vi "PIV_Stats_Single_with_Check.vi"(0 "Data Folder":path=path "C:/Users/PIV/Documents/mike_ensight/NACA0015_MB_G/15ms_PLANE_B_PA_300/rear", 1 "PIV Meas Plane":enum16{"XY", "YZ", "XZ"}(ring)=enum."XZ", 2 "Row number":i32=1, 5 "Output Directory":path=path "C:/Users/PIV/Documents/mike_ensight/NACA0015_MB_G/15ms_PLANE_B_PA_300/rear", 7 "XYZ Translation":dbl[](array[numeric])=[0.0, 0.0, 0.0], 9 "Case Name":string="ensight", 11 "PIV Freq (Hz)":dbl=7.25, 12 "Invert U":bool=TRUE, 13 "Invert V":bool, 14 "Kurt Tolerance":dbl=2.0) -> (4 "Progress Bar":i32(slide)=98 scale=0.0..100.0, 6 "Status":string="Wrting the data to file...", 10 "# total vectors":i32=10235)   [LabVIEW 2022 SP3]
uses:
  <vilib>/Utility/error.llb/DialogType.ctl
  <vilib>/Analysis/1siggen.llb/Ramp Pattern by Samples.vi
  <vilib>/Utility/error.llb/Trim Whitespace One-Sided.vi
  <vilib>/Analysis/NI_AALBase.lvlib
panel:
  out "interpolated vetors %":dbl[][](array[numeric])=[[15.76889236484505], [16.860635696821515], [16.77103718199609], [19.11750317972801], [17.901838091513493], [19.95502542041455], [17.47335484501809], [19.833822091886606], [17.568228504352927], [19.048084440969507], [19.503129890453835], [18.20848816741639], [19.704818688300264], [16.888323880305105], [18.985238048685112], [19.086731201720937], [19.43874058863792], [20.062603932309496], [18.812946123007723], [16.77097594367299], [18.17114914425428], [17.349232724073893], [20.437884859740006], [18.84596577017115], [17.522245037645447], [16.37484104470312], [17.813844348846306], [15.853300733496333], [17.204616588419405], [17.514179542343047], [17.895560336397416], [17.282502443792765], [19.48978594467794], [19.409406473061505], [15.101721439749607], [19.047153198982585], [20.273838630806846], [18.624669862075713], [16.686217008797655], [19.910033248582046], [17.447432762836186], [19.52292501710822], [18.057321725520882], [17.794290183809153], [18.836185819070906], [21.9538431449247], [19.12771367103462], [18.779342723004692], [19.080684596577015], [17.11324075884999], [18.96989835809226], [19.661712944857253], [17.548147423990613], [18.355173088206534], [19.303735575982788], [18.40226850493791], [19.730020541915287], [19.192412983965585], [15.809542432538132], [18.797066014669927], [16.179489686186333], [19.215724623508702], [20.629644114196324], [17.93116933906922], [21.66601486116543], [17.78973105134474], [18.141809290953546], [18.83987087938961], [17.193154034229828], [18.425427872860638], [19.253322908522282], [17.072455265473746], [19.196166634070018], [19.11189358372457], [19.732212666145426], [20.89566832893322], [19.980440097799512], [19.622604614782947], [19.311626087806786], [19.655779385879132], [16.301584197144532], [18.671752738654146], [15.97887737140622], [19.530562347188262], [19.66363547472377], [20.829664416397613], [16.601486116542823], [16.992760712189394], [17.893810501613377], [18.24581988853036], [17.78973105134474], [17.86098347834588], [17.78973105134474], [17.41001564945227], [17.850156494522693], [19.681267109894407], [18.73472181480395], [21.938575899843503], [19.033646322378715], [19.186387639350674], [17.31859964795619], [17.96752738654147], [19.69682151589242], [18.45115869756527], [19.102112676056336], [18.613067292644757], [17.709759436729904], [19.551815246110188], [17.30543605788033], [19.72809076682316], [16.93075117370892], [17.594132029339853], [17.77190923317684], [20.385217051231912], [19.26461959710542], [18.672401994329846], [19.91392801251956], [16.23154395228317], [17.58381389893461], [15.446280183791181], [18.061803246626244], [16.744868035190617], [18.525760093850817], [17.470409860119336], [18.382712427886965], [17.205982989539546], [15.335744306519402], [17.284554436075517], [19.13562139434829], [15.350019554165037], [17.535452322738386], [17.87775061124694], [18.39710343477835], [16.475994915419967], [18.69012707722385], [18.228046156855076], [18.21292403949555], [18.4841075794621], [16.744868035190617], [17.404908575339785], [16.477606102092704], [19.155177471399238], [16.891627543035995], [19.15330465389128], [15.395148669796557], [16.83129584352078], [15.180840664711631], [18.634451726499073], [15.529043614316448], [17.396831605710933], [16.927439859182474], [20.05475701574264], [19.317292644757433], [17.39853300733496], [17.240367690201445], [16.317950723504108], [19.3097379741885], [17.056234718826406], [19.3138500635324], [16.695992179863147], [16.347281971059836], [17.157390198571846], [17.117997849252127], [17.041454829878763], [17.015450811656564], [17.597028057483623], [17.059571554338255], [17.588971450919047], [18.4627420301193], [18.077825576847868], [17.58091326879828], [16.572154868987095], [19.052281182690425], [17.87775061124694], [17.80299325051355], [18.21826716213573], [18.3080684596577], [18.710876369327075], [19.27215809039327], [19.72051206879703], [19.921760391198042], [18.24403597966367], [19.72423234891453], [15.3199804592086], [16.674816625916872], [16.570534754130414], [17.03500880109525], [18.68583162217659], [16.901270772238515], [18.910726508262442], [17.408748409824838], [18.578273198396403], [17.970277669143528], [18.99872885499169], [21.344028171769537], [19.526742935367164], [21.466992665036674], [19.835680751173708], [16.83778234086242], [18.54712553773954], [17.253176930596286], [18.63147605083089], [18.648542929786817], [19.033646322378715], [17.03500880109525], [19.061124694376527], [17.418092909535453], [19.13562139434829], [18.521415998435362], [19.90804147916259], [17.784513101290575], [20.27185605319773], [16.47438404380133], [18.333822235259607], [17.155712050078247], [18.580089966751416], [18.459131795072352], [15.453834115805948], [17.59874853343762], [16.863934265871077], [17.800176142479696], [16.863818555088475], [17.311827956989248], [17.727583846680357], [17.946210268948658], [19.180760582657154], [19.683191551774716], [17.917888563049853], [20.86429409464216], [21.878971551471306], [15.705065519264618], [18.638763935067477], [18.72739712638061], [19.74982898465748], [18.00762537882491], [17.647058823529413], [17.874254424562434], [19.739802406338647], [18.43417065780471], [17.437200664646664], [17.852952678920612], [17.64360504941775], [17.750611246943766], [17.874254424562434], [17.916870415647924], [18.86976926085256], [17.11324075884999], [19.081133919843598], [16.035983181773737], [19.767214397496087], [18.37113805240516], [18.18092909535452], [17.330073349633253], [18.031665363565285], [21.255377395385217], [17.061008994915916], [18.806845965770172], [19.315403422982886], [18.615565115369574], [16.559076682316118], [17.602190494817133], [15.735941320293398], [19.3236242791516], [18.736553882260903], [17.475063563465675], [20.082127493156044], [17.285881892843175], [20.16428711128496], [16.264058679706604], [17.944455309994133], [18.732890105592492], [19.088151844242248], [19.34474327628362], [18.116933906922174], [19.14768839800606], [21.071673022391707], [16.199041939583537], [18.748166259168705], [19.50122249388753], [19.26049104959405], [16.738365271802895], [18.34001368657738], [19.061124694376527], [19.13562139434829], [19.585613760750586], [13.806590397966168], [17.269704674359478], [18.765890866418932], [17.905339331116764], [19.098376686876588], [19.888584831899923], [18.167595580326587], [19.346635367762126], [17.93743890518084], [18.859992178333982], [18.32225263981228], [17.175273865414713], [17.594132029339853], [21.550796910139827], [19.675337375317817], [19.9745795854517], [17.489490663799003], [17.597028057483623], [20.565225894778017], [17.530308955807588], [17.732160312805473], [17.74997556446095], [18.715165737753008], [19.61071987480438], [18.376528117359413], [19.511002444987774], [17.846665362800703], [17.036674816625915], [18.672401994329846], [17.70171149144254], [21.95718056506012], [18.378325508607197], [17.779298211318544], [18.45115869756527], [18.919976521228723], [20.117359413202934], [18.040481079495454], [16.73185996479562], [19.538431449247017], [18.728606356968218], [20.350259270130124], [19.403422982885086], [21.09122909944265], [18.34620271723194], [17.928403755868544], [18.18092909535452], [18.332029722330855], [19.943298465148107], [22.793470823966377], [18.34360027378508], [20.62762733405025], [18.61738535249829], [17.86098347834588], [17.132798748288675], [17.196206862840942], [21.914727166047328], [14.947697722162479], [15.304126735771561], [20.660995404321895], [19.66940532081377], [16.668296021116433], [15.213140398904967], [18.66379731976915], [18.029739776951672], [19.9745795854517], [18.912575787209075], [17.682151589242054], [17.44402072944167], [17.805808154884133], [19.692969590300187], [20.61008994915917], [20.428319968707218], [20.316932407316834], [20.152462861610633], [17.095354523227385], [19.796656564669078], [18.82145998240985], [18.58260019550342], [18.43417065780471], [17.052899188422803], [18.29113305308437], [16.335907713363966], [19.471882640586795], [18.873459808331702], [20.506799726054204], [20.774647887323944], [16.995892822217876], [17.378555370931483], [17.704565451168246], [19.362409544298846], [16.679702776691435], [17.47335484501809], [19.74572127139364], [19.206333691721237], [19.086731201720937], [18.099149310648283], [20.04304020346278], [17.628079780993353], [19.245061607666734], [20.81377151799687], [18.90279679248973], [17.227219397731716], [18.228046156855076], [19.75755205787467], [19.145399432873766], [18.90094846973697], [18.190709046454767], [19.178885630498534], [19.042033235581624], [17.743669957962656], [18.37473107764522], [17.963252541047694], [17.39853300733496], [18.413847056522588], [19.763348327791903], [18.490270851667155], [18.787286063569685], [20.867950346984653], [18.49281595151989], [16.904575674618695], [18.58372456964006], [18.274310311093718], [17.887530562347187], [19.69874804381847], [16.370037160179933], [18.66314347230378], [17.079135283184975], [19.534383253448105], [18.054740957966764], [20.440097799511005], [21.149335418295543], [17.499755453389415], [17.452092295658975], [18.888780201506407], [18.130256209661646], [19.249193469547365], [18.702924777462584], [17.767787333854574], [18.11069822022296], [16.555838059847446], [18.613745234138236], [19.497408819790753], [20.228783730934687], [17.86622335223939], [17.49633251833741], [20.891582754912505], [18.69743790338353], [18.560531977312735], [18.07158224134559], [21.411810715682442], [20.602327173169062], [20.312805474095796], [20.739219712525667], [17.956989247311828], [20.39898298454919], [18.723113023073914], [17.535452322738386], [16.753056234718827], [19.824046920821115], [18.035190615835777], [17.988073125427707], [19.87875232228415], [18.24139280125196], [18.715793588741203], [19.577340769004987], [20.41454829878764], [20.058651026392962], [19.9119804400978], [20.45387850924386], [19.552034428794993], [20.097751710654936], [17.038341158059467], [17.32499022291748], [18.571009676473462], [18.65401545534579], [20.035218156916454], [18.608746697974755], [18.689486552567235], [17.492910922069033], [17.35981994324298], [19.092331768388107], [17.507824726134587], [17.42105777690879], [18.456572769953052], [17.519319182236135], [20.583056153394637], [19.960899315738025], [17.404908575339785], [17.452092295658975], [17.77299833805846], [18.66875183266543], [20.156479217603913], [18.75794621026895], [17.165200391006845], [18.464547677261614], [16.239734063355495], [18.397887323943664], [18.585542404382274], [16.31774603795735], [18.59601095033242], [19.50909446508899], [19.61839530332681], [20.013694610192704], [17.93467631527479], [19.46781451770691], [18.842845973416733], [19.970660146699267], [19.661547490951776], [20.01173708920188], [17.32329650992277], [17.194525904203324], [18.394289067083903], [17.039788835663312], [18.974960876369327], [21.02589154860772], [17.850156494522693], [19.375978090766825], [19.976521228722362], [18.593505477308295], [19.558205454012313], [18.383719792583896], [17.42105777690879], [17.284554436075517], [20.357876210032266], [18.441380659039798], [17.685013197771042], [16.725352112676056], [17.999608916699255], [18.996380710163358], [17.113502935420744], [19.454225352112676], [17.900087985140285], [19.158924205378973], [19.244692300166324], [20.751026794445533], [16.903061723564512], [19.804496578690127], [18.955909668589303], [16.606321557882374], [16.823069403714566], [17.376856919468334], [18.418222700166194], [18.361360969886587], [18.68765890866419], [16.37484104470312], [16.754694835680752], [20.195599022004888], [19.405320813771517], [17.202933985330073], [16.927439859182474], [19.859196245233207], [22.610312102534], [17.74997556446095], [17.352624890018575], [18.286720125171133], [20.944558521560573], [20.0352009386917], [16.413968502396557], [18.96703511689328], [18.456572769953052], [19.466432131339783], [18.93716970052848], [20.36566288619476], [18.341806804849433], [17.438905180840663], [17.015450811656564], [16.47921760391198], [19.524833789597185], [20.952287837309346], [17.84492030898602], [17.970277669143528], [20.819880637902358], [18.754277891854894], [20.445878556761514], [17.774736018771996], [19.30596285434995], [18.083961248654468], [20.291414042636415], [21.10872115760657], [19.114196323816973], [17.74083129584352], [19.9041939583537], [18.413847056522588], [17.884032463087905], [20.316777473601878], [19.180760582657154], [19.319182236134207], [17.137550102649328], [18.688845401174166], [19.43276283618582], [17.962256771291678], [17.66718811106766], [18.811106765741105], [19.08904310429088], [18.918125794776483], [18.540973987874047], [18.228046156855076], [19.07463562555023], [18.894865525672373], [16.441837732160312], [18.448596302455247], [17.67523707107244], [17.79495206417531], [17.525672371638144], [20.217030012708964], [15.66536203522505], [20.88223787167449], [18.855745721271393], [17.196206862840942], [17.561357191747334], [16.916006649066198], [18.2200488997555], [17.900087985140285], [17.97906681013401], [17.561882398982487], [18.752444270629645], [16.528036011351404], [18.55438184663537], [18.778103616813294], [16.33750488854126], [20.3991781626064], [18.635119280406727], [19.05134474327628], [16.779114109709592], [18.947985921001173], [17.80058651026393], [19.86897428375868], [19.17245426978382], [18.552567237163814], [18.271580799687165], [20.39898298454919], [16.839428906708388], [17.947214076246336], [19.36840046929996], [19.741859782927545], [19.33118216485773], [17.87075960504448], [18.394289067083903], [16.552600703949942], [17.207665232694563], [16.554219223623743], [16.982792334767304], [20.39319248826291], [19.97653270753887], [16.314760508308897], [18.998239092154176], [20.4950107611035], [18.120477214942305], [20.73552425665102], [17.04312114989733], [17.134474327628364], [17.369193154034228], [20.232853928187065], [17.389177023192094], [15.833740831295842], [16.195599022004888], [19.107719401232757], [19.90414710485133], [18.320461433180174], [17.392154944732464], [18.744499853329422], [18.20492764958936], [17.336855493591624], [18.035190615835777], [17.944455309994133], [16.169713559487732], [17.334767305436056], [19.157050655192645], [16.687848274513637], [17.832338843783624], [17.58607198748044], [18.2920864716815], [17.725850606179115], [16.964896841693555], [13.423344095489679], [17.139503032674625], [17.230588695482105], [17.21744231521314], [17.748875415607277], [17.15067957367752], [17.93116933906922], [16.352262730915847], [16.65199960887846], [19.098376686876588], [17.804067266327728], [16.775897486060842], [18.155140369754474], [16.39921722113503], [18.191593352883675], [17.3657964212379], [18.539161044294513], [18.77750611246944], [18.68765890866419], [18.77750611246944], [17.962256771291678], [19.090909090909093], [15.611855619681112], [18.877151799687013], [16.977995110024448], [18.47432762836186], [20.25625978090767], [18.840438013296833], [18.73105875452146], [17.22754842496576], [19.66363547472377], [18.910726508262442], [18.490270851667155], [19.006648416112633], [18.720657276995308], [18.677879913944846], [17.549863120844737], [15.50880626223092], [18.96889062805713], [16.73349633251834], [16.1861010653895], [17.693661971830984], [18.190709046454767], [17.08866946915632], [15.605749486652979], [16.050469483568076], [18.646719468074703], [18.80258266484054], [18.431602620514326], [17.22586324953536], [15.487721357988454], [17.11324075884999], [17.751710654936463], [17.44402072944167], [18.501125134526955], [16.992952231793264], [17.659137577002053], [17.629803461425638], [15.108546841384706], [19.38196753373753], [18.052976248656044], [16.49555099247091], [17.792550591455665], [17.498043818466353], [20.03325833903942], [18.609426950909448], [18.11069822022296], [17.969284945710655], [17.721271393643033], [17.964013299432818], [18.754277891854894], [17.111567419575632], [19.78097193702943], [16.83129584352078], [19.231145456323976], [19.614556838192136], [18.47432762836186], [16.749779994133178], [17.825364231935072], [18.07252467989444], [16.052400039104505], [19.538431449247017], [17.541801114696394], [16.819960861056753], [16.311363191863876], [19.000097837784953], [16.412363067292645], [17.737990411897076], [17.23531136963535], [18.854461929430162], [21.517254863623034], [18.426197458455523], [17.667775386421443], [15.67726161369193], [16.955118803168084], [18.10623104763768], [18.682178121028446], [19.83770043019163], [20.40876197926853], [16.151740320688308], [16.314760508308897], [17.471646460696128], [20.04105973213413], [18.35337831231055], [19.09046454767726], [18.258234776659172], [20.41454829878764], [18.4627420301193], [17.98983183418068], [16.59986313422622], [18.249388753056234], [17.628079780993353], [16.454829878764176], [16.665035717780604], [17.531515684549987], [15.328181551403697], [18.447551080262002], [17.56479217603912], [20.778712580708277], [18.253813062182246], [19.14581704456607], [19.36840046929996], [17.58263250537845], [15.22589477801682], [17.96752738654147], [15.164254986312084], [19.19843597262952], [16.544441185098268], [18.894865525672373], [16.07858469357834], [17.616580310880828], [18.34360027378508], [18.81846635367762], [18.411269810213266], [15.996477839741708], [15.626833561509876], [16.7627797869221], [17.843175596402034], [20.119327073552427], [16.779114109709592], [19.27887434043385], [16.709034024247167], [18.114241001564945], [16.339102376063362], [18.195150567070787], [20.588235294117645], [19.27027291401741], [18.879546343371135], [16.59495403872482], [16.938715668067637], [18.670576735092865], [17.334767305436056], [16.757919436840048], [17.73562768869769], [17.466992665036674], [18.695609660702065], [16.995892822217876], [17.727583846680357], [16.808365093325516], [17.416389595149617], [17.59874853343762], [20.266040688575902], [19.375978090766825], [17.630368848449272], [17.205982989539546], [19.14768839800606], [16.625916870415647], [20.125171132407587], [17.597028057483623], [20.09190457567462], [18.07959323359734], [18.5721271393643], [17.95950308128729], [17.401505523511585], [19.65753424657534], [18.325836104048506], [16.357059053578414], [21.65412063740346], [18.282304607258144], [19.505279624560032], [19.252957856653953], [16.80031292783102], [17.87075960504448], [15.955781647427116], [19.775061124694375], [17.08390377469196], [18.63080684596577], [18.542787286063568], [18.710876369327075], [17.162135732446703], [18.853901818893018], [18.236041850004888], [18.461688819390147], [16.096225308038335], [20.391006842619745], [18.081361236064932], [16.933906922174423], [17.81451770690667], [17.197888150175988], [17.725850606179115], [17.284554436075517], [20.357876210032266], [17.97203480981715], [18.915745180546043], [16.2217659137577], [17.892780277832127], [17.45255331637644], [18.253813062182246], [16.850855745721272], [17.697644874425876], [18.369543942063025], [19.36399217221135], [18.188930177977706], [17.774736018771996], [15.708699902248288], [18.71699589282222], [16.321142186583216], [16.172875721130342], [16.709034024247167], [17.07102328311485], [18.332029722330855], [18.461688819390147], [17.75691796225677], [16.426964093532924], [17.600469345849223], [16.01642710472279], [17.194835680751176], [17.24340175953079], [18.01114696391904], [17.629803461425638], [19.927607121893953], [18.037757996674166], [18.345394093487187], [17.530308955807588], [17.851902572630344], [16.269065310911223], [18.517794290183808], [14.646069612827533], [18.236041850004888], [16.01642710472279], [18.581213307240706], [16.90774042220485], [17.44402072944167], [17.038341158059467], [16.619415387623423], [18.16849100860047], [16.357059053578414], [19.4759483770043], [21.434854852898056], [18.054740957966764], [19.814271749755623], [17.248801487134333], [19.36840046929996], [16.80680484943293], [18.79890453834116], [15.502738654147105], [17.72411770456545], [20.832925994720892], [19.215724623508702], [18.437774953563398], [20.22504892367906], [15.943304007820135], [17.95774647887324], [18.707216898102875], [19.072769953051644], [17.517605633802816], [18.599647956190104], [18.03246626246822], [19.469978486211616], [17.83059467918623], [18.87585532746823], [18.566679702776693], [19.590958019375673], [18.881392392686028], [20.667057902973397], [20.26392961876833], [20.91113500830971], [17.414686613865257], [18.947471388046562], [17.49633251833741], [17.22586324953536], [18.195150567070787], [19.636221396440444], [18.10800234787713], [18.89301779777039], [18.464547677261614], [19.096509240246405], [17.48826291079812], [16.839428906708388], [17.34793663211422], [17.718921032056294], [18.498240125146655], [17.93366598180217], [20.150567070786078], [22.345002933698417], [19.387954634337117], [17.728694292415952], [18.726152039917814], [19.282291972230368], [20.502787831360656], [19.64809384164223], [19.299960891669926], [17.835142270460548], [18.464547677261614], [16.74491392801252], [15.907313257723896], [21.59546387721185], [18.93213377664776], [18.49643171375501], [20.39898298454919], [20.553436980541704], [16.891627543035995], [15.97419102551569], [18.38810641627543], [19.90804147916259], [17.341153470185727], [18.2200488997555], [17.832338843783624], [19.978486211617447], [17.295658975361754], [15.711771607352365], [18.327628361858192], [16.658515112980535], [19.41510172143975], [19.078818697437903], [17.002543533555077], [18.133802816901408], [18.982885085574573], [18.548939082819988], [18.274310311093718], [18.00841240340409], [18.190709046454767], [18.38091513492374], [17.831655098250074], [18.174704098601193], [20.766523269456393], [18.657154026583267], [18.019163081736412], [18.08312958435208], [17.59241150009779], [17.400234741784036]]
  out "bad vectors %":dbl[][](array[numeric])=[[0.009776126698602014], [0.15647921760391198], [0.12720156555772996], [0.1858917914098425], [0.04888541259288229], [0.04888541259288229], [0.048890192627358955], [0.04887585532746823], [0.1271642375036682], [0.039093041438623924], [0.21517996870109546], [0.18580089966751417], [0.1466132342879484], [0.15646391550948563], [0.22485091406784632], [0.048890192627358955], [0.10755842378018969], [0.04890932211679546], [0.19556077050943582], [0.09778994719342853], [0.254278728606357], [0.029322646857589677], [0.17593588114553807], [0.0684596577017115], [0.14667057788207685], [0.04890932211679546], [0.03910833007430582], [0.058679706601467], [0.029342723004694836], [0.2249168785448856], [0.11734793663211421], [0.13685239491691104], [0.10751637181116215], [0.06844626967830253], [0.18583724569640062], [0.17609078458227354], [0.10757946210268948], [0.17607355962046367], [0.4594330400782014], [0.07823195775474281], [0.0684596577017115], [0.29328380095806045], [0.14672796635038637], [0.1564333202972233], [0.08801955990220049], [0.2835908468609427], [0.19557989438685705], [0.09780907668231612], [0.058679706601467], [0.10756894191277137], [0.029319781078967946], [0.09777082518576458], [0.05865676019161209], [0.07823195775474281], [0.2542538627029141], [0.05866823115283074], [0.19563728846718184], [0.08799374266718811], [0.14665623777864686], [0.31295843520782396], [0.09776126698602015], [0.18580089966751417], [0.06843957763003519], [0.17598748533437622], [0.03910833007430582], [0.24449877750611246], [0.18581907090464547], [0.20541915289054094], [0.04889975550122249], [0.1466992665036675], [0.13682564503518374], [0.05866823115283074], [0.019557989438685704], [0.0782472613458529], [0.1563721657544957], [0.10755842378018969], [0.009779951100244499], [0.09777082518576458], [0.09778038525471791], [0.3422648151769998], [0.07823195775474281], [0.029342723004694836], [0.009778994719342852], [0.26405867970660146], [0.07822430820377432], [0.13697289893356815], [0.3030895580758702], [0.019565642731363724], [0.07822430820377432], [0.05866823115283074], [0.04889975550122249], [0.29328380095806045], [0.0293398533007335], [0.08802816901408451], [0.09780907668231612], [0.19554165037152915], [0.02933411557641537], [0.09780907668231612], [0.13693270735524257], [0.09778994719342853], [0.37160179933502835], [0.13693270735524257], [0.08801955990220049], [0.0880023467292461], [0.14671361502347416], [0.03912363067292645], [0.06845296303539997], [0.17614247969468638], [0.01955416503715291], [0.19561815336463223], [0.009780907668231613], [0.19559902200488996], [0.03912363067292645], [0.06843957763003519], [0.058673968316057104], [0.10753739368462216], [0.35211267605633806], [0.12711450083113326], [0.20525852800312777], [0.17597028057483624], [0.27381185214159987], [0.19550342130987292], [0.43014957473848864], [0.1173823730803091], [0.048890192627358955], [0.14664190047903022], [0.0977421561919656], [0.019563728846718184], [0.048890192627358955], [0.14665623777864686], [0.019559902200488997], [0.0293398533007335], [0.18592817301105782], [0.048890192627358955], [0.05865102639296188], [0.019557989438685704], [0.08798514028741812], [0.09779951100244498], [0.1270772238514174], [0.02933411557641537], [0.04889497359671426], [0.3324533098660409], [0.04890453834115806], [0.1564333202972233], [0.0], [0.0293398533007335], [0.07820136852394917], [0.2641103394306955], [0.17602190494817133], [0.08801095247408566], [0.23469587326422842], [0.10755842378018969], [0.09780907668231612], [0.039119804400977995], [0.2444748679835713], [0.0], [0.0], [0.07823960880195599], [0.1368390186687518], [0.08797653958944282], [0.0], [0.15650983077374547], [0.1955225339720403], [0.009777082518576456], [0.04889497359671426], [0.05865676019161209], [0.029345593270077276], [0.18576456785295267], [0.12712693135145706], [0.05866249511145874], [0.28356311723868194], [0.19554165037152915], [0.10769532014881535], [0.1271393643031785], [0.06847305096351364], [0.10756894191277137], [0.18581907090464547], [0.019561815336463225], [0.16630796321659166], [0.0977230528681716], [0.04889975550122249], [0.09777082518576458], [0.08801095247408566], [0.039081582804103565], [0.0684596577017115], [0.10753739368462216], [0.2249168785448856], [0.16622665493302044], [0.16617790811339198], [0.22489488608585118], [0.03914277326548586], [0.10755842378018969], [0.02933124755572937], [0.07822430820377432], [0.15650983077374547], [0.03911215410188716], [0.09779951100244498], [0.10758998435054773], [0.24445096313679476], [0.18576456785295267], [0.04887585532746823], [0.13685239491691104], [0.16624291022882848], [0.08802816901408451], [0.04889497359671426], [0.1271393643031785], [0.117359413202934], [0.03911215410188716], [0.058673968316057104], [0.20543924867931912], [0.07821666014861164], [0.07823195775474281], [0.18576456785295267], [0.09778038525471791], [0.09780907668231612], [0.19557989438685705], [0.14665623777864686], [0.0], [0.04888541259288229], [0.04890932211679546], [0.1076426264800861], [0.0], [0.0], [0.05866823115283074], [0.15647921760391198], [0.21507478736924432], [0.30311919428962547], [0.1466275659824047], [0.19554165037152915], [0.14664190047903022], [0.058673968316057104], [0.27381185214159987], [0.0684195093343759], [0.3420306850386006], [0.30305992765666245], [0.11745130664578643], [0.05866823115283074], [0.20541915289054094], [0.1954843123839312], [0.0], [0.02933124755572937], [0.07828554653097172], [0.117359413202934], [0.13689253935660506], [0.1271393643031785], [0.04888541259288229], [0.3227068257383141], [0.20527859237536658], [0.13689253935660506], [0.12715179968701096], [0.05866249511145874], [0.20537897310513448], [0.28361858190709044], [0.2052384675527756], [0.07821666014861164], [0.09777082518576458], [0.019559902200488997], [0.19559902200488996], [0.03910833007430582], [0.12715179968701096], [0.06845296303539997], [0.1271393643031785], [0.1368390186687518], [0.21513788382554275], [0.009778994719342852], [0.04888541259288229], [0.09777082518576458], [0.08801095247408566], [0.117359413202934], [0.13690592607079993], [0.10754790770434103], [0.2348106838861168], [0.019559902200488997], [0.01955416503715291], [0.08796794057276904], [0.26400704018773835], [0.16619415387623424], [0.09779951100244498], [0.1662591687041565], [0.06847305096351364], [0.14665623777864686], [0.11731352038322418], [0.0684596577017115], [0.12711450083113326], [0.009773260359655981], [0.10755842378018969], [0.07823195775474281], [0.14668492079014278], [0.09778994719342853], [0.14668492079014278], [0.019546520719311962], [0.22489488608585118], [0.03912363067292645], [0.13685239491691104], [0.06843957763003519], [0.29331247555729373], [0.1564945226917058], [0.136919315403423], [0.25422900166226653], [0.009778994719342852], [0.10754790770434103], [0.2052986606706423], [0.03910450679440806], [0.03911597887737141], [0.0], [0.09775171065493646], [0.11729058743035871], [0.14667057788207685], [0.30320813771517996], [0.04889975550122249], [0.019559902200488997], [0.17602190494817133], [0.04889975550122249], [0.15641802717763223], [0.117359413202934], [0.029328380095806045], [0.04890453834115806], [0.03909686247678624], [0.05866823115283074], [0.03913128546272745], [0.058679706601467], [0.21511684756037938], [0.04889497359671426], [0.23469587326422842], [0.09779951100244498], [0.1174053419430584], [0.0684596577017115], [0.24445096313679476], [0.01954843123839312], [0.1662754303599374], [0.273838630806846], [0.21509581540868206], [0.2052986606706423], [0.15638744990714495], [0.09778038525471791], [0.07820901358881611], [0.05866823115283074], [0.29328380095806045], [0.07823195775474281], [0.21507478736924432], [0.13690592607079993], [0.05865676019161209], [0.08801095247408566], [0.048890192627358955], [0.12715179968701096], [0.23462704076644836], [0.04888541259288229], [0.07825491538687274], [0.04891410682840931], [0.05866249511145874], [0.12712693135145706], [0.1271393643031785], [0.0880023467292461], [0.11733646230566148], [0.20533880903490762], [0.02933124755572937], [0.29336984158028556], [0.17607355962046367], [0.07818608287724785], [0.1662591687041565], [0.23462704076644836], [0.08795074758135445], [0.09775171065493646], [0.2639038217183071], [0.09778038525471791], [0.12708964708182618], [0.05865676019161209], [0.136919315403423], [0.029336984158028552], [0.10762156344780353], [0.019561815336463225], [0.058673968316057104], [0.03909686247678624], [0.12708964708182618], [0.2444748679835713], [0.13687915526007038], [0.1760046934584922], [0.04889975550122249], [0.18571009676473463], [0.11733646230566148], [0.2737850787132101], [0.04890932211679546], [0.09777082518576458], [0.23469587326422842], [0.009780907668231613], [0.10756894191277137], [0.1564333202972233], [0.15646391550948563], [0.11731352038322418], [0.02933411557641537], [0.26400704018773835], [0.019559902200488997], [0.04887585532746823], [0.5474095796676441], [0.05865676019161209], [0.14668492079014278], [0.11727912431587179], [0.10757946210268948], [0.019557989438685704], [0.019557989438685704], [0.05866823115283074], [0.43031784841075793], [0.03909686247678624], [0.07819372495357248], [0.08799374266718811], [0.09780907668231612], [0.06847974955977304], [0.293398533007335], [0.009780907668231613], [0.2249168785448856], [0.21530632217655118], [0.019563728846718184], [0.05869118654015455], [0.009775171065493646], [0.04889975550122249], [0.2052384675527756], [0.08803677981023184], [0.03910833007430582], [0.14672796635038637], [0.019557989438685704], [0.1955225339720403], [0.14672796635038637], [0.13682564503518374], [0.04889497359671426], [0.21513788382554275], [0.2052986606706423], [0.06844626967830253], [0.19554165037152915], [0.2249168785448856], [0.24449877750611246], [0.03910450679440806], [0.16624291022882848], [0.20535888910619987], [0.009778994719342852], [0.23464998044583496], [0.16622665493302044], [0.1270772238514174], [0.05866823115283074], [0.11730205278592376], [0.16624291022882848], [0.18576456785295267], [0.1662591687041565], [0.35207823960880197], [0.08797653958944282], [0.3812316715542522], [0.03910450679440806], [0.14667057788207685], [0.44992175273865415], [0.07818608287724785], [0.15654045592407786], [0.07821666014861164], [0.17595307917888564], [0.136919315403423], [0.06847305096351364], [0.04890453834115806], [0.24437927663734116], [0.27386541471048514], [0.1564333202972233], [0.2639038217183071], [0.1271642375036682], [0.019565642731363724], [0.0293513354857646], [0.09779951100244498], [0.15644861640754865], [0.08807123984734319], [0.009780907668231613], [0.10758998435054773], [0.08798514028741812], [0.19561815336463223], [0.019563728846718184], [0.14674232048522795], [0.21505376344086022], [0.10755842378018969], [0.07821666014861164], [0.15641802717763223], [0.10751637181116215], [0.09779951100244498], [0.1271393643031785], [0.09775171065493646], [0.039119804400977995], [0.02933124755572937], [0.11737089201877934], [0.2543284750073364], [0.0782625709254549], [0.04888541259288229], [0.12712693135145706], [0.029354207436399216], [0.30323779712413185], [0.11734793663211421], [0.2543533555077284], [0.14659890539483972], [0.24449877750611246], [0.1271642375036682], [0.13693270735524257], [0.10753739368462216], [0.17595307917888564], [0.08801095247408566], [0.08798514028741812], [0.1662754303599374], [0.14655593551538837], [0.1662754303599374], [0.1564945226917058], [0.05869692819409117], [0.11737089201877934], [0.058645293715179354], [0.07827022796203893], [0.17597028057483624], [0.09781864423359092], [0.048890192627358955], [0.13689253935660506], [0.08798514028741812], [0.04890453834115806], [0.2248728979272585], [0.21520101731390004], [0.08806262230919766], [0.10758998435054773], [0.08798514028741812], [0.10757946210268948], [0.09783778495254868], [0.04889497359671426], [0.03912745769343637], [0.09775171065493646], [0.009776126698602014], [0.1369997064292005], [0.1466275659824047], [0.06841282251759187], [0.03910450679440806], [0.20531873289010558], [0.19557989438685705], [0.13694610192702728], [0.029342723004694836], [0.1466992665036675], [0.14671361502347416], [0.0684596577017115], [0.11734793663211421], [0.05866823115283074], [0.1858917914098425], [0.0977421561919656], [0.2835076742594584], [0.13690592607079993], [0.39112154101887164], [0.40089957954434335], [0.14672796635038637], [0.1173823730803091], [0.19561815336463223], [0.0977230528681716], [0.07829320806420043], [0.3030895580758702], [0.10754790770434103], [0.13685239491691104], [0.14668492079014278], [0.09779951100244498], [0.11732499022291748], [0.12710207274149393], [0.185782731983964], [0.009777082518576456], [0.5381078172390177], [0.06844626967830253], [0.19556077050943582], [0.16621040281579977], [0.19550342130987292], [0.07828554653097172], [0.17602190494817133], [0.21509581540868206], [0.10754790770434103], [0.04889975550122249], [0.30305992765666245], [0.30314883629962835], [0.05866823115283074], [0.25420414548298786], [0.14664190047903022], [0.10760050865695002], [0.09776126698602015], [0.09784735812133072], [0.22493887530562348], [0.0880023467292461], [0.12710207274149393], [0.10754790770434103], [0.12706480304955528], [0.1173823730803091], [0.19557989438685705], [0.14668492079014278], [0.009781864423359092], [0.0293398533007335], [0.08797653958944282], [0.009781864423359092], [0.1955225339720403], [0.1565251418509098], [0.019559902200488997], [0.09776126698602015], [0.1076320939334638], [0.3129890453834116], [0.15647921760391198], [0.08798514028741812], [0.1760046934584922], [0.02933411557641537], [0.0684596577017115], [0.2052986606706423], [0.019563728846718184], [0.2054593484003522], [0.10754790770434103], [0.029357079949114396], [0.12715179968701096], [0.23460410557184752], [0.04888541259288229], [0.019567556990509733], [0.2835353930387172], [0.15647921760391198], [0.03911215410188716], [0.24442706296441144], [0.10752688172043011], [0.06844626967830253], [0.05869118654015455], [0.058679706601467], [0.04888063349301008], [0.2444748679835713], [0.0], [0.05865102639296188], [0.18576456785295267], [0.34223134839151265], [0.1760046934584922], [0.10753739368462216], [0.11734793663211421], [0.35197497066875244], [0.04888541259288229], [0.06844626967830253], [0.07821666014861164], [0.19561815336463223], [0.1760046934584922], [0.08797653958944282], [0.22500489141068286], [0.09782821365681862], [0.20535888910619987], [0.39123630672926446], [0.13689253935660506], [0.0293398533007335], [0.039119804400977995], [0.009783778495254867], [0.26421371954202955], [0.117359413202934], [0.04889975550122249], [0.0587026709715292], [0.08802816901408451], [0.23462704076644836], [0.04890932211679546], [0.0880023467292461], [0.0], [0.34243224733392036], [0.37145650048875856], [0.029336984158028552], [0.11731352038322418], [0.05866249511145874], [0.03911597887737141], [0.09776126698602015], [0.15650983077374547], [0.019561815336463225], [0.15650983077374547], [0.3226437231130231], [0.05866823115283074], [0.0], [0.029348464097045585], [0.0], [0.10754790770434103], [0.16624291022882848], [0.20533880903490762], [0.03910833007430582], [0.1954843123839312], [0.10755842378018969], [0.12712693135145706], [0.02933124755572937], [0.07825491538687274], [0.06847305096351364], [0.14677103718199608], [0.1466275659824047], [0.02933411557641537], [0.11733646230566148], [0.08801955990220049], [0.09778994719342853], [0.08801955990220049], [0.048890192627358955], [0.039100684261974585], [0.18585542404382277], [0.09780907668231612], [0.1271393643031785], [0.058679706601467], [0.09780907668231612], [0.27375831052014077], [0.24440316746505036], [0.09782821365681862], [0.06844626967830253], [0.01955607705094358], [0.07822430820377432], [0.21509581540868206], [0.08802816901408451], [0.10756894191277137], [0.06843957763003519], [0.03913894324853229], [0.04891410682840931], [0.17603911980440098], [0.18571009676473463], [0.19561815336463223], [0.0684596577017115], [0.07820901358881611], [0.07822430820377432], [0.10758998435054773], [0.20533880903490762], [0.18587360594795538], [0.07822430820377432], [0.08803677981023184], [0.28372957636239116], [0.10756894191277137], [0.20527859237536658], [0.12711450083113326], [0.0880540064572938], [0.07830853563038372], [0.22489488608585118], [0.10755842378018969], [0.04889497359671426], [0.07823195775474281], [0.058645293715179354], [0.0880023467292461], [0.12708964708182618], [0.06846635367762129], [0.08803677981023184], [0.04889497359671426], [0.10756894191277137], [0.2445466105839773], [0.019559902200488997], [0.13690592607079993], [0.0], [0.05866823115283074], [0.23467292461132297], [0.15647921760391198], [0.05869118654015455], [0.13695949911954608], [0.0293398533007335], [0.11733646230566148], [0.03911215410188716], [0.03909686247678624], [0.10753739368462216], [0.058673968316057104], [0.03911215410188716], [0.05870841487279843], [0.04889497359671426], [0.3913511398101947], [0.05868544600938967], [0.019567556990509733], [0.0684328868902141], [0.12706480304955528], [0.14664190047903022], [0.09775171065493646], [0.06847974955977304], [0.019559902200488997], [0.06844626967830253], [0.0], [0.01955225339720403], [0.03910833007430582], [0.10756894191277137], [0.03910833007430582], [0.04887585532746823], [0.20531873289010558], [0.05865676019161209], [0.0880023467292461], [0.117359413202934], [0.10751637181116215], [0.17598748533437622], [0.029336984158028552], [0.08799374266718811], [0.11731352038322418], [0.0293398533007335], [0.10754790770434103], [0.1564333202972233], [0.12721401311282904], [0.13681227401544024], [0.13694610192702728], [0.12708964708182618], [0.019559902200488997], [0.09782821365681862], [0.04888541259288229], [0.13682564503518374], [0.14665623777864686], [0.09778994719342853], [0.019557989438685704], [0.22496087636932707], [0.05866249511145874], [0.1270772238514174], [0.15644861640754865], [0.117359413202934], [0.0], [0.0], [0.22489488608585118], [0.06846635367762129], [0.0782625709254549], [0.0587026709715292], [0.10756894191277137], [0.1466132342879484], [0.14665623777864686], [0.1564945226917058], [0.13689253935660506], [0.048856752003126835], [0.09777082518576458], [0.11737089201877934], [0.10755842378018969], [0.18576456785295267], [0.13679890560875513], [0.029345593270077276], [0.11732499022291748], [0.06845296303539997], [0.01954843123839312], [0.08797653958944282], [0.07821666014861164], [0.12710207274149393], [0.08799374266718811], [0.04889975550122249], [0.048890192627358955], [0.20535888910619987], [0.0880023467292461], [0.10749535815498877], [0.3618228046156855], [0.08799374266718811], [0.3423317683881064], [0.05868544600938967], [0.07827022796203893], [0.08798514028741812], [0.1954843123839312], [0.08801955990220049], [0.20535888910619987], [0.05865676019161209], [0.11732499022291748], [0.05866823115283074], [0.04889975550122249], [0.13694610192702728], [0.1368657737804282], [0.23483365949119372], [0.18580089966751417], [0.16621040281579977], [0.31283605435526446], [0.05869118654015455], [0.04888541259288229], [0.05866823115283074], [0.21513788382554275], [0.03910450679440806], [0.1271766777538642], [0.1466992665036675], [0.14668492079014278], [0.1662591687041565], [0.117359413202934], [0.3227699530516432], [0.019557989438685704], [0.18580089966751417], [0.02933411557641537], [0.3029710711493354], [0.058673968316057104], [0.11730205278592376], [0.10756894191277137], [0.14665623777864686], [0.19565642731363725], [0.09777082518576458], [0.16621040281579977], [0.04890932211679546], [0.12711450083113326], [0.11733646230566148], [0.029357079949114396], [0.00977803852547179], [0.03913128546272745], [0.04891410682840931], [0.0], [0.15647921760391198], [0.16612918987589173], [0.23487962419260128], [0.03913894324853229], [0.13690592607079993], [0.0], [0.02932551319648094], [0.04889497359671426], [0.0], [0.07822430820377432], [0.04888541259288229], [0.1565251418509098], [0.05866249511145874], [0.1563721657544957], [0.06844626967830253], [0.19567556990509735], [0.10755842378018969], [0.19556077050943582], [0.08802816901408451], [0.06842619745845552], [0.07822430820377432], [0.32267527134056906], [0.20543924867931912], [0.2249828817372591], [0.23469587326422842], [0.11732499022291748], [0.13694610192702728], [0.03910833007430582], [0.19554165037152915], [0.13687915526007038], [0.09778038525471791], [0.07822430820377432], [0.2054794520547945], [0.11727912431587179], [0.06844626967830253], [0.0782472613458529], [0.17597028057483624], [0.08795934323690383], [0.11732499022291748], [0.01955416503715291], [0.1661616655263415], [0.019550342130987292], [0.06842619745845552], [0.009783778495254867], [0.14665623777864686], [0.41063746578021115], [0.03912363067292645], [0.09780907668231612], [0.029328380095806045], [0.029328380095806045], [0.11734793663211421], [0.07820901358881611], [0.04892367906066536], [0.22482893450635386], [0.10758998435054773], [0.264032857422257], [0.08802816901408451], [0.05868544600938967], [0.12712693135145706], [0.04889497359671426], [0.09778994719342853], [0.019561815336463225], [0.019550342130987292], [0.21509581540868206], [0.05871415989822879], [0.07822430820377432], [0.4694835680751174], [0.039100684261974585], [0.08798514028741812], [0.30311919428962547], [0.03912745769343637], [0.21515892420537897], [0.09781864423359092], [0.16621040281579977], [0.10756894191277137], [0.20543924867931912], [0.19557989438685705], [0.058679706601467], [0.10755842378018969], [0.2445226917057903], [0.029336984158028552], [0.17602190494817133], [0.009773260359655981], [0.08799374266718811], [0.009783778495254867], [0.09777082518576458], [0.3227068257383141], [0.21509581540868206], [0.0], [0.0587026709715292], [0.28356311723868194], [0.07825491538687274], [0.009775171065493646], [0.04888541259288229], [0.13689253935660506], [0.08801955990220049], [0.0], [0.009777082518576456], [0.04888063349301008], [0.16624291022882848], [0.11731352038322418], [0.2542538627029141], [0.24445096313679476], [0.04890453834115806], [0.03910450679440806], [0.35211267605633806], [0.13695949911954608], [0.1466275659824047], [0.09779951100244498], [0.03912745769343637], [0.019557989438685704], [0.3226437231130231], [0.21509581540868206], [0.039119804400977995], [0.04890932211679546], [0.18583724569640062], [0.2542538627029141], [0.13695949911954608], [0.14671361502347416], [0.058679706601467], [0.01955607705094358], [0.215222070045001], [0.16629169519710454], [0.20537897310513448], [0.01955416503715291], [0.2052986606706423], [0.029345593270077276], [0.10754790770434103], [0.11727912431587179], [0.06843957763003519], [0.3422982885085574], [0.06845296303539997], [0.1662754303599374]]
  out "good vectors %":dbl[][](array[numeric])=[[84.22133150845636], [82.98288508557458], [83.10176125244618], [80.69660502886215], [82.04927649589364], [79.99608916699256], [82.47775496235455], [80.11730205278592], [82.3046072581434], [80.91282251759186], [80.28169014084507], [81.6057109329161], [80.14856807741178], [82.95521220418541], [80.78991103724704], [80.86437860565171], [80.45370098758188], [79.8884867455737], [80.99149310648284], [83.13123410913357], [81.57457212713936], [82.62144462906852], [79.38617925911446], [81.08557457212714], [82.33108438447248], [83.57624963318008], [82.1470473210794], [84.08801955990221], [82.7660406885759], [82.26090357911207], [81.98709172697046], [82.58064516129032], [80.4026976835109], [80.52214725726019], [84.71244131455398], [80.77675601643513], [79.61858190709047], [81.19925657830382], [82.85434995112414], [80.01173479366321], [82.4841075794621], [80.18379118193371], [81.79595030812872], [82.04927649589364], [81.0757946210269], [77.76256600821435], [80.67670643457852], [81.12284820031299], [80.86063569682152], [82.77919029923724], [81.00078186082878], [80.24051622995698], [82.39319581581778], [81.56659495403873], [80.44201056131429], [81.53906326390926], [80.07434216961752], [80.71959327336722], [84.04380132968322], [80.88997555012224], [83.72274904682764], [80.59847447682378], [79.30191630817363], [81.8928431755964], [78.29487680876026], [81.96577017114915], [81.67237163814181], [80.95470996771985], [82.75794621026895], [81.4278728606357], [80.60985144644253], [82.86887650337343], [80.7842753764913], [80.80985915492957], [80.11141516810008], [78.99677324728658], [80.00977995110024], [80.27962456003128], [80.59059352693849], [80.00195579894387], [83.62018384510073], [81.29890453834115], [84.01134363387443], [80.20537897310514], [80.25814021707247], [79.03336268466882], [83.0954243253813], [82.98767364507924], [82.02796519018285], [81.6955118803168], [82.16136919315403], [81.84573272069606], [82.18092909535453], [82.50195618153364], [82.052034428795], [80.12319123973406], [81.23594406961963], [77.96361502347418], [80.82942097026604], [80.7158224134559], [82.30979855270878], [81.89553990610328], [80.21515892420538], [81.46083895570548], [80.75117370892019], [81.34780907668232], [82.22178760023469], [80.27204227419513], [82.67500977708252], [80.07629107981221], [83.05946791862286], [82.21026894865525], [82.18896713615024], [79.54634337113805], [80.67670643457852], [81.22006061198553], [79.7339593114241], [83.6413415468857], [82.21092757306226], [84.37774953563398], [81.66438490123215], [83.05962854349951], [81.04409033141069], [82.41220776680035], [81.56839737948567], [82.64737510998143], [84.56651353728863], [82.69588183507777], [80.81548841302435], [84.50332420805631], [82.44498777506112], [82.09290953545232], [81.41696839221059], [83.47511489195267], [81.25122189638319], [81.75239585370623], [81.69909082021704], [81.41809290953546], [83.12805474095796], [82.56575730908379], [83.47349892431059], [80.51236921873472], [83.05946791862286], [80.69026202581149], [84.60485133020345], [83.13936430317848], [84.74095796676441], [81.10143793407023], [84.29493448073538], [82.51515744181498], [82.8378642675533], [79.83768456047717], [80.58489827856025], [82.56234718826406], [82.51515744181498], [83.68204927649589], [80.69026202581149], [82.86552567237165], [80.54931091779885], [83.21603128054741], [83.65271802894017], [82.6860999706544], [82.68647961677583], [82.94876808760266], [82.93565421474672], [82.34431518232476], [82.91108285239167], [82.225263981228], [81.41013103852924], [81.86351192804068], [82.13552361396303], [83.23230348064138], [80.84002349716076], [81.99511002444989], [82.12853369852294], [81.6741638959515], [81.50611246943765], [81.26956181533646], [80.56153394639014], [80.1817648783348], [80.02933985330073], [81.65819319515056], [80.18775669861138], [84.64093795798729], [83.25672371638142], [83.32192785218496], [82.74007432035987], [81.1479417228904], [82.9325513196481], [80.86437860565171], [82.55210881690968], [81.3141683778234], [82.00039108330074], [80.92304683680453], [78.4994619974567], [80.43414491053095], [78.43520782396088], [80.05672926447575], [82.91776669600078], [81.26710989440751], [82.69794721407625], [81.23167155425219], [81.18521415998435], [80.87832550860719], [82.91609622530804], [80.8117359413203], [82.4645476772616], [80.82526645154982], [81.41991003324858], [79.88651927215808], [82.13727023856082], [79.64991198904752], [83.33985138834572], [81.56839737948567], [82.74647887323944], [81.22433013886172], [81.394211967149], [84.54616588419405], [82.35236605396949], [83.08715641201213], [82.09218123104021], [83.13618144491153], [82.68817204301075], [82.21374792216682], [81.89731051344744], [80.60416462997361], [80.01368925393567], [81.93548387096774], [78.94016425498631], [77.97438654804967], [84.23626051241932], [81.08742421279092], [81.20418336428502], [79.90814033030392], [81.68931469351844], [82.2354898698248], [82.06707734428474], [80.05477844077082], [81.37034502981135], [82.56279933535335], [82.11771607352367], [82.27810940405128], [82.13202933985329], [81.98885303608097], [81.9559902200489], [81.08134532655455], [82.5640524154117], [80.71358748778104], [83.82712427886966], [80.1056338028169], [81.57019945248338], [81.61369193154034], [82.38630806845966], [81.76309616888194], [78.66640594446616], [82.84122017989833], [81.17359413202934], [80.48899755501222], [81.34532655455612], [83.31377151799687], [82.32935654214747], [84.13691931540342], [80.53953670217965], [81.04830823391356], [82.51515744181498], [79.86898709425108], [82.61634728197106], [79.74770193624096], [83.61858190709046], [81.91863876393506], [81.15956198670317], [80.67703747187164], [80.6356968215159], [81.86351192804068], [80.76434366142117], [78.66431993742056], [83.63476390654023], [81.15403422982885], [80.33251833740832], [80.67103589944243], [83.11497849041845], [81.5426727930394], [80.87041564792176], [80.73726410482057], [80.40461297888976], [86.08585117825365], [82.65206336788579], [81.08742421279092], [81.9968707216898], [80.75493839233326], [80.09186864738076], [81.60750953358756], [80.61424100156495], [81.92570869990224], [81.07156824403597], [81.38443488463042], [82.66823161189359], [82.26894865525672], [78.19497408819791], [80.31488362996284], [79.91787250684396], [82.30521067553036], [82.36386743572197], [79.39565812634461], [82.46969104419242], [82.17008797653959], [82.13273384810869], [81.13816368436491], [80.08607198748044], [81.57457212713936], [80.46943765281173], [81.97731273225114], [82.91442542787286], [81.17117997849252], [82.18092909535453], [78.01349105484408], [81.57276995305163], [82.18160492620467], [81.4901730712819], [81.04089219330855], [79.8239608801956], [81.74440207294417], [83.21924506160767], [80.22687267748876], [81.17359413202934], [79.53233538792682], [80.5281173594132], [78.66431993742056], [81.63424885152966], [81.90532081377152], [81.54523227383864], [81.45287446226047], [79.85140287418126], [77.05014172612647], [81.5586193409602], [79.29416365236094], [81.32394641634887], [81.84573272069606], [82.78896929395658], [82.58871834978981], [77.94836690788188], [84.99364551764592], [84.60786231175436], [79.29011440305075], [80.20344287949922], [83.09707693811713], [84.73797418850215], [81.25794776484398], [81.92134611621992], [79.96675791943684], [80.96029728143947], [82.19070904645477], [82.46797692382908], [82.07685538281021], [80.1016916006649], [79.3605788032851], [79.2783101897125], [79.50699403306271], [79.76935105551212], [82.73838630806846], [79.96871639456448], [81.09058927000879], [81.31964809384165], [81.30192552047698], [82.84932042632248], [81.5817772998338], [83.60543552644442], [80.39119804400978], [81.09720320751028], [79.385578710498], [79.20579029733959], [82.94543320946607], [82.58234776659174], [82.16834490174992], [80.39311558771757], [83.1834180680485], [82.35064046152341], [80.20537897310514], [80.60795621151404], [80.7959323359734], [81.62706561063851], [79.90805047442042], [82.27414939382088], [80.52024251906904], [79.1764475743349], [80.9896342655975], [82.61634728197106], [81.61548992763544], [80.1251344217421], [80.82526645154982], [80.83504449007529], [81.78973105134475], [80.772238514174], [80.41055718475073], [82.19767328184572], [81.47858400156464], [81.91946833463643], [82.49388753056235], [81.56659495403873], [80.21709368276942], [81.45106091718002], [80.78239608801955], [79.09295279053856], [81.42899032352653], [83.00743058271411], [81.31846635367762], [81.65720993934652], [81.81907090464547], [80.2914710485133], [83.40504596127518], [81.12155020551967], [82.90130098796831], [80.40692556001173], [81.93548387096774], [79.51100244498778], [78.64542611415169], [82.41220776680035], [82.50879937426672], [80.96449183214321], [81.85018580089967], [80.5552839964806], [81.15034725618703], [82.09538702111024], [81.84040680618033], [83.229024056327], [81.18095610519113], [80.43414491053095], [79.57567461869378], [81.90885976921572], [82.25916870415648], [79.06931273829308], [81.13631918638764], [81.23410913358107], [81.91863876393506], [78.35353930387173], [79.23144617189791], [79.56011730205279], [79.20211205632151], [81.92570869990224], [79.43477410522199], [81.09112240907314], [82.29828850855746], [82.89486552567237], [80.08797653958945], [81.58357771260997], [81.97282236777788], [79.97457709983378], [81.30868544600939], [81.20602032838154], [80.26611877507092], [79.50723504106375], [79.76539589442815], [79.95110024449878], [79.47764843979263], [80.39906103286386], [79.65786901270772], [82.68779342723005], [82.5185764567853], [81.16508650180822], [81.21882030715054], [79.94521620035219], [81.36190196653948], [81.21271393643032], [82.35064046152341], [82.55210881690968], [80.89788732394366], [82.38458528951486], [82.49095708280379], [81.34780907668232], [82.46111708891715], [79.27020152612013], [79.82404692082112], [82.48753300088002], [82.46969104419242], [82.0705836347639], [81.2237317955234], [79.74572127139365], [81.11491442542787], [82.73704789833822], [81.49633251833741], [83.73093468908877], [81.48474178403757], [81.16012912061039], [83.60399139111719], [81.3551036370747], [80.36377860355955], [80.35225048923678], [79.68306759268316], [81.9479757480931], [80.27783212678537], [81.01055512118843], [79.78484107579462], [80.21128827154456], [79.85133020344288], [82.5691660963926], [82.62952101661779], [81.51769998044202], [82.87222602404927], [80.85876369327075], [78.8275525158769], [81.98356807511738], [80.46752738654148], [79.96478184308354], [81.28912363067292], [80.3831492522725], [81.53800997945406], [82.40297194251637], [82.61762691969089], [79.59323359734037], [81.4217268016036], [82.22700166194153], [83.22574334898279], [81.77551818537349], [80.78841827252275], [82.79843444227006], [80.43818466353677], [82.0119268745723], [80.73349633251834], [80.65746991488113], [79.20007823195776], [83.05781081874206], [80.09775171065495], [81.03431420471209], [83.25667873568842], [83.03030303030303], [82.55473025801408], [81.5426727930394], [81.4333202972233], [81.11676119694894], [83.48821285336984], [83.21596244131455], [79.65770171149144], [80.447965571205], [82.72860635696821], [82.95521220418541], [80.08213552361396], [77.20379610605616], [82.15228227934708], [82.36386743572197], [81.57637394875806], [78.66431993742056], [79.56389948176395], [83.43930353125306], [80.91558251002641], [81.34780907668232], [80.43584481579205], [80.98453709140732], [79.33124755572936], [81.55064528744622], [82.42424242424242], [82.8378642675533], [83.42298288508557], [80.35784122017989], [78.92061008994916], [81.96929695903002], [82.0199452483379], [78.64201154485862], [81.1772758384668], [79.35856067272906], [82.0590535784122], [80.49853372434018], [81.83775320481456], [79.53256405241541], [78.67618302698475], [80.77825576847869], [82.21026894865525], [79.79274611398964], [81.28300410717777], [82.05729930575927], [79.42901838091514], [80.67259751686382], [80.57321725520885], [82.76468863036465], [81.2133072407045], [80.34229828850856], [81.94974088197907], [82.20570981619085], [81.08134532655455], [80.78389209265956], [80.96449183214321], [81.2634461177391], [81.62526892235478], [80.91558251002641], [81.0757946210269], [83.47018572825024], [81.5416218331214], [82.12924039495552], [82.04852279397377], [82.45476772616136], [79.68520872030501], [84.22700587084148], [78.80477308294209], [80.9877750611247], [82.71580799687163], [82.26263811479417], [83.05465923535739], [81.71149144254278], [81.89461335418908], [82.00136946101927], [82.23265825261717], [81.14000782166602], [83.44260690869947], [81.31846635367762], [80.98729227761486], [83.61360969886586], [79.58125428040309], [81.08134532655455], [80.7921760391198], [83.18177373618852], [80.8075870160344], [82.09188660801564], [80.06257944656302], [80.76885454367603], [81.38875305623472], [81.67953856681983], [79.35654214746724], [83.16057109329161], [81.99413489736071], [80.44583496284709], [79.91590886868094], [80.49281314168378], [82.0217030012709], [81.48836299628398], [83.0954243253813], [82.74344935471255], [83.37733450669795], [82.93899100508409], [79.41118935837245], [79.84746259900264], [83.59726295210166], [80.77675601643513], [79.40716102523967], [81.6741638959515], [78.87323943661971], [82.81998631074606], [82.8361858190709], [82.59168704156478], [79.75736229331768], [82.34660925726588], [84.04889975550122], [83.75550122249389], [80.83357792779572], [80.00782472613459], [81.44491152605337], [82.55893573315075], [81.16749779994133], [81.79507235041063], [82.32071225907445], [81.59335288367546], [82.02620770584784], [83.71297292012905], [82.60657019945248], [80.80383336592998], [83.21439045850035], [82.01115132544263], [82.3943661971831], [81.55140369754476], [81.95150567070786], [82.9764349271536], [86.57665590451032], [82.83114850322833], [82.76941130451789], [82.67500977708252], [82.0848816741639], [82.64398161728758], [82.02972233085647], [83.45225295670022], [83.24044196734135], [80.77449638177195], [82.16660148611655], [83.14584759855228], [81.77638657928202], [83.45401174168298], [81.66177908113393], [82.60486946318568], [81.34350249339982], [81.13447432762835], [81.21455114414238], [81.13447432762835], [81.98885303608097], [80.86999022482894], [84.20228895627505], [81.02503912363068], [82.89486552567237], [81.46699266503667], [79.64593114241002], [80.88580367618303], [81.02453807801349], [82.67462336137741], [80.26791825559792], [81.06971741468662], [81.43150484012907], [80.77825576847869], [81.19131455399061], [81.21455114414238], [82.38169730152522], [84.45205479452055], [80.98219526511446], [83.09046454767726], [83.62818883784577], [82.11071987480439], [81.74083129584352], [82.83312151725485], [84.31602620514325], [83.84194053208138], [81.1479417228904], [81.0115437292115], [81.4901730712819], [82.6860999706544], [84.22854906564915], [82.77919029923724], [82.04301075268818], [82.4288647697272], [81.41082085901576], [82.92873923257635], [82.1159675369121], [82.26263811479417], [84.84255818501858], [80.53980050850772], [81.88837845762878], [83.41644666079985], [82.0803597614625], [82.43348982785602], [79.87870488115034], [81.34167807549385], [81.78173283786427], [81.78616844370536], [82.25916870415648], [81.89908077449638], [81.2457221081451], [82.82976434927154], [79.98435513835925], [83.0122249388753], [80.71016335713587], [80.24848366268832], [81.49633251833741], [83.13288354356116], [82.13552361396303], [81.88837845762878], [83.84006256721086], [80.40289458243693], [82.41908673120172], [83.12133072407045], [83.63974183453941], [80.60855102240485], [83.52895148669796], [82.24244203111242], [82.69625574347444], [81.01847326752029], [78.33610323589794], [81.47605083088955], [82.26374486401879], [84.30317848410758], [82.9764349271536], [81.89376895236232], [81.29826962557435], [80.12319123973406], [79.48366907881869], [83.80915134923738], [83.63636363636363], [82.32303480641376], [79.90028350767426], [81.5586193409602], [80.7921760391198], [81.63424885152966], [79.40946421587797], [81.50792098572268], [81.92217442315213], [83.28282334539055], [81.72127139364304], [82.26437231130231], [83.3887368009386], [83.20775026910655], [82.33167204143457], [84.53487234666927], [81.42535927265617], [82.4156479217604], [79.1234592056349], [81.69730152522487], [80.71735731039875], [80.4849432929214], [82.31957754742812], [84.7545472325445], [81.8075117370892], [84.77708251857645], [80.67448680351906], [83.29911019849419], [80.9877750611247], [83.92141530642166], [82.38341968911918], [81.43150484012907], [81.11306729264476], [81.51046761886128], [83.94481948928676], [84.26559749657734], [83.09060697878995], [82.01016816581932], [79.72417840375586], [83.08399335093381], [80.67226890756302], [83.19319515056706], [81.76838810641628], [83.55333920015646], [81.61908486507626], [79.2749658002736], [80.70038149271251], [81.00312866640594], [83.33659299823978], [83.04173590069396], [81.24144672531769], [82.58701603441533], [83.11497849041845], [82.17637856863512], [82.4841075794621], [81.25550014667058], [82.79874828867592], [82.1844138065904], [83.0841395485195], [82.22178760023469], [82.31325772389519], [79.391627543036], [80.56533646322379], [82.29136092358868], [82.70603187017304], [80.65682728961], [83.28606356968216], [79.6694699784862], [82.34431518232476], [79.79077043410247], [81.86173853524983], [81.37897310513448], [81.90355081678568], [82.46162870270798], [80.10763209393346], [81.48836299628398], [83.4767305436058], [78.03304330824128], [81.6590042062017], [80.44583496284709], [80.68837391219321], [82.98454918834344], [82.09013588816111], [83.91704167481902], [80.07823960880197], [82.76941130451789], [81.20293398533008], [81.3398533007335], [80.96635367762129], [82.8183062781146], [80.96029728143947], [81.73462403441869], [81.23534010946052], [83.8451007236456], [79.49169110459434], [81.8110698220223], [82.91943684004693], [81.9898258657797], [82.70434102463825], [82.10793899100508], [82.66653624180769], [79.5150092891366], [81.91062872787718], [81.05489773950484], [83.76845604771684], [82.06808843670514], [82.49853257679514], [81.74618693781775], [82.99266503667482], [82.13622593569822], [81.39557643374438], [80.59686888454011], [81.6741638959515], [82.225263981228], [84.26197458455523], [81.23410913358107], [83.67885781341678], [83.74889997066587], [83.24208056315994], [82.77245157503424], [81.60930778255768], [81.38193901485535], [82.17463576806493], [83.37736033656198], [82.29197223037059], [83.78801212476777], [82.71713615023474], [82.68817204301075], [81.91062872787718], [82.04752126723379], [79.86695362942673], [81.73725912158858], [81.41991003324858], [82.35236605396949], [82.01115132544263], [83.69182635901447], [81.28666405944466], [85.2170512319124], [81.66617776474038], [83.90534858707343], [81.2133072407045], [82.97498045347929], [82.48753300088002], [82.88341158059468], [83.20461433180174], [81.74354964816263], [83.52561595619868], [80.50449745795855], [78.3989834815756], [81.92570869990224], [80.11730205278592], [82.74141473437041], [80.4849432929214], [82.78255768478687], [81.16197183098592], [84.39945226917058], [82.24655391533874], [79.1377456251833], [80.66692743985918], [81.48401603284779], [79.72602739726027], [83.83186705767352], [81.93466353677621], [81.02875024447486], [80.83920187793427], [82.42370892018779], [81.27322511245843], [81.91863876393506], [80.43223156659496], [82.1498435054773], [81.10459433040079], [81.21822448181463], [80.3503278207261], [81.0403832991102], [78.8634585289515], [79.6969696969697], [79.00087985140287], [82.28219419184512], [81.01340115426], [82.2885085574572], [82.67631810623105], [81.63863903011341], [80.25620966164678], [81.68655840344356], [80.91140230784275], [81.47677261613691], [80.7959323359734], [82.26721439749609], [83.13123410913357], [82.47604146293762], [82.27130570758405], [81.41376613218615], [82.05655023970257], [79.75166210402816], [77.33229024056327], [80.3969495502542], [82.27130570758405], [81.21514528911065], [80.43414491053095], [79.41895725325246], [80.34213098729228], [80.6511536957372], [82.02796519018285], [81.44743276283619], [83.25508607198748], [84.08290965975753], [78.35565548929515], [80.90162331312342], [81.38625476586176], [79.3467631527479], [79.20211205632151], [83.05946791862286], [83.9867044676899], [81.25978090766823], [79.95499902171787], [82.51221896383186], [81.68215158924205], [82.12853369852294], [80.00195579894387], [82.38169730152522], [84.07313257723895], [81.63325183374083], [83.29257556490268], [80.39906103286386], [80.66692743985918], [82.86049696732537], [81.71948356807512], [80.95843520782397], [81.43150484012907], [81.51046761886128], [81.8252959013988], [81.6039119804401], [81.59953070003911], [81.96304624107928], [81.79595030812872], [79.12592882283927], [81.22556684910086], [81.91239734063356], [81.57457212713936], [82.33913553686682], [82.43348982785602]]
  out "max bad vectors":i32=34
  out "Bad vect index (spot)":i32[][](array[numeric])
  out "Data Array (spot,Var)":dbl[][](array[numeric])
  out "File Paths":path[](array[path])=[path "C:/Users/PIV/Documents/mike_ensight/NACA0015_MB_G/15ms_PLANE_B_PA_300/rear/ensight/ENSI.case", path "C:/Users/PIV/Documents/mike_ensight/NACA0015_MB_G/15ms_PLANE_B_PA_300/rear/ensight/ENSI.geo", path "C:/Users/PIV/Documents/mike_ensight/NACA0015_MB_G/15ms_PLANE_B_PA_300/rear/ensight/ENSI.var1", path "C:/Users/PIV/Documents/mike_ensight/NACA0015_MB_G/15ms_PLANE_B_PA_300/rear/ensight/ENSI.var2", path "C:/Users/PIV/Documents/mike_ensight/NACA0015_MB_G/15ms_PLANE_B_PA_300/rear/ensight/ENSI.var3", path "C:/Users/PIV/Documents/mike_ensight/NACA0015_MB_G/15ms_PLANE_B_PA_300/rear/ensight/ENSI.var4", path "C:/Users/PIV/Documents/mike_ensight/NACA0015_MB_G/15ms_PLANE_B_PA_300/rear/ensight/ENSI.var5", path "C:/Users/PIV/Documents/mike_ensight/NACA0015_MB_G/15ms_PLANE_B_PA_300/rear/ensight/ENSI.var6", path "C:/Users/PIV/Documents/mike_ensight/NACA0015_MB_G/15ms_PLANE_B_PA_300/rear/ensight/ENSI.var7", path "C:/Users/PIV/Documents/mike_ensight/NACA0015_MB_G/15ms_PLANE_B_PA_300/rear/ensight/ENSI.var8", path "C:/Users/PIV/Documents/mike_ensight/NACA0015_MB_G/15ms_PLANE_B_PA_300/rear/ensight/ENSI.var9", path "C:/Users/PIV/Documents/mike_ensight/NACA0015_MB_G/15ms_PLANE_B_PA_300/rear/ensight/ENSI.var10", path "C:/Users/PIV/Documents/mike_ensight/NACA0015_MB_G/15ms_PLANE_B_PA_300/rear/ensight/ENSI.var11", path "C:/Users/PIV/Documents/mike_ensight/NACA0015_MB_G/15ms_PLANE_B_PA_300/rear/ensight/ENSI.var12", path "C:/Users/PIV/Documents/mike_ensight/NACA0015_MB_G/15ms_PLANE_B_PA_300/rear/ensight/ENSI.var13", path "C:/Users/PIV/Documents/mike_ensight/NACA0015_MB_G/15ms_PLANE_B_PA_300/rear/ensight/ENSI.var14", path "C:/Users/PIV/Documents/mike_ensight/NACA0015_MB_G/15ms_PLANE_B_PA_300/rear/ensight/ENSI.var15", path "C:/Users/PIV/Documents/mike_ensight/NACA0015_MB_G/15ms_PLANE_B_PA_300/rear/ensight/ENSI.var16", path "C:/Users/PIV/Documents/mike_ensight/NACA0015_MB_G/15ms_PLANE_B_PA_300/rear/ensight/ENSI.var17", path "C:/Users/PIV/Documents/mike_ensight/NACA0015_MB_G/15ms_PLANE_B_PA_300/rear/ensight/ENSI.var18", path "C:/Users/PIV/Documents/mike_ensight/NACA0015_MB_G/15ms_PLANE_B_PA_300/rear/ensight/ENSI.var19", path "C:/Users/PIV/Documents/mike_ensight/NACA0015_MB_G/15ms_PLANE_B_PA_300/rear/ensight/ENSI.var20", path "C:/Users/PIV/Documents/mike_ensight/NACA0015_MB_G/15ms_PLANE_B_PA_300/rear/ensight/ENSI.var21", path "C:/Users/PIV/Documents/mike_ensight/NACA0015_MB_G/15ms_PLANE_B_PA_300/rear/ensight/ENSI.var22", path "C:/Users/PIV/Documents/mike_ensight/NACA0015_MB_G/15ms_PLANE_B_PA_300/rear/ensight/ENSI.var23", path "C:/Users/PIV/Documents/mike_ensight/NACA0015_MB_G/15ms_PLANE_B_PA_300/rear/ensight/ENSI.var24", path "C:/Users/PIV/Documents/mike_ensight/NACA0015_MB_G/15ms_PLANE_B_PA_300/rear/ensight/ENSI.var25", path "C:/Users/PIV/Documents/mike_ensight/NACA0015_MB_G/15ms_PLANE_B_PA_300/rear/ensight/ENSI.var26", path "C:/Users/PIV/Documents/mike_ensight/NACA0015_MB_G/15ms_PLANE_B_PA_300/rear/ensight/ENSI.var27", path "C:/Users/PIV/Documents/mike_ensight/NACA0015_MB_G/15ms_PLANE_B_PA_300/rear/ensight/ENSI.var28", path "C:/Users/PIV/Documents/mike_ensight/NACA0015_MB_G/15ms_PLANE_B_PA_300/rear/ensight/ENSI.var29", path "C:/Users/PIV/Documents/mike_ensight/NACA0015_MB_G/15ms_PLANE_B_PA_300/rear/ensight/ENSI.var30", path "C:/Users/PIV/Documents/mike_ensight/NACA0015_MB_G/15ms_PLANE_B_PA_300/rear/ensight/ENSI.var31", path "C:/Users/PIV/Documents/mike_ensight/NACA0015_MB_G/15ms_PLANE_B_PA_300/rear/ensight/ENSI.var32", path "C:/Users/PIV/Documents/mike_ensight/NACA0015_MB_G/15ms_PLANE_B_PA_300/rear/ensight/ENSI.var33", path "C:/Users/PIV/Documents/mike_ensight/NACA0015_MB_G/15ms_PLANE_B_PA_300/rear/ensight/ENSI.var34", path "C:/Users/PIV/Documents/mike_ensight/NACA0015_MB_G/15ms_PLANE_B_PA_300/rear/ensight/ENSI.var35", path "C:/Users/PIV/Documents/mike_ensight/NACA0015_MB_G/15ms_PLANE_B_PA_300/rear/ensight/ENSI.var36", path "C:/Users/PIV/Documents/mike_ensight/NACA0015_MB_G/15ms_PLANE_B_PA_300/rear/ensight/ENSI.var37", path "C:/Users/PIV/Documents/mike_ensight/NACA0015_MB_G/15ms_PLANE_B_PA_300/rear/ensight/ENSI.var38", path "C:/Users/PIV/Documents/mike_ensight/NACA0015_MB_G/15ms_PLANE_B_PA_300/rear/ensight/ENSI.var39", path "C:/Users/PIV/Documents/mike_ensight/NACA0015_MB_G/15ms_PLANE_B_PA_300/rear/ensight/ENSI.var40", path "C:/Users/PIV/Documents/mike_ensight/NACA0015_MB_G/15ms_PLANE_B_PA_300/rear/ensight/ENSI.var41", path "C:/Users/PIV/Documents/mike_ensight/NACA0015_MB_G/15ms_PLANE_B_PA_300/rear/ensight/ENSI.var42", path "C:/Users/PIV/Documents/mike_ensight/NACA0015_MB_G/15ms_PLANE_B_PA_300/rear/ensight/ENSI.var43", path "C:/Users/PIV/Documents/mike_ensight/NACA0015_MB_G/15ms_PLANE_B_PA_300/rear/ensight/ENSI.var44", path "C:/Users/PIV/Documents/mike_ensight/NACA0015_MB_G/15ms_PLANE_B_PA_300/rear/ensight/ENSI.var45"]
  out "Position Array (XYZ,spot)":dbl[][](array[numeric])
  out "Variable Names":string[](array[string])=["Record_Length", "Turb_Stats_U_ms", "Turb_Stats_u2_m2s2", "Turb_Stats_u3_m3s3", "Turb_Stats_u4_m4s4", "Turb_Stats_TurbU_%", "Turb_Stats_Skew_u", "Turb_Stats_Kurt_u", "Turb_Stats_V_ms", "Turb_Stats_v2_m2s2", "Turb_Stats_v3_m3s3", "Turb_Stats_v4_m4s4", "Turb_Stats_TurbV_%", "Turb_Stats_Skew_v", "Turb_Stats_Kurt_v", "Turb_Stats_u2v2_m4s4", "Turb_Stats_uv3_m4s4", "Turb_Stats_u3v_m4s4", "Turb_Stats_uv2_m3s3", "Turb_Stats_u2v_m3s3", "Turb_Stats_uv_cc", "Turb_Stats_uv", "Turb_Stats_TKE_J", "Turb_Stats_Error_U_ms", "Turb_Stats_Error_u2_m2s2", "Turb_Stats_Error_u3_m3s3", "Turb_Stats_Error_u4_m4s4", "Turb_Stats_Error_TurbU_%", "Turb_Stats_Error_Skew_u", "Turb_Stats_Error_Kurt_u", "Turb_Stats_Error_V_ms", "Turb_Stats_Error_v2_m2s2", "Turb_Stats_Error_v3_m3s3", "Turb_Stats_Error_v4_m4s4", "Turb_Stats_Error_TurbV_%", "Turb_Stats_Error_Skew_v", "Turb_Stats_Error_Kurt_v", "Turb_Stats_Error_u2v2_m4s4", "Turb_Stats_Error_uv3_m4s4", "Turb_Stats_Error_u3v_m4s4", "Turb_Stats_Error_uv2_m3s3", "Turb_Stats_Error_u2v_m3s3", "Turb_Stats_Error_uv_cc", "Turb_Stats_Error_uv", "Turb_Stats_Error_TKE_J"]
  out "time s":dbl[](array[numeric])=[0.0, 0.13806910358634494, 0.2761382071726899, 0.41420731075903483, 0.5522764143453798, 0.6903455179317247, 0.8284146215180697, 0.9664837251044146, 1.1045528286907595, 1.2426219322771046, 1.3806910358634494, 1.5187601394497943, 1.6568292430361393, 1.7948983466224844, 1.9329674502088292, 2.071036553795174, 2.209105657381519, 2.347174760967864, 2.485243864554209, 2.623312968140554, 2.761382071726899, 2.899451175313244, 3.0375202788995885, 3.1755893824859336, 3.3136584860722786, 3.4517275896586237, 3.5897966932449688, 3.7278657968313134, 3.8659349004176584, 4.0040040040040035, 4.142073107590348, 4.280142211176694, 4.418211314763038, 4.556280418349383, 4.694349521935728, 4.832418625522073, 4.970487729108418, 5.108556832694763, 5.246625936281108, 5.384695039867453, 5.522764143453798, 5.660833247040142, 5.798902350626488, 5.9369714542128325, 6.075040557799177, 6.213109661385523, 6.351178764971867, 6.489247868558213, 6.627316972144557, 6.765386075730902, 6.903455179317247, 7.041524282903592, 7.1795933864899375, 7.317662490076282, 7.455731593662627, 7.593800697248972, 7.731869800835317, 7.869938904421661, 8.008008008008007, 8.146077111594352, 8.284146215180696, 8.42221531876704, 8.560284422353387, 8.698353525939732, 8.836422629526076, 8.974491733112421, 9.112560836698766, 9.250629940285112, 9.388699043871457, 9.526768147457801, 9.664837251044146, 9.80290635463049, 9.940975458216837, 10.079044561803181, 10.217113665389526, 10.35518276897587, 10.493251872562215, 10.63132097614856, 10.769390079734906, 10.90745918332125, 11.045528286907595, 11.18359739049394, 11.321666494080285, 11.459735597666631, 11.597804701252976, 11.73587380483932, 11.873942908425665, 12.01201201201201, 12.150081115598354, 12.2881502191847, 12.426219322771045, 12.56428842635739, 12.702357529943734, 12.840426633530079, 12.978495737116425, 13.11656484070277, 13.254633944289115, 13.39270304787546, 13.530772151461804, 13.66884125504815, 13.806910358634495, 13.94497946222084, 14.083048565807184, 14.221117669393529, 14.359186772979875, 14.49725587656622, 14.635324980152564, 14.773394083738909, 14.911463187325253, 15.049532290911598, 15.187601394497944, 15.325670498084289, 15.463739601670634, 15.601808705256978, 15.739877808843323, 15.87794691242967, 16.016016016016014, 16.154085119602357, 16.292154223188703, 16.43022332677505, 16.568292430361392, 16.70636153394774, 16.84443063753408, 16.982499741120428, 17.120568844706774, 17.258637948293117, 17.396707051879464, 17.534776155465806, 17.672845259052153, 17.8109143626385, 17.948983466224842, 18.08705256981119, 18.22512167339753, 18.363190776983878, 18.501259880570224, 18.639328984156567, 18.777398087742913, 18.915467191329256, 19.053536294915602, 19.19160539850195, 19.32967450208829, 19.467743605674638, 19.60581270926098, 19.743881812847327, 19.881950916433674, 20.020020020020016, 20.158089123606363, 20.296158227192706, 20.434227330779052, 20.572296434365395, 20.71036553795174, 20.848434641538088, 20.98650374512443, 21.124572848710777, 21.26264195229712, 21.400711055883466, 21.538780159469813, 21.676849263056155, 21.8149183666425, 21.952987470228845, 22.09105657381519, 22.229125677401537, 22.36719478098788, 22.505263884574227, 22.64333298816057, 22.781402091746916, 22.919471195333262, 23.057540298919605, 23.19560940250595, 23.333678506092294, 23.47174760967864, 23.609816713264987, 23.74788581685133, 23.885954920437676, 24.02402402402402, 24.162093127610365, 24.30016223119671, 24.438231334783055, 24.5763004383694, 24.714369541955744, 24.85243864554209, 24.990507749128433, 25.12857685271478, 25.266645956301126, 25.40471505988747, 25.542784163473815, 25.680853267060158, 25.818922370646504, 25.95699147423285, 26.095060577819194, 26.23312968140554, 26.371198784991883, 26.50926788857823, 26.647336992164576, 26.78540609575092, 26.923475199337265, 27.061544302923608, 27.199613406509954, 27.3376825100963, 27.475751613682643, 27.61382071726899, 27.751889820855332, 27.88995892444168, 28.028028028028025, 28.166097131614368, 28.304166235200714, 28.442235338787057, 28.580304442373404, 28.71837354595975, 28.856442649546093, 28.99451175313244, 29.132580856718782, 29.27064996030513, 29.40871906389147, 29.546788167477818, 29.684857271064164, 29.822926374650507, 29.960995478236853, 30.099064581823196, 30.237133685409542, 30.37520278899589, 30.51327189258223, 30.651340996168578, 30.78941009975492, 30.927479203341267, 31.065548306927614, 31.203617410513957, 31.341686514100303, 31.479755617686646, 31.617824721272992, 31.75589382485934, 31.89396292844568, 32.03203203203203, 32.170101135618374, 32.30817023920471, 32.44623934279106, 32.584308446377406, 32.72237754996375, 32.8604466535501, 32.99851575713644, 33.136584860722785, 33.27465396430913, 33.41272306789548, 33.550792171481824, 33.68886127506816, 33.82693037865451, 33.964999482240856, 34.1030685858272, 34.24113768941355, 34.37920679299989, 34.517275896586234, 34.65534500017258, 34.79341410375893, 34.93148320734527, 35.06955231093161, 35.20762141451796, 35.345690518104306, 35.48375962169065, 35.621828725277, 35.75989782886334, 35.897966932449684, 36.03603603603603, 36.17410513962238, 36.31217424320872, 36.45024334679506, 36.58831245038141, 36.726381553967755, 36.8644506575541, 37.00251976114045, 37.14058886472679, 37.278657968313134, 37.41672707189948, 37.554796175485826, 37.69286527907217, 37.83093438265851, 37.96900348624486, 38.107072589831205, 38.24514169341755, 38.3832107970039, 38.52127990059024, 38.65934900417658, 38.79741810776293, 38.935487211349276, 39.07355631493562, 39.21162541852196, 39.34969452210831, 39.487763625694654, 39.625832729281, 39.76390183286735, 39.90197093645369, 40.04004004004003, 40.17810914362638, 40.316178247212726, 40.454247350799065, 40.59231645438541, 40.73038555797176, 40.868454661558104, 41.00652376514445, 41.14459286873079, 41.282661972317136, 41.42073107590348, 41.55880017948983, 41.696869283076175, 41.834938386662515, 41.97300749024886, 42.11107659383521, 42.249145697421554, 42.3872148010079, 42.52528390459424, 42.663353008180586, 42.80142211176693, 42.93949121535328, 43.077560318939625, 43.215629422525964, 43.35369852611231, 43.49176762969866, 43.629836733285, 43.76790583687135, 43.90597494045769, 44.044044044044036, 44.18211314763038, 44.32018225121673, 44.458251354803075, 44.596320458389414, 44.73438956197576, 44.87245866556211, 45.01052776914845, 45.1485968727348, 45.28666597632114, 45.424735079907485, 45.56280418349383, 45.70087328708018, 45.838942390666524, 45.977011494252864, 46.11508059783921, 46.253149701425556, 46.3912188050119, 46.52928790859825, 46.66735701218459, 46.805426115770935, 46.94349521935728, 47.08156432294363, 47.219633426529974, 47.35770253011631, 47.49577163370266, 47.633840737289006, 47.77190984087535, 47.9099789444617, 48.04804804804804, 48.186117151634384, 48.32418625522073, 48.46225535880708, 48.60032446239342, 48.73839356597976, 48.87646266956611, 49.014531773152456, 49.1526008767388, 49.29066998032514, 49.42873908391149, 49.566808187497834, 49.70487729108418, 49.84294639467053, 49.981015498256866, 50.11908460184321, 50.25715370542956, 50.395222809015905, 50.53329191260225, 50.67136101618859, 50.80943011977494, 50.947499223361284, 51.08556832694763, 51.22363743053398, 51.361706534120316, 51.49977563770666, 51.63784474129301, 51.775913844879355, 51.9139829484657, 52.05205205205204, 52.19012115563839, 52.32819025922473, 52.46625936281108, 52.604328466397426, 52.742397569983765, 52.88046667357011, 53.01853577715646, 53.156604880742805, 53.29467398432915, 53.43274308791549, 53.57081219150184, 53.70888129508818, 53.84695039867453, 53.985019502260876, 54.123088605847215, 54.26115770943356, 54.39922681301991, 54.537295916606254, 54.6753650201926, 54.81343412377894, 54.951503227365286, 55.08957233095163, 55.22764143453798, 55.365710538124326, 55.503779641710665, 55.64184874529701, 55.77991784888336, 55.917986952469704, 56.05605605605605, 56.19412515964239, 56.332194263228736, 56.47026336681508, 56.60833247040143, 56.746401573987775, 56.884470677574114, 57.02253978116046, 57.16060888474681, 57.298677988333154, 57.4367470919195, 57.57481619550584, 57.712885299092186, 57.85095440267853, 57.98902350626488, 58.12709260985122, 58.265161713437564, 58.40323081702391, 58.54129992061026, 58.6793690241966, 58.81743812778294, 58.95550723136929, 59.093576334955635, 59.23164543854198, 59.36971454212833, 59.50778364571467, 59.645852749301014, 59.78392185288736, 59.92199095647371, 60.06006006006005, 60.19812916364639, 60.33619826723274, 60.474267370819085, 60.61233647440543, 60.75040557799178, 60.88847468157812, 61.02654378516446, 61.16461288875081, 61.302681992337156, 61.4407510959235, 61.57882019950984, 61.71688930309619, 61.854958406682535, 61.99302751026888, 62.13109661385523, 62.26916571744157, 62.40723482102791, 62.54530392461426, 62.683373028200606, 62.82144213178695, 62.95951123537329, 63.09758033895964, 63.235649442545984, 63.37371854613233, 63.51178764971868, 63.649856753305016, 63.78792585689136, 63.92599496047771, 64.06406406406406, 64.2021331676504, 64.34020227123675, 64.4782713748231, 64.61634047840943, 64.75440958199577, 64.89247868558212, 65.03054778916847, 65.16861689275481, 65.30668599634116, 65.4447550999275, 65.58282420351385, 65.7208933071002, 65.85896241068654, 65.99703151427288, 66.13510061785922, 66.27316972144557, 66.41123882503192, 66.54930792861826, 66.68737703220461, 66.82544613579095, 66.9635152393773, 67.10158434296365, 67.23965344655, 67.37772255013633, 67.51579165372267, 67.65386075730902, 67.79192986089537, 67.92999896448171, 68.06806806806806, 68.2061371716544, 68.34420627524075, 68.4822753788271, 68.62034448241344, 68.75841358599978, 68.89648268958612, 69.03455179317247, 69.17262089675881, 69.31069000034516, 69.44875910393151, 69.58682820751785, 69.7248973111042, 69.86296641469055, 70.0010355182769, 70.13910462186323, 70.27717372544957, 70.41524282903592, 70.55331193262226, 70.69138103620861, 70.82945013979496, 70.9675192433813, 71.10558834696765, 71.243657450554, 71.38172655414033, 71.51979565772668, 71.65786476131302, 71.79593386489937, 71.93400296848571, 72.07207207207206, 72.2101411756584, 72.34821027924475, 72.4862793828311, 72.62434848641745, 72.76241759000378, 72.90048669359012, 73.03855579717647, 73.17662490076282, 73.31469400434916, 73.45276310793551, 73.59083221152186, 73.7289013151082, 73.86697041869455, 74.0050395222809, 74.14310862586723, 74.28117772945357, 74.41924683303992, 74.55731593662627, 74.69538504021261, 74.83345414379896, 74.9715232473853, 75.10959235097165, 75.247661454558, 75.38573055814435, 75.52379966173068, 75.66186876531702, 75.79993786890337, 75.93800697248972, 76.07607607607606, 76.21414517966241, 76.35221428324876, 76.4902833868351, 76.62835249042145, 76.7664215940078, 76.90449069759413, 77.04255980118047, 77.18062890476682, 77.31869800835317, 77.45676711193951, 77.59483621552586, 77.7329053191122, 77.87097442269855, 78.0090435262849, 78.14711262987124, 78.28518173345758, 78.42325083704392, 78.56131994063027, 78.69938904421662, 78.83745814780296, 78.97552725138931, 79.11359635497566, 79.251665458562, 79.38973456214835, 79.5278036657347, 79.66587276932103, 79.80394187290737, 79.94201097649372, 80.08008008008007, 80.21814918366641, 80.35621828725276, 80.4942873908391, 80.63235649442545, 80.7704255980118, 80.90849470159813, 81.04656380518448, 81.18463290877082, 81.32270201235717, 81.46077111594352, 81.59884021952986, 81.73690932311621, 81.87497842670255, 82.0130475302889, 82.15111663387525, 82.28918573746158, 82.42725484104793, 82.56532394463427, 82.70339304822062, 82.84146215180697, 82.97953125539331, 83.11760035897966, 83.255669462566, 83.39373856615235, 83.5318076697387, 83.66987677332503, 83.80794587691138, 83.94601498049772, 84.08408408408407, 84.22215318767041, 84.36022229125676, 84.49829139484311, 84.63636049842945, 84.7744296020158, 84.91249870560215, 85.05056780918848, 85.18863691277483, 85.32670601636117, 85.46477511994752, 85.60284422353386, 85.74091332712021, 85.87898243070656, 86.0170515342929, 86.15512063787925, 86.2931897414656, 86.43125884505193, 86.56932794863827, 86.70739705222462, 86.84546615581097, 86.98353525939731, 87.12160436298366, 87.25967346657, 87.39774257015635, 87.5358116737427, 87.67388077732905, 87.81194988091538, 87.95001898450172, 88.08808808808807, 88.22615719167442, 88.36422629526076, 88.50229539884711, 88.64036450243346, 88.7784336060198, 88.91650270960615, 89.05457181319248, 89.19264091677883, 89.33071002036517, 89.46877912395152, 89.60684822753787, 89.74491733112421, 89.88298643471056, 90.0210555382969, 90.15912464188325, 90.2971937454696, 90.43526284905593, 90.57333195264228, 90.71140105622862, 90.84947015981497, 90.98753926340132, 91.12560836698766, 91.26367747057401, 91.40174657416036, 91.5398156777467, 91.67788478133305, 91.81595388491938, 91.95402298850573, 92.09209209209207, 92.23016119567842, 92.36823029926477, 92.50629940285111, 92.64436850643746, 92.7824376100238, 92.92050671361015, 93.0585758171965, 93.19664492078283, 93.33471402436918, 93.47278312795552, 93.61085223154187, 93.74892133512822, 93.88699043871456, 94.02505954230091, 94.16312864588726, 94.3011977494736, 94.43926685305995, 94.57733595664628, 94.71540506023263, 94.85347416381897, 94.99154326740532, 95.12961237099167, 95.26768147457801, 95.40575057816436, 95.5438196817507, 95.68188878533705, 95.8199578889234, 95.95802699250973, 96.09609609609608, 96.23416519968242, 96.37223430326877, 96.51030340685512, 96.64837251044146, 96.78644161402781, 96.92451071761415, 97.0625798212005, 97.20064892478683, 97.33871802837318, 97.47678713195953, 97.61485623554587, 97.75292533913222, 97.89099444271856, 98.02906354630491, 98.16713264989126, 98.3052017534776, 98.44327085706395, 98.58133996065028, 98.71940906423663, 98.85747816782298, 98.99554727140932, 99.13361637499567, 99.27168547858201, 99.40975458216836, 99.54782368575471, 99.68589278934105, 99.8239618929274, 99.96203099651373, 100.10010010010008, 100.23816920368643, 100.37623830727277, 100.51430741085912, 100.65237651444546, 100.79044561803181, 100.92851472161816, 101.0665838252045, 101.20465292879085, 101.34272203237718, 101.48079113596353, 101.61886023954987, 101.75692934313622, 101.89499844672257, 102.03306755030891, 102.17113665389526, 102.3092057574816, 102.44727486106795, 102.5853439646543, 102.72341306824063, 102.86148217182698, 102.99955127541332, 103.13762037899967, 103.27568948258602, 103.41375858617236, 103.55182768975871, 103.68989679334506, 103.8279658969314, 103.96603500051775, 104.10410410410408, 104.24217320769043, 104.38024231127677, 104.51831141486312, 104.65638051844947, 104.79444962203581, 104.93251872562216, 105.0705878292085, 105.20865693279485, 105.3467260363812, 105.48479513996753, 105.62286424355388, 105.76093334714022, 105.89900245072657, 106.03707155431292, 106.17514065789926, 106.31320976148561, 106.45127886507196, 106.5893479686583, 106.72741707224463, 106.86548617583098, 107.00355527941733, 107.14162438300367, 107.27969348659002, 107.41776259017637, 107.55583169376271, 107.69390079734906, 107.8319699009354, 107.97003900452175, 108.10810810810808, 108.24617721169443, 108.38424631528078, 108.52231541886712, 108.66038452245347, 108.79845362603982, 108.93652272962616, 109.07459183321251, 109.21266093679886, 109.3507300403852, 109.48879914397153, 109.62686824755788, 109.76493735114423, 109.90300645473057, 110.04107555831692, 110.17914466190327, 110.31721376548961, 110.45528286907596, 110.5933519726623, 110.73142107624865, 110.86949017983498, 111.00755928342133, 111.14562838700768, 111.28369749059402, 111.42176659418037, 111.55983569776672, 111.69790480135306, 111.83597390493941, 111.97404300852575, 112.1121121121121, 112.25018121569843, 112.38825031928478, 112.52631942287113, 112.66438852645747, 112.80245763004382, 112.94052673363016, 113.07859583721651, 113.21666494080286, 113.3547340443892, 113.49280314797555, 113.63087225156188, 113.76894135514823, 113.90701045873458, 114.04507956232092, 114.18314866590727, 114.32121776949361, 114.45928687307996, 114.59735597666631, 114.73542508025265, 114.873494183839, 115.01156328742533, 115.14963239101168, 115.28770149459802, 115.42577059818437, 115.56383970177072, 115.70190880535706, 115.83997790894341, 115.97804701252976, 116.1161161161161, 116.25418521970244, 116.39225432328878, 116.53032342687513, 116.66839253046147, 116.80646163404782, 116.94453073763417, 117.08259984122051, 117.22066894480686, 117.3587380483932, 117.49680715197955, 117.63487625556589, 117.77294535915223, 117.91101446273858, 118.04908356632492, 118.18715266991127, 118.32522177349762, 118.46329087708396, 118.60135998067031, 118.73942908425666, 118.877498187843, 119.01556729142933, 119.15363639501568, 119.29170549860203, 119.42977460218837, 119.56784370577472, 119.70591280936107, 119.84398191294741, 119.98205101653376, 120.1201201201201, 120.25818922370645, 120.39625832729278, 120.53432743087913, 120.67239653446548, 120.81046563805182, 120.94853474163817, 121.08660384522452, 121.22467294881086, 121.36274205239721, 121.50081115598356, 121.6388802595699, 121.77694936315623, 121.91501846674258, 122.05308757032893, 122.19115667391527, 122.32922577750162, 122.46729488108797, 122.60536398467431, 122.74343308826066, 122.881502191847, 123.01957129543335, 123.15764039901968, 123.29570950260603, 123.43377860619238, 123.57184770977872, 123.70991681336507, 123.84798591695142, 123.98605502053776, 124.12412412412411, 124.26219322771045, 124.40026233129679, 124.53833143488313, 124.67640053846948, 124.81446964205583, 124.95253874564217, 125.09060784922852, 125.22867695281487, 125.36674605640121, 125.50481515998756, 125.6428842635739, 125.78095336716024, 125.91902247074658, 126.05709157433293, 126.19516067791928, 126.33322978150562, 126.47129888509197, 126.60936798867831, 126.74743709226466, 126.88550619585101, 127.02357529943735, 127.16164440302369, 127.29971350661003, 127.43778261019638, 127.57585171378273, 127.71392081736907, 127.85198992095542, 127.99005902454176, 128.1281281281281, 128.26619723171444, 128.4042663353008, 128.54233543888714, 128.6804045424735, 128.81847364605983, 128.9565427496462, 129.09461185323252, 129.23268095681885, 129.37075006040521, 129.50881916399155, 129.6468882675779, 129.78495737116424, 129.9230264747506, 130.06109557833693, 130.1991646819233, 130.33723378550962, 130.47530288909599, 130.61337199268232, 130.75144109626865, 130.889510199855, 131.02757930344134, 131.1656484070277, 131.30371751061404, 131.4417866142004, 131.57985571778673, 131.7179248213731, 131.85599392495942, 131.99406302854575, 132.1321321321321, 132.27020123571845, 132.4082703393048, 132.54633944289114, 132.6844085464775, 132.82247765006383, 132.9605467536502, 133.09861585723652, 133.23668496082286, 133.37475406440922, 133.51282316799555, 133.6508922715819, 133.78896137516824, 133.9270304787546, 134.06509958234093, 134.2031686859273, 134.34123778951363, 134.4793068931, 134.61737599668632, 134.75544510027265, 134.893514203859, 135.03158330744535, 135.1696524110317, 135.30772151461804, 135.4457906182044, 135.58385972179073, 135.7219288253771, 135.85999792896342, 135.99806703254976, 136.13613613613612, 136.27420523972245, 136.4122743433088, 136.55034344689514, 136.6884125504815, 136.82648165406783, 136.9645507576542, 137.10261986124053, 137.2406889648269, 137.37875806841322, 137.51682717199955, 137.6548962755859, 137.79296537917224, 137.9310344827586]
  out "File Array":path[](array[path])=[path "C:/Users/PIV/Documents/mike_ensight/NACA0015_MB_G/15ms_PLANE_B_PA_300/rear/15ms_PLANE_B_PA_300_000000.T000.D000.P007.H000.L.vec", path "C:/Users/PIV/Documents/mike_ensight/NACA0015_MB_G/15ms_PLANE_B_PA_300/rear/15ms_PLANE_B_PA_300_000001.T000.D000.P007.H000.L.vec", path "C:/Users/PIV/Documents/mike_ensight/NACA0015_MB_G/15ms_PLANE_B_PA_300/rear/15ms_PLANE_B_PA_300_000002.T000.D000.P007.H000.L.vec", path "C:/Users/PIV/Documents/mike_ensight/NACA0015_MB_G/15ms_PLANE_B_PA_300/rear/15ms_PLANE_B_PA_300_000003.T000.D000.P007.H000.L.vec", path "C:/Users/PIV/Documents/mike_ensight/NACA0015_MB_G/15ms_PLANE_B_PA_300/rear/15ms_PLANE_B_PA_300_000004.T000.D000.P007.H000.L.vec", path "C:/Users/PIV/Documents/mike_ensight/NACA0015_MB_G/15ms_PLANE_B_PA_300/rear/15ms_PLANE_B_PA_300_000005.T000.D000.P007.H000.L.vec", path "C:/Users/PIV/Documents/mike_ensight/NACA0015_MB_G/15ms_PLANE_B_PA_300/rear/15ms_PLANE_B_PA_300_000006.T000.D000.P007.H000.L.vec", path "C:/Users/PIV/Documents/mike_ensight/NACA0015_MB_G/15ms_PLANE_B_PA_300/rear/15ms_PLANE_B_PA_300_000007.T000.D000.P007.H000.L.vec", path "C:/Users/PIV/Documents/mike_ensight/NACA0015_MB_G/15ms_PLANE_B_PA_300/rear/15ms_PLANE_B_PA_300_000008.T000.D000.P007.H000.L.vec", path "C:/Users/PIV/Documents/mike_ensight/NACA0015_MB_G/15ms_PLANE_B_PA_300/rear/15ms_PLANE_B_PA_300_000009.T000.D000.P007.H000.L.vec", path "C:/Users/PIV/Documents/mike_ensight/NACA0015_MB_G/15ms_PLANE_B_PA_300/rear/15ms_PLANE_B_PA_300_000010.T000.D000.P007.H000.L.vec", path "C:/Users/PIV/Documents/mike_ensight/NACA0015_MB_G/15ms_PLANE_B_PA_300/rear/15ms_PLANE_B_PA_300_000011.T000.D000.P007.H000.L.vec", path "C:/Users/PIV/Documents/mike_ensight/NACA0015_MB_G/15ms_PLANE_B_PA_300/rear/15ms_PLANE_B_PA_300_000012.T000.D000.P007.H000.L.vec", path "C:/Users/PIV/Documents/mike_ensight/NACA0015_MB_G/15ms_PLANE_B_PA_300/rear/15ms_PLANE_B_PA_300_000013.T000.D000.P007.H000.L.vec", path "C:/Users/PIV/Documents/mike_ensight/NACA0015_MB_G/15ms_PLANE_B_PA_300/rear/15ms_PLANE_B_PA_300_000014.T000.D000.P007.H000.L.vec", path "C:/Users/PIV/Documents/mike_ensight/NACA0015_MB_G/15ms_PLANE_B_PA_300/rear/15ms_PLANE_B_PA_300_000015.T000.D000.P007.H000.L.vec", path "C:/Users/PIV/Documents/mike_ensight/NACA0015_MB_G/15ms_PLANE_B_PA_300/rear/15ms_PLANE_B_PA_300_000016.T000.D000.P007.H000.L.vec", path "C:/Users/PIV/Documents/mike_ensight/NACA0015_MB_G/15ms_PLANE_B_PA_300/rear/15ms_PLANE_B_PA_300_000017.T000.D000.P007.H000.L.vec", path "C:/Users/PIV/Documents/mike_ensight/NACA0015_MB_G/15ms_PLANE_B_PA_300/rear/15ms_PLANE_B_PA_300_000018.T000.D000.P007.H000.L.vec", path "C:/Users/PIV/Documents/mike_ensight/NACA0015_MB_G/15ms_PLANE_B_PA_300/rear/15ms_PLANE_B_PA_300_000019.T000.D000.P007.H000.L.vec", path "C:/Users/PIV/Documents/mike_ensight/NACA0015_MB_G/15ms_PLANE_B_PA_300/rear/15ms_PLANE_B_PA_300_000020.T000.D000.P007.H000.L.vec", path "C:/Users/PIV/Documents/mike_ensight/NACA0015_MB_G/15ms_PLANE_B_PA_300/rear/15ms_PLANE_B_PA_300_000021.T000.D000.P007.H000.L.vec", path "C:/Users/PIV/Documents/mike_ensight/NACA0015_MB_G/15ms_PLANE_B_PA_300/rear/15ms_PLANE_B_PA_300_000022.T000.D000.P007.H000.L.vec", path "C:/Users/PIV/Documents/mike_ensight/NACA0015_MB_G/15ms_PLANE_B_PA_300/rear/15ms_PLANE_B_PA_300_000023.T000.D000.P007.H000.L.vec", path "C:/Users/PIV/Documents/mike_ensight/NACA0015_MB_G/15ms_PLANE_B_PA_300/rear/15ms_PLANE_B_PA_300_000024.T000.D000.P007.H000.L.vec", path "C:/Users/PIV/Documents/mike_ensight/NACA0015_MB_G/15ms_PLANE_B_PA_300/rear/15ms_PLANE_B_PA_300_000025.T000.D000.P007.H000.L.vec", path "C:/Users/PIV/Documents/mike_ensight/NACA0015_MB_G/15ms_PLANE_B_PA_300/rear/15ms_PLANE_B_PA_300_000026.T000.D000.P007.H000.L.vec", path "C:/Users/PIV/Documents/mike_ensight/NACA0015_MB_G/15ms_PLANE_B_PA_300/rear/15ms_PLANE_B_PA_300_000027.T000.D000.P007.H000.L.vec", path "C:/Users/PIV/Documents/mike_ensight/NACA0015_MB_G/15ms_PLANE_B_PA_300/rear/15ms_PLANE_B_PA_300_000028.T000.D000.P007.H000.L.vec", path "C:/Users/PIV/Documents/mike_ensight/NACA0015_MB_G/15ms_PLANE_B_PA_300/rear/15ms_PLANE_B_PA_300_000029.T000.D000.P007.H000.L.vec", path "C:/Users/PIV/Documents/mike_ensight/NACA0015_MB_G/15ms_PLANE_B_PA_300/rear/15ms_PLANE_B_PA_300_000030.T000.D000.P007.H000.L.vec", path "C:/Users/PIV/Documents/mike_ensight/NACA0015_MB_G/15ms_PLANE_B_PA_300/rear/15ms_PLANE_B_PA_300_000031.T000.D000.P007.H000.L.vec", path "C:/Users/PIV/Documents/mike_ensight/NACA0015_MB_G/15ms_PLANE_B_PA_300/rear/15ms_PLANE_B_PA_300_000032.T000.D000.P007.H000.L.vec", path "C:/Users/PIV/Documents/mike_ensight/NACA0015_MB_G/15ms_PLANE_B_PA_300/rear/15ms_PLANE_B_PA_300_000033.T000.D000.P007.H000.L.vec", path "C:/Users/PIV/Documents/mike_ensight/NACA0015_MB_G/15ms_PLANE_B_PA_300/rear/15ms_PLANE_B_PA_300_000034.T000.D000.P007.H000.L.vec", path "C:/Users/PIV/Documents/mike_ensight/NACA0015_MB_G/15ms_PLANE_B_PA_300/rear/15ms_PLANE_B_PA_300_000035.T000.D000.P007.H000.L.vec", path "C:/Users/PIV/Documents/mike_ensight/NACA0015_MB_G/15ms_PLANE_B_PA_300/rear/15ms_PLANE_B_PA_300_000036.T000.D000.P007.H000.L.vec", path "C:/Users/PIV/Documents/mike_ensight/NACA0015_MB_G/15ms_PLANE_B_PA_300/rear/15ms_PLANE_B_PA_300_000037.T000.D000.P007.H000.L.vec", path "C:/Users/PIV/Documents/mike_ensight/NACA0015_MB_G/15ms_PLANE_B_PA_300/rear/15ms_PLANE_B_PA_300_000038.T000.D000.P007.H000.L.vec", path "C:/Users/PIV/Documents/mike_ensight/NACA0015_MB_G/15ms_PLANE_B_PA_300/rear/15ms_PLANE_B_PA_300_000039.T000.D000.P007.H000.L.vec", path "C:/Users/PIV/Documents/mike_ensight/NACA0015_MB_G/15ms_PLANE_B_PA_300/rear/15ms_PLANE_B_PA_300_000040.T000.D000.P007.H000.L.vec", path "C:/Users/PIV/Documents/mike_ensight/NACA0015_MB_G/15ms_PLANE_B_PA_300/rear/15ms_PLANE_B_PA_300_000041.T000.D000.P007.H000.L.vec", path "C:/Users/PIV/Documents/mike_ensight/NACA0015_MB_G/15ms_PLANE_B_PA_300/rear/15ms_PLANE_B_PA_300_000042.T000.D000.P007.H000.L.vec", path "C:/Users/PIV/Documents/mike_ensight/NACA0015_MB_G/15ms_PLANE_B_PA_300/rear/15ms_PLANE_B_PA_300_000043.T000.D000.P007.H000.L.vec", path "C:/Users/PIV/Documents/mike_ensight/NACA0015_MB_G/15ms_PLANE_B_PA_300/rear/15ms_PLANE_B_PA_300_000044.T000.D000.P007.H000.L.vec", path "C:/Users/PIV/Documents/mike_ensight/NACA0015_MB_G/15ms_PLANE_B_PA_300/rear/15ms_PLANE_B_PA_300_000045.T000.D000.P007.H000.L.vec", path "C:/Users/PIV/Documents/mike_ensight/NACA0015_MB_G/15ms_PLANE_B_PA_300/rear/15ms_PLANE_B_PA_300_000046.T000.D000.P007.H000.L.vec", path "C:/Users/PIV/Documents/mike_ensight/NACA0015_MB_G/15ms_PLANE_B_PA_300/rear/15ms_PLANE_B_PA_300_000047.T000.D000.P007.H000.L.vec", path "C:/Users/PIV/Documents/mike_ensight/NACA0015_MB_G/15ms_PLANE_B_PA_300/rear/15ms_PLANE_B_PA_300_000048.T000.D000.P007.H000.L.vec", path "C:/Users/PIV/Documents/mike_ensight/NACA0015_MB_G/15ms_PLANE_B_PA_300/rear/15ms_PLANE_B_PA_300_000049.T000.D000.P007.H000.L.vec", path "C:/Users/PIV/Documents/mike_ensight/NACA0015_MB_G/15ms_PLANE_B_PA_300/rear/15ms_PLANE_B_PA_300_000050.T000.D000.P007.H000.L.vec", path "C:/Users/PIV/Documents/mike_ensight/NACA0015_MB_G/15ms_PLANE_B_PA_300/rear/15ms_PLANE_B_PA_300_000051.T000.D000.P007.H000.L.vec", path "C:/Users/PIV/Documents/mike_ensight/NACA0015_MB_G/15ms_PLANE_B_PA_300/rear/15ms_PLANE_B_PA_300_000052.T000.D000.P007.H000.L.vec", path "C:/Users/PIV/Documents/mike_ensight/NACA0015_MB_G/15ms_PLANE_B_PA_300/rear/15ms_PLANE_B_PA_300_000053.T000.D000.P007.H000.L.vec", path "C:/Users/PIV/Documents/mike_ensight/NACA0015_MB_G/15ms_PLANE_B_PA_300/rear/15ms_PLANE_B_PA_300_000054.T000.D000.P007.H000.L.vec", path "C:/Users/PIV/Documents/mike_ensight/NACA0015_MB_G/15ms_PLANE_B_PA_300/rear/15ms_PLANE_B_PA_300_000055.T000.D000.P007.H000.L.vec", path "C:/Users/PIV/Documents/mike_ensight/NACA0015_MB_G/15ms_PLANE_B_PA_300/rear/15ms_PLANE_B_PA_300_000056.T000.D000.P007.H000.L.vec", path "C:/Users/PIV/Documents/mike_ensight/NACA0015_MB_G/15ms_PLANE_B_PA_300/rear/15ms_PLANE_B_PA_300_000057.T000.D000.P007.H000.L.vec", path "C:/Users/PIV/Documents/mike_ensight/NACA0015_MB_G/15ms_PLANE_B_PA_300/rear/15ms_PLANE_B_PA_300_000058.T000.D000.P007.H000.L.vec", path "C:/Users/PIV/Documents/mike_ensight/NACA0015_MB_G/15ms_PLANE_B_PA_300/rear/15ms_PLANE_B_PA_300_000059.T000.D000.P007.H000.L.vec", path "C:/Users/PIV/Documents/mike_ensight/NACA0015_MB_G/15ms_PLANE_B_PA_300/rear/15ms_PLANE_B_PA_300_000060.T000.D000.P007.H000.L.vec", path "C:/Users/PIV/Documents/mike_ensight/NACA0015_MB_G/15ms_PLANE_B_PA_300/rear/15ms_PLANE_B_PA_300_000061.T000.D000.P007.H000.L.vec", path "C:/Users/PIV/Documents/mike_ensight/NACA0015_MB_G/15ms_PLANE_B_PA_300/rear/15ms_PLANE_B_PA_300_000062.T000.D000.P007.H000.L.vec", path "C:/Users/PIV/Documents/mike_ensight/NACA0015_MB_G/15ms_PLANE_B_PA_300/rear/15ms_PLANE_B_PA_300_000063.T000.D000.P007.H000.L.vec", path "C:/Users/PIV/Documents/mike_ensight/NACA0015_MB_G/15ms_PLANE_B_PA_300/rear/15ms_PLANE_B_PA_300_000064.T000.D000.P007.H000.L.vec", path "C:/Users/PIV/Documents/mike_ensight/NACA0015_MB_G/15ms_PLANE_B_PA_300/rear/15ms_PLANE_B_PA_300_000065.T000.D000.P007.H000.L.vec", path "C:/Users/PIV/Documents/mike_ensight/NACA0015_MB_G/15ms_PLANE_B_PA_300/rear/15ms_PLANE_B_PA_300_000066.T000.D000.P007.H000.L.vec", path "C:/Users/PIV/Documents/mike_ensight/NACA0015_MB_G/15ms_PLANE_B_PA_300/rear/15ms_PLANE_B_PA_300_000067.T000.D000.P007.H000.L.vec", path "C:/Users/PIV/Documents/mike_ensight/NACA0015_MB_G/15ms_PLANE_B_PA_300/rear/15ms_PLANE_B_PA_300_000068.T000.D000.P007.H000.L.vec", path "C:/Users/PIV/Documents/mike_ensight/NACA0015_MB_G/15ms_PLANE_B_PA_300/rear/15ms_PLANE_B_PA_300_000069.T000.D000.P007.H000.L.vec", path "C:/Users/PIV/Documents/mike_ensight/NACA0015_MB_G/15ms_PLANE_B_PA_300/rear/15ms_PLANE_B_PA_300_000070.T000.D000.P007.H000.L.vec", path "C:/Users/PIV/Documents/mike_ensight/NACA0015_MB_G/15ms_PLANE_B_PA_300/rear/15ms_PLANE_B_PA_300_000071.T000.D000.P007.H000.L.vec", path "C:/Users/PIV/Documents/mike_ensight/NACA0015_MB_G/15ms_PLANE_B_PA_300/rear/15ms_PLANE_B_PA_300_000072.T000.D000.P007.H000.L.vec", path "C:/Users/PIV/Documents/mike_ensight/NACA0015_MB_G/15ms_PLANE_B_PA_300/rear/15ms_PLANE_B_PA_300_000073.T000.D000.P007.H000.L.vec", path "C:/Users/PIV/Documents/mike_ensight/NACA0015_MB_G/15ms_PLANE_B_PA_300/rear/15ms_PLANE_B_PA_300_000074.T000.D000.P007.H000.L.vec", path "C:/Users/PIV/Documents/mike_ensight/NACA0015_MB_G/15ms_PLANE_B_PA_300/rear/15ms_PLANE_B_PA_300_000075.T000.D000.P007.H000.L.vec", path "C:/Users/PIV/Documents/mike_ensight/NACA0015_MB_G/15ms_PLANE_B_PA_300/rear/15ms_PLANE_B_PA_300_000076.T000.D000.P007.H000.L.vec", path "C:/Users/PIV/Documents/mike_ensight/NACA0015_MB_G/15ms_PLANE_B_PA_300/rear/15ms_PLANE_B_PA_300_000077.T000.D000.P007.H000.L.vec", path "C:/Users/PIV/Documents/mike_ensight/NACA0015_MB_G/15ms_PLANE_B_PA_300/rear/15ms_PLANE_B_PA_300_000078.T000.D000.P007.H000.L.vec", path "C:/Users/PIV/Documents/mike_ensight/NACA0015_MB_G/15ms_PLANE_B_PA_300/rear/15ms_PLANE_B_PA_300_000079.T000.D000.P007.H000.L.vec", path "C:/Users/PIV/Documents/mike_ensight/NACA0015_MB_G/15ms_PLANE_B_PA_300/rear/15ms_PLANE_B_PA_300_000080.T000.D000.P007.H000.L.vec", path "C:/Users/PIV/Documents/mike_ensight/NACA0015_MB_G/15ms_PLANE_B_PA_300/rear/15ms_PLANE_B_PA_300_000081.T000.D000.P007.H000.L.vec", path "C:/Users/PIV/Documents/mike_ensight/NACA0015_MB_G/15ms_PLANE_B_PA_300/rear/15ms_PLANE_B_PA_300_000082.T000.D000.P007.H000.L.vec", path "C:/Users/PIV/Documents/mike_ensight/NACA0015_MB_G/15ms_PLANE_B_PA_300/rear/15ms_PLANE_B_PA_300_000083.T000.D000.P007.H000.L.vec", path "C:/Users/PIV/Documents/mike_ensight/NACA0015_MB_G/15ms_PLANE_B_PA_300/rear/15ms_PLANE_B_PA_300_000084.T000.D000.P007.H000.L.vec", path "C:/Users/PIV/Documents/mike_ensight/NACA0015_MB_G/15ms_PLANE_B_PA_300/rear/15ms_PLANE_B_PA_300_000085.T000.D000.P007.H000.L.vec", path "C:/Users/PIV/Documents/mike_ensight/NACA0015_MB_G/15ms_PLANE_B_PA_300/rear/15ms_PLANE_B_PA_300_000086.T000.D000.P007.H000.L.vec", path "C:/Users/PIV/Documents/mike_ensight/NACA0015_MB_G/15ms_PLANE_B_PA_300/rear/15ms_PLANE_B_PA_300_000087.T000.D000.P007.H000.L.vec", path "C:/Users/PIV/Documents/mike_ensight/NACA0015_MB_G/15ms_PLANE_B_PA_300/rear/15ms_PLANE_B_PA_300_000088.T000.D000.P007.H000.L.vec", path "C:/Users/PIV/Documents/mike_ensight/NACA0015_MB_G/15ms_PLANE_B_PA_300/rear/15ms_PLANE_B_PA_300_000089.T000.D000.P007.H000.L.vec", path "C:/Users/PIV/Documents/mike_ensight/NACA0015_MB_G/15ms_PLANE_B_PA_300/rear/15ms_PLANE_B_PA_300_000090.T000.D000.P007.H000.L.vec", path "C:/Users/PIV/Documents/mike_ensight/NACA0015_MB_G/15ms_PLANE_B_PA_300/rear/15ms_PLANE_B_PA_300_000091.T000.D000.P007.H000.L.vec", path "C:/Users/PIV/Documents/mike_ensight/NACA0015_MB_G/15ms_PLANE_B_PA_300/rear/15ms_PLANE_B_PA_300_000092.T000.D000.P007.H000.L.vec", path "C:/Users/PIV/Documents/mike_ensight/NACA0015_MB_G/15ms_PLANE_B_PA_300/rear/15ms_PLANE_B_PA_300_000093.T000.D000.P007.H000.L.vec", path "C:/Users/PIV/Documents/mike_ensight/NACA0015_MB_G/15ms_PLANE_B_PA_300/rear/15ms_PLANE_B_PA_300_000094.T000.D000.P007.H000.L.vec", path "C:/Users/PIV/Documents/mike_ensight/NACA0015_MB_G/15ms_PLANE_B_PA_300/rear/15ms_PLANE_B_PA_300_000095.T000.D000.P007.H000.L.vec", path "C:/Users/PIV/Documents/mike_ensight/NACA0015_MB_G/15ms_PLANE_B_PA_300/rear/15ms_PLANE_B_PA_300_000096.T000.D000.P007.H000.L.vec", path "C:/Users/PIV/Documents/mike_ensight/NACA0015_MB_G/15ms_PLANE_B_PA_300/rear/15ms_PLANE_B_PA_300_000097.T000.D000.P007.H000.L.vec", path "C:/Users/PIV/Documents/mike_ensight/NACA0015_MB_G/15ms_PLANE_B_PA_300/rear/15ms_PLANE_B_PA_300_000098.T000.D000.P007.H000.L.vec", path "C:/Users/PIV/Documents/mike_ensight/NACA0015_MB_G/15ms_PLANE_B_PA_300/rear/15ms_PLANE_B_PA_300_000099.T000.D000.P007.H000.L.vec", path "C:/Users/PIV/Documents/mike_ensight/NACA0015_MB_G/15ms_PLANE_B_PA_300/rear/15ms_PLANE_B_PA_300_000100.T000.D000.P007.H000.L.vec", path "C:/Users/PIV/Documents/mike_ensight/NACA0015_MB_G/15ms_PLANE_B_PA_300/rear/15ms_PLANE_B_PA_300_000101.T000.D000.P007.H000.L.vec", path "C:/Users/PIV/Documents/mike_ensight/NACA0015_MB_G/15ms_PLANE_B_PA_300/rear/15ms_PLANE_B_PA_300_000102.T000.D000.P007.H000.L.vec", path "C:/Users/PIV/Documents/mike_ensight/NACA0015_MB_G/15ms_PLANE_B_PA_300/rear/15ms_PLANE_B_PA_300_000103.T000.D000.P007.H000.L.vec", path "C:/Users/PIV/Documents/mike_ensight/NACA0015_MB_G/15ms_PLANE_B_PA_300/rear/15ms_PLANE_B_PA_300_000104.T000.D000.P007.H000.L.vec", path "C:/Users/PIV/Documents/mike_ensight/NACA0015_MB_G/15ms_PLANE_B_PA_300/rear/15ms_PLANE_B_PA_300_000105.T000.D000.P007.H000.L.vec", path "C:/Users/PIV/Documents/mike_ensight/NACA0015_MB_G/15ms_PLANE_B_PA_300/rear/15ms_PLANE_B_PA_300_000106.T000.D000.P007.H000.L.vec", path "C:/Users/PIV/Documents/mike_ensight/NACA0015_MB_G/15ms_PLANE_B_PA_300/rear/15ms_PLANE_B_PA_300_000107.T000.D000.P007.H000.L.vec", path "C:/Users/PIV/Documents/mike_ensight/NACA0015_MB_G/15ms_PLANE_B_PA_300/rear/15ms_PLANE_B_PA_300_000108.T000.D000.P007.H000.L.vec", path "C:/Users/PIV/Documents/mike_ensight/NACA0015_MB_G/15ms_PLANE_B_PA_300/rear/15ms_PLANE_B_PA_300_000109.T000.D000.P007.H000.L.vec", path "C:/Users/PIV/Documents/mike_ensight/NACA0015_MB_G/15ms_PLANE_B_PA_300/rear/15ms_PLANE_B_PA_300_000110.T000.D000.P007.H000.L.vec", path "C:/Users/PIV/Documents/mike_ensight/NACA0015_MB_G/15ms_PLANE_B_PA_300/rear/15ms_PLANE_B_PA_300_000111.T000.D000.P007.H000.L.vec", path "C:/Users/PIV/Documents/mike_ensight/NACA0015_MB_G/15ms_PLANE_B_PA_300/rear/15ms_PLANE_B_PA_300_000112.T000.D000.P007.H000.L.vec", path "C:/Users/PIV/Documents/mike_ensight/NACA0015_MB_G/15ms_PLANE_B_PA_300/rear/15ms_PLANE_B_PA_300_000113.T000.D000.P007.H000.L.vec", path "C:/Users/PIV/Documents/mike_ensight/NACA0015_MB_G/15ms_PLANE_B_PA_300/rear/15ms_PLANE_B_PA_300_000114.T000.D000.P007.H000.L.vec", path "C:/Users/PIV/Documents/mike_ensight/NACA0015_MB_G/15ms_PLANE_B_PA_300/rear/15ms_PLANE_B_PA_300_000115.T000.D000.P007.H000.L.vec", path "C:/Users/PIV/Documents/mike_ensight/NACA0015_MB_G/15ms_PLANE_B_PA_300/rear/15ms_PLANE_B_PA_300_000116.T000.D000.P007.H000.L.vec", path "C:/Users/PIV/Documents/mike_ensight/NACA0015_MB_G/15ms_PLANE_B_PA_300/rear/15ms_PLANE_B_PA_300_000117.T000.D000.P007.H000.L.vec", path "C:/Users/PIV/Documents/mike_ensight/NACA0015_MB_G/15ms_PLANE_B_PA_300/rear/15ms_PLANE_B_PA_300_000118.T000.D000.P007.H000.L.vec", path "C:/Users/PIV/Documents/mike_ensight/NACA0015_MB_G/15ms_PLANE_B_PA_300/rear/15ms_PLANE_B_PA_300_000119.T000.D000.P007.H000.L.vec", path "C:/Users/PIV/Documents/mike_ensight/NACA0015_MB_G/15ms_PLANE_B_PA_300/rear/15ms_PLANE_B_PA_300_000120.T000.D000.P007.H000.L.vec", path "C:/Users/PIV/Documents/mike_ensight/NACA0015_MB_G/15ms_PLANE_B_PA_300/rear/15ms_PLANE_B_PA_300_000121.T000.D000.P007.H000.L.vec", path "C:/Users/PIV/Documents/mike_ensight/NACA0015_MB_G/15ms_PLANE_B_PA_300/rear/15ms_PLANE_B_PA_300_000122.T000.D000.P007.H000.L.vec", path "C:/Users/PIV/Documents/mike_ensight/NACA0015_MB_G/15ms_PLANE_B_PA_300/rear/15ms_PLANE_B_PA_300_000123.T000.D000.P007.H000.L.vec", path "C:/Users/PIV/Documents/mike_ensight/NACA0015_MB_G/15ms_PLANE_B_PA_300/rear/15ms_PLANE_B_PA_300_000124.T000.D000.P007.H000.L.vec", path "C:/Users/PIV/Documents/mike_ensight/NACA0015_MB_G/15ms_PLANE_B_PA_300/rear/15ms_PLANE_B_PA_300_000125.T000.D000.P007.H000.L.vec", path "C:/Users/PIV/Documents/mike_ensight/NACA0015_MB_G/15ms_PLANE_B_PA_300/rear/15ms_PLANE_B_PA_300_000126.T000.D000.P007.H000.L.vec", path "C:/Users/PIV/Documents/mike_ensight/NACA0015_MB_G/15ms_PLANE_B_PA_300/rear/15ms_PLANE_B_PA_300_000127.T000.D000.P007.H000.L.vec", path "C:/Users/PIV/Documents/mike_ensight/NACA0015_MB_G/15ms_PLANE_B_PA_300/rear/15ms_PLANE_B_PA_300_000128.T000.D000.P007.H000.L.vec", path "C:/Users/PIV/Documents/mike_ensight/NACA0015_MB_G/15ms_PLANE_B_PA_300/rear/15ms_PLANE_B_PA_300_000129.T000.D000.P007.H000.L.vec", path "C:/Users/PIV/Documents/mike_ensight/NACA0015_MB_G/15ms_PLANE_B_PA_300/rear/15ms_PLANE_B_PA_300_000130.T000.D000.P007.H000.L.vec", path "C:/Users/PIV/Documents/mike_ensight/NACA0015_MB_G/15ms_PLANE_B_PA_300/rear/15ms_PLANE_B_PA_300_000131.T000.D000.P007.H000.L.vec", path "C:/Users/PIV/Documents/mike_ensight/NACA0015_MB_G/15ms_PLANE_B_PA_300/rear/15ms_PLANE_B_PA_300_000132.T000.D000.P007.H000.L.vec", path "C:/Users/PIV/Documents/mike_ensight/NACA0015_MB_G/15ms_PLANE_B_PA_300/rear/15ms_PLANE_B_PA_300_000133.T000.D000.P007.H000.L.vec", path "C:/Users/PIV/Documents/mike_ensight/NACA0015_MB_G/15ms_PLANE_B_PA_300/rear/15ms_PLANE_B_PA_300_000134.T000.D000.P007.H000.L.vec", path "C:/Users/PIV/Documents/mike_ensight/NACA0015_MB_G/15ms_PLANE_B_PA_300/rear/15ms_PLANE_B_PA_300_000135.T000.D000.P007.H000.L.vec", path "C:/Users/PIV/Documents/mike_ensight/NACA0015_MB_G/15ms_PLANE_B_PA_300/rear/15ms_PLANE_B_PA_300_000136.T000.D000.P007.H000.L.vec", path "C:/Users/PIV/Documents/mike_ensight/NACA0015_MB_G/15ms_PLANE_B_PA_300/rear/15ms_PLANE_B_PA_300_000137.T000.D000.P007.H000.L.vec", path "C:/Users/PIV/Documents/mike_ensight/NACA0015_MB_G/15ms_PLANE_B_PA_300/rear/15ms_PLANE_B_PA_300_000138.T000.D000.P007.H000.L.vec", path "C:/Users/PIV/Documents/mike_ensight/NACA0015_MB_G/15ms_PLANE_B_PA_300/rear/15ms_PLANE_B_PA_300_000139.T000.D000.P007.H000.L.vec", path "C:/Users/PIV/Documents/mike_ensight/NACA0015_MB_G/15ms_PLANE_B_PA_300/rear/15ms_PLANE_B_PA_300_000140.T000.D000.P007.H000.L.vec", path "C:/Users/PIV/Documents/mike_ensight/NACA0015_MB_G/15ms_PLANE_B_PA_300/rear/15ms_PLANE_B_PA_300_000141.T000.D000.P007.H000.L.vec", path "C:/Users/PIV/Documents/mike_ensight/NACA0015_MB_G/15ms_PLANE_B_PA_300/rear/15ms_PLANE_B_PA_300_000142.T000.D000.P007.H000.L.vec", path "C:/Users/PIV/Documents/mike_ensight/NACA0015_MB_G/15ms_PLANE_B_PA_300/rear/15ms_PLANE_B_PA_300_000143.T000.D000.P007.H000.L.vec", path "C:/Users/PIV/Documents/mike_ensight/NACA0015_MB_G/15ms_PLANE_B_PA_300/rear/15ms_PLANE_B_PA_300_000144.T000.D000.P007.H000.L.vec", path "C:/Users/PIV/Documents/mike_ensight/NACA0015_MB_G/15ms_PLANE_B_PA_300/rear/15ms_PLANE_B_PA_300_000145.T000.D000.P007.H000.L.vec", path "C:/Users/PIV/Documents/mike_ensight/NACA0015_MB_G/15ms_PLANE_B_PA_300/rear/15ms_PLANE_B_PA_300_000146.T000.D000.P007.H000.L.vec", path "C:/Users/PIV/Documents/mike_ensight/NACA0015_MB_G/15ms_PLANE_B_PA_300/rear/15ms_PLANE_B_PA_300_000147.T000.D000.P007.H000.L.vec", path "C:/Users/PIV/Documents/mike_ensight/NACA0015_MB_G/15ms_PLANE_B_PA_300/rear/15ms_PLANE_B_PA_300_000148.T000.D000.P007.H000.L.vec", path "C:/Users/PIV/Documents/mike_ensight/NACA0015_MB_G/15ms_PLANE_B_PA_300/rear/15ms_PLANE_B_PA_300_000149.T000.D000.P007.H000.L.vec", path "C:/Users/PIV/Documents/mike_ensight/NACA0015_MB_G/15ms_PLANE_B_PA_300/rear/15ms_PLANE_B_PA_300_000150.T000.D000.P007.H000.L.vec", path "C:/Users/PIV/Documents/mike_ensight/NACA0015_MB_G/15ms_PLANE_B_PA_300/rear/15ms_PLANE_B_PA_300_000151.T000.D000.P007.H000.L.vec", path "C:/Users/PIV/Documents/mike_ensight/NACA0015_MB_G/15ms_PLANE_B_PA_300/rear/15ms_PLANE_B_PA_300_000152.T000.D000.P007.H000.L.vec", path "C:/Users/PIV/Documents/mike_ensight/NACA0015_MB_G/15ms_PLANE_B_PA_300/rear/15ms_PLANE_B_PA_300_000153.T000.D000.P007.H000.L.vec", path "C:/Users/PIV/Documents/mike_ensight/NACA0015_MB_G/15ms_PLANE_B_PA_300/rear/15ms_PLANE_B_PA_300_000154.T000.D000.P007.H000.L.vec", path "C:/Users/PIV/Documents/mike_ensight/NACA0015_MB_G/15ms_PLANE_B_PA_300/rear/15ms_PLANE_B_PA_300_000155.T000.D000.P007.H000.L.vec", path "C:/Users/PIV/Documents/mike_ensight/NACA0015_MB_G/15ms_PLANE_B_PA_300/rear/15ms_PLANE_B_PA_300_000156.T000.D000.P007.H000.L.vec", path "C:/Users/PIV/Documents/mike_ensight/NACA0015_MB_G/15ms_PLANE_B_PA_300/rear/15ms_PLANE_B_PA_300_000157.T000.D000.P007.H000.L.vec", path "C:/Users/PIV/Documents/mike_ensight/NACA0015_MB_G/15ms_PLANE_B_PA_300/rear/15ms_PLANE_B_PA_300_000158.T000.D000.P007.H000.L.vec", path "C:/Users/PIV/Documents/mike_ensight/NACA0015_MB_G/15ms_PLANE_B_PA_300/rear/15ms_PLANE_B_PA_300_000159.T000.D000.P007.H000.L.vec", path "C:/Users/PIV/Documents/mike_ensight/NACA0015_MB_G/15ms_PLANE_B_PA_300/rear/15ms_PLANE_B_PA_300_000160.T000.D000.P007.H000.L.vec", path "C:/Users/PIV/Documents/mike_ensight/NACA0015_MB_G/15ms_PLANE_B_PA_300/rear/15ms_PLANE_B_PA_300_000161.T000.D000.P007.H000.L.vec", path "C:/Users/PIV/Documents/mike_ensight/NACA0015_MB_G/15ms_PLANE_B_PA_300/rear/15ms_PLANE_B_PA_300_000162.T000.D000.P007.H000.L.vec", path "C:/Users/PIV/Documents/mike_ensight/NACA0015_MB_G/15ms_PLANE_B_PA_300/rear/15ms_PLANE_B_PA_300_000163.T000.D000.P007.H000.L.vec", path "C:/Users/PIV/Documents/mike_ensight/NACA0015_MB_G/15ms_PLANE_B_PA_300/rear/15ms_PLANE_B_PA_300_000164.T000.D000.P007.H000.L.vec", path "C:/Users/PIV/Documents/mike_ensight/NACA0015_MB_G/15ms_PLANE_B_PA_300/rear/15ms_PLANE_B_PA_300_000165.T000.D000.P007.H000.L.vec", path "C:/Users/PIV/Documents/mike_ensight/NACA0015_MB_G/15ms_PLANE_B_PA_300/rear/15ms_PLANE_B_PA_300_000166.T000.D000.P007.H000.L.vec", path "C:/Users/PIV/Documents/mike_ensight/NACA0015_MB_G/15ms_PLANE_B_PA_300/rear/15ms_PLANE_B_PA_300_000167.T000.D000.P007.H000.L.vec", path "C:/Users/PIV/Documents/mike_ensight/NACA0015_MB_G/15ms_PLANE_B_PA_300/rear/15ms_PLANE_B_PA_300_000168.T000.D000.P007.H000.L.vec", path "C:/Users/PIV/Documents/mike_ensight/NACA0015_MB_G/15ms_PLANE_B_PA_300/rear/15ms_PLANE_B_PA_300_000169.T000.D000.P007.H000.L.vec", path "C:/Users/PIV/Documents/mike_ensight/NACA0015_MB_G/15ms_PLANE_B_PA_300/rear/15ms_PLANE_B_PA_300_000170.T000.D000.P007.H000.L.vec", path "C:/Users/PIV/Documents/mike_ensight/NACA0015_MB_G/15ms_PLANE_B_PA_300/rear/15ms_PLANE_B_PA_300_000171.T000.D000.P007.H000.L.vec", path "C:/Users/PIV/Documents/mike_ensight/NACA0015_MB_G/15ms_PLANE_B_PA_300/rear/15ms_PLANE_B_PA_300_000172.T000.D000.P007.H000.L.vec", path "C:/Users/PIV/Documents/mike_ensight/NACA0015_MB_G/15ms_PLANE_B_PA_300/rear/15ms_PLANE_B_PA_300_000173.T000.D000.P007.H000.L.vec", path "C:/Users/PIV/Documents/mike_ensight/NACA0015_MB_G/15ms_PLANE_B_PA_300/rear/15ms_PLANE_B_PA_300_000174.T000.D000.P007.H000.L.vec", path "C:/Users/PIV/Documents/mike_ensight/NACA0015_MB_G/15ms_PLANE_B_PA_300/rear/15ms_PLANE_B_PA_300_000175.T000.D000.P007.H000.L.vec", path "C:/Users/PIV/Documents/mike_ensight/NACA0015_MB_G/15ms_PLANE_B_PA_300/rear/15ms_PLANE_B_PA_300_000176.T000.D000.P007.H000.L.vec", path "C:/Users/PIV/Documents/mike_ensight/NACA0015_MB_G/15ms_PLANE_B_PA_300/rear/15ms_PLANE_B_PA_300_000177.T000.D000.P007.H000.L.vec", path "C:/Users/PIV/Documents/mike_ensight/NACA0015_MB_G/15ms_PLANE_B_PA_300/rear/15ms_PLANE_B_PA_300_000178.T000.D000.P007.H000.L.vec", path "C:/Users/PIV/Documents/mike_ensight/NACA0015_MB_G/15ms_PLANE_B_PA_300/rear/15ms_PLANE_B_PA_300_000179.T000.D000.P007.H000.L.vec", path "C:/Users/PIV/Documents/mike_ensight/NACA0015_MB_G/15ms_PLANE_B_PA_300/rear/15ms_PLANE_B_PA_300_000180.T000.D000.P007.H000.L.vec", path "C:/Users/PIV/Documents/mike_ensight/NACA0015_MB_G/15ms_PLANE_B_PA_300/rear/15ms_PLANE_B_PA_300_000181.T000.D000.P007.H000.L.vec", path "C:/Users/PIV/Documents/mike_ensight/NACA0015_MB_G/15ms_PLANE_B_PA_300/rear/15ms_PLANE_B_PA_300_000182.T000.D000.P007.H000.L.vec", path "C:/Users/PIV/Documents/mike_ensight/NACA0015_MB_G/15ms_PLANE_B_PA_300/rear/15ms_PLANE_B_PA_300_000183.T000.D000.P007.H000.L.vec", path "C:/Users/PIV/Documents/mike_ensight/NACA0015_MB_G/15ms_PLANE_B_PA_300/rear/15ms_PLANE_B_PA_300_000184.T000.D000.P007.H000.L.vec", path "C:/Users/PIV/Documents/mike_ensight/NACA0015_MB_G/15ms_PLANE_B_PA_300/rear/15ms_PLANE_B_PA_300_000185.T000.D000.P007.H000.L.vec", path "C:/Users/PIV/Documents/mike_ensight/NACA0015_MB_G/15ms_PLANE_B_PA_300/rear/15ms_PLANE_B_PA_300_000186.T000.D000.P007.H000.L.vec", path "C:/Users/PIV/Documents/mike_ensight/NACA0015_MB_G/15ms_PLANE_B_PA_300/rear/15ms_PLANE_B_PA_300_000187.T000.D000.P007.H000.L.vec", path "C:/Users/PIV/Documents/mike_ensight/NACA0015_MB_G/15ms_PLANE_B_PA_300/rear/15ms_PLANE_B_PA_300_000188.T000.D000.P007.H000.L.vec", path "C:/Users/PIV/Documents/mike_ensight/NACA0015_MB_G/15ms_PLANE_B_PA_300/rear/15ms_PLANE_B_PA_300_000189.T000.D000.P007.H000.L.vec", path "C:/Users/PIV/Documents/mike_ensight/NACA0015_MB_G/15ms_PLANE_B_PA_300/rear/15ms_PLANE_B_PA_300_000190.T000.D000.P007.H000.L.vec", path "C:/Users/PIV/Documents/mike_ensight/NACA0015_MB_G/15ms_PLANE_B_PA_300/rear/15ms_PLANE_B_PA_300_000191.T000.D000.P007.H000.L.vec", path "C:/Users/PIV/Documents/mike_ensight/NACA0015_MB_G/15ms_PLANE_B_PA_300/rear/15ms_PLANE_B_PA_300_000192.T000.D000.P007.H000.L.vec", path "C:/Users/PIV/Documents/mike_ensight/NACA0015_MB_G/15ms_PLANE_B_PA_300/rear/15ms_PLANE_B_PA_300_000193.T000.D000.P007.H000.L.vec", path "C:/Users/PIV/Documents/mike_ensight/NACA0015_MB_G/15ms_PLANE_B_PA_300/rear/15ms_PLANE_B_PA_300_000194.T000.D000.P007.H000.L.vec", path "C:/Users/PIV/Documents/mike_ensight/NACA0015_MB_G/15ms_PLANE_B_PA_300/rear/15ms_PLANE_B_PA_300_000195.T000.D000.P007.H000.L.vec", path "C:/Users/PIV/Documents/mike_ensight/NACA0015_MB_G/15ms_PLANE_B_PA_300/rear/15ms_PLANE_B_PA_300_000196.T000.D000.P007.H000.L.vec", path "C:/Users/PIV/Documents/mike_ensight/NACA0015_MB_G/15ms_PLANE_B_PA_300/rear/15ms_PLANE_B_PA_300_000197.T000.D000.P007.H000.L.vec", path "C:/Users/PIV/Documents/mike_ensight/NACA0015_MB_G/15ms_PLANE_B_PA_300/rear/15ms_PLANE_B_PA_300_000198.T000.D000.P007.H000.L.vec", path "C:/Users/PIV/Documents/mike_ensight/NACA0015_MB_G/15ms_PLANE_B_PA_300/rear/15ms_PLANE_B_PA_300_000199.T000.D000.P007.H000.L.vec", path "C:/Users/PIV/Documents/mike_ensight/NACA0015_MB_G/15ms_PLANE_B_PA_300/rear/15ms_PLANE_B_PA_300_000200.T000.D000.P007.H000.L.vec", path "C:/Users/PIV/Documents/mike_ensight/NACA0015_MB_G/15ms_PLANE_B_PA_300/rear/15ms_PLANE_B_PA_300_000201.T000.D000.P007.H000.L.vec", path "C:/Users/PIV/Documents/mike_ensight/NACA0015_MB_G/15ms_PLANE_B_PA_300/rear/15ms_PLANE_B_PA_300_000202.T000.D000.P007.H000.L.vec", path "C:/Users/PIV/Documents/mike_ensight/NACA0015_MB_G/15ms_PLANE_B_PA_300/rear/15ms_PLANE_B_PA_300_000203.T000.D000.P007.H000.L.vec", path "C:/Users/PIV/Documents/mike_ensight/NACA0015_MB_G/15ms_PLANE_B_PA_300/rear/15ms_PLANE_B_PA_300_000204.T000.D000.P007.H000.L.vec", path "C:/Users/PIV/Documents/mike_ensight/NACA0015_MB_G/15ms_PLANE_B_PA_300/rear/15ms_PLANE_B_PA_300_000205.T000.D000.P007.H000.L.vec", path "C:/Users/PIV/Documents/mike_ensight/NACA0015_MB_G/15ms_PLANE_B_PA_300/rear/15ms_PLANE_B_PA_300_000206.T000.D000.P007.H000.L.vec", path "C:/Users/PIV/Documents/mike_ensight/NACA0015_MB_G/15ms_PLANE_B_PA_300/rear/15ms_PLANE_B_PA_300_000207.T000.D000.P007.H000.L.vec", path "C:/Users/PIV/Documents/mike_ensight/NACA0015_MB_G/15ms_PLANE_B_PA_300/rear/15ms_PLANE_B_PA_300_000208.T000.D000.P007.H000.L.vec", path "C:/Users/PIV/Documents/mike_ensight/NACA0015_MB_G/15ms_PLANE_B_PA_300/rear/15ms_PLANE_B_PA_300_000209.T000.D000.P007.H000.L.vec", path "C:/Users/PIV/Documents/mike_ensight/NACA0015_MB_G/15ms_PLANE_B_PA_300/rear/15ms_PLANE_B_PA_300_000210.T000.D000.P007.H000.L.vec", path "C:/Users/PIV/Documents/mike_ensight/NACA0015_MB_G/15ms_PLANE_B_PA_300/rear/15ms_PLANE_B_PA_300_000211.T000.D000.P007.H000.L.vec", path "C:/Users/PIV/Documents/mike_ensight/NACA0015_MB_G/15ms_PLANE_B_PA_300/rear/15ms_PLANE_B_PA_300_000212.T000.D000.P007.H000.L.vec", path "C:/Users/PIV/Documents/mike_ensight/NACA0015_MB_G/15ms_PLANE_B_PA_300/rear/15ms_PLANE_B_PA_300_000213.T000.D000.P007.H000.L.vec", path "C:/Users/PIV/Documents/mike_ensight/NACA0015_MB_G/15ms_PLANE_B_PA_300/rear/15ms_PLANE_B_PA_300_000214.T000.D000.P007.H000.L.vec", path "C:/Users/PIV/Documents/mike_ensight/NACA0015_MB_G/15ms_PLANE_B_PA_300/rear/15ms_PLANE_B_PA_300_000215.T000.D000.P007.H000.L.vec", path "C:/Users/PIV/Documents/mike_ensight/NACA0015_MB_G/15ms_PLANE_B_PA_300/rear/15ms_PLANE_B_PA_300_000216.T000.D000.P007.H000.L.vec", path "C:/Users/PIV/Documents/mike_ensight/NACA0015_MB_G/15ms_PLANE_B_PA_300/rear/15ms_PLANE_B_PA_300_000217.T000.D000.P007.H000.L.vec", path "C:/Users/PIV/Documents/mike_ensight/NACA0015_MB_G/15ms_PLANE_B_PA_300/rear/15ms_PLANE_B_PA_300_000218.T000.D000.P007.H000.L.vec", path "C:/Users/PIV/Documents/mike_ensight/NACA0015_MB_G/15ms_PLANE_B_PA_300/rear/15ms_PLANE_B_PA_300_000219.T000.D000.P007.H000.L.vec", path "C:/Users/PIV/Documents/mike_ensight/NACA0015_MB_G/15ms_PLANE_B_PA_300/rear/15ms_PLANE_B_PA_300_000220.T000.D000.P007.H000.L.vec", path "C:/Users/PIV/Documents/mike_ensight/NACA0015_MB_G/15ms_PLANE_B_PA_300/rear/15ms_PLANE_B_PA_300_000221.T000.D000.P007.H000.L.vec", path "C:/Users/PIV/Documents/mike_ensight/NACA0015_MB_G/15ms_PLANE_B_PA_300/rear/15ms_PLANE_B_PA_300_000222.T000.D000.P007.H000.L.vec", path "C:/Users/PIV/Documents/mike_ensight/NACA0015_MB_G/15ms_PLANE_B_PA_300/rear/15ms_PLANE_B_PA_300_000223.T000.D000.P007.H000.L.vec", path "C:/Users/PIV/Documents/mike_ensight/NACA0015_MB_G/15ms_PLANE_B_PA_300/rear/15ms_PLANE_B_PA_300_000224.T000.D000.P007.H000.L.vec", path "C:/Users/PIV/Documents/mike_ensight/NACA0015_MB_G/15ms_PLANE_B_PA_300/rear/15ms_PLANE_B_PA_300_000225.T000.D000.P007.H000.L.vec", path "C:/Users/PIV/Documents/mike_ensight/NACA0015_MB_G/15ms_PLANE_B_PA_300/rear/15ms_PLANE_B_PA_300_000226.T000.D000.P007.H000.L.vec", path "C:/Users/PIV/Documents/mike_ensight/NACA0015_MB_G/15ms_PLANE_B_PA_300/rear/15ms_PLANE_B_PA_300_000227.T000.D000.P007.H000.L.vec", path "C:/Users/PIV/Documents/mike_ensight/NACA0015_MB_G/15ms_PLANE_B_PA_300/rear/15ms_PLANE_B_PA_300_000228.T000.D000.P007.H000.L.vec", path "C:/Users/PIV/Documents/mike_ensight/NACA0015_MB_G/15ms_PLANE_B_PA_300/rear/15ms_PLANE_B_PA_300_000229.T000.D000.P007.H000.L.vec", path "C:/Users/PIV/Documents/mike_ensight/NACA0015_MB_G/15ms_PLANE_B_PA_300/rear/15ms_PLANE_B_PA_300_000230.T000.D000.P007.H000.L.vec", path "C:/Users/PIV/Documents/mike_ensight/NACA0015_MB_G/15ms_PLANE_B_PA_300/rear/15ms_PLANE_B_PA_300_000231.T000.D000.P007.H000.L.vec", path "C:/Users/PIV/Documents/mike_ensight/NACA0015_MB_G/15ms_PLANE_B_PA_300/rear/15ms_PLANE_B_PA_300_000232.T000.D000.P007.H000.L.vec", path "C:/Users/PIV/Documents/mike_ensight/NACA0015_MB_G/15ms_PLANE_B_PA_300/rear/15ms_PLANE_B_PA_300_000233.T000.D000.P007.H000.L.vec", path "C:/Users/PIV/Documents/mike_ensight/NACA0015_MB_G/15ms_PLANE_B_PA_300/rear/15ms_PLANE_B_PA_300_000234.T000.D000.P007.H000.L.vec", path "C:/Users/PIV/Documents/mike_ensight/NACA0015_MB_G/15ms_PLANE_B_PA_300/rear/15ms_PLANE_B_PA_300_000235.T000.D000.P007.H000.L.vec", path "C:/Users/PIV/Documents/mike_ensight/NACA0015_MB_G/15ms_PLANE_B_PA_300/rear/15ms_PLANE_B_PA_300_000236.T000.D000.P007.H000.L.vec", path "C:/Users/PIV/Documents/mike_ensight/NACA0015_MB_G/15ms_PLANE_B_PA_300/rear/15ms_PLANE_B_PA_300_000237.T000.D000.P007.H000.L.vec", path "C:/Users/PIV/Documents/mike_ensight/NACA0015_MB_G/15ms_PLANE_B_PA_300/rear/15ms_PLANE_B_PA_300_000238.T000.D000.P007.H000.L.vec", path "C:/Users/PIV/Documents/mike_ensight/NACA0015_MB_G/15ms_PLANE_B_PA_300/rear/15ms_PLANE_B_PA_300_000239.T000.D000.P007.H000.L.vec", path "C:/Users/PIV/Documents/mike_ensight/NACA0015_MB_G/15ms_PLANE_B_PA_300/rear/15ms_PLANE_B_PA_300_000240.T000.D000.P007.H000.L.vec", path "C:/Users/PIV/Documents/mike_ensight/NACA0015_MB_G/15ms_PLANE_B_PA_300/rear/15ms_PLANE_B_PA_300_000241.T000.D000.P007.H000.L.vec", path "C:/Users/PIV/Documents/mike_ensight/NACA0015_MB_G/15ms_PLANE_B_PA_300/rear/15ms_PLANE_B_PA_300_000242.T000.D000.P007.H000.L.vec", path "C:/Users/PIV/Documents/mike_ensight/NACA0015_MB_G/15ms_PLANE_B_PA_300/rear/15ms_PLANE_B_PA_300_000243.T000.D000.P007.H000.L.vec", path "C:/Users/PIV/Documents/mike_ensight/NACA0015_MB_G/15ms_PLANE_B_PA_300/rear/15ms_PLANE_B_PA_300_000244.T000.D000.P007.H000.L.vec", path "C:/Users/PIV/Documents/mike_ensight/NACA0015_MB_G/15ms_PLANE_B_PA_300/rear/15ms_PLANE_B_PA_300_000245.T000.D000.P007.H000.L.vec", path "C:/Users/PIV/Documents/mike_ensight/NACA0015_MB_G/15ms_PLANE_B_PA_300/rear/15ms_PLANE_B_PA_300_000246.T000.D000.P007.H000.L.vec", path "C:/Users/PIV/Documents/mike_ensight/NACA0015_MB_G/15ms_PLANE_B_PA_300/rear/15ms_PLANE_B_PA_300_000247.T000.D000.P007.H000.L.vec", path "C:/Users/PIV/Documents/mike_ensight/NACA0015_MB_G/15ms_PLANE_B_PA_300/rear/15ms_PLANE_B_PA_300_000248.T000.D000.P007.H000.L.vec", path "C:/Users/PIV/Documents/mike_ensight/NACA0015_MB_G/15ms_PLANE_B_PA_300/rear/15ms_PLANE_B_PA_300_000249.T000.D000.P007.H000.L.vec", path "C:/Users/PIV/Documents/mike_ensight/NACA0015_MB_G/15ms_PLANE_B_PA_300/rear/15ms_PLANE_B_PA_300_000250.T000.D000.P007.H000.L.vec", path "C:/Users/PIV/Documents/mike_ensight/NACA0015_MB_G/15ms_PLANE_B_PA_300/rear/15ms_PLANE_B_PA_300_000251.T000.D000.P007.H000.L.vec", path "C:/Users/PIV/Documents/mike_ensight/NACA0015_MB_G/15ms_PLANE_B_PA_300/rear/15ms_PLANE_B_PA_300_000252.T000.D000.P007.H000.L.vec", path "C:/Users/PIV/Documents/mike_ensight/NACA0015_MB_G/15ms_PLANE_B_PA_300/rear/15ms_PLANE_B_PA_300_000253.T000.D000.P007.H000.L.vec", path "C:/Users/PIV/Documents/mike_ensight/NACA0015_MB_G/15ms_PLANE_B_PA_300/rear/15ms_PLANE_B_PA_300_000254.T000.D000.P007.H000.L.vec", path "C:/Users/PIV/Documents/mike_ensight/NACA0015_MB_G/15ms_PLANE_B_PA_300/rear/15ms_PLANE_B_PA_300_000255.T000.D000.P007.H000.L.vec", path "C:/Users/PIV/Documents/mike_ensight/NACA0015_MB_G/15ms_PLANE_B_PA_300/rear/15ms_PLANE_B_PA_300_000256.T000.D000.P007.H000.L.vec", path "C:/Users/PIV/Documents/mike_ensight/NACA0015_MB_G/15ms_PLANE_B_PA_300/rear/15ms_PLANE_B_PA_300_000257.T000.D000.P007.H000.L.vec", path "C:/Users/PIV/Documents/mike_ensight/NACA0015_MB_G/15ms_PLANE_B_PA_300/rear/15ms_PLANE_B_PA_300_000258.T000.D000.P007.H000.L.vec", path "C:/Users/PIV/Documents/mike_ensight/NACA0015_MB_G/15ms_PLANE_B_PA_300/rear/15ms_PLANE_B_PA_300_000259.T000.D000.P007.H000.L.vec", path "C:/Users/PIV/Documents/mike_ensight/NACA0015_MB_G/15ms_PLANE_B_PA_300/rear/15ms_PLANE_B_PA_300_000260.T000.D000.P007.H000.L.vec", path "C:/Users/PIV/Documents/mike_ensight/NACA0015_MB_G/15ms_PLANE_B_PA_300/rear/15ms_PLANE_B_PA_300_000261.T000.D000.P007.H000.L.vec", path "C:/Users/PIV/Documents/mike_ensight/NACA0015_MB_G/15ms_PLANE_B_PA_300/rear/15ms_PLANE_B_PA_300_000262.T000.D000.P007.H000.L.vec", path "C:/Users/PIV/Documents/mike_ensight/NACA0015_MB_G/15ms_PLANE_B_PA_300/rear/15ms_PLANE_B_PA_300_000263.T000.D000.P007.H000.L.vec", path "C:/Users/PIV/Documents/mike_ensight/NACA0015_MB_G/15ms_PLANE_B_PA_300/rear/15ms_PLANE_B_PA_300_000264.T000.D000.P007.H000.L.vec", path "C:/Users/PIV/Documents/mike_ensight/NACA0015_MB_G/15ms_PLANE_B_PA_300/rear/15ms_PLANE_B_PA_300_000265.T000.D000.P007.H000.L.vec", path "C:/Users/PIV/Documents/mike_ensight/NACA0015_MB_G/15ms_PLANE_B_PA_300/rear/15ms_PLANE_B_PA_300_000266.T000.D000.P007.H000.L.vec", path "C:/Users/PIV/Documents/mike_ensight/NACA0015_MB_G/15ms_PLANE_B_PA_300/rear/15ms_PLANE_B_PA_300_000267.T000.D000.P007.H000.L.vec", path "C:/Users/PIV/Documents/mike_ensight/NACA0015_MB_G/15ms_PLANE_B_PA_300/rear/15ms_PLANE_B_PA_300_000268.T000.D000.P007.H000.L.vec", path "C:/Users/PIV/Documents/mike_ensight/NACA0015_MB_G/15ms_PLANE_B_PA_300/rear/15ms_PLANE_B_PA_300_000269.T000.D000.P007.H000.L.vec", path "C:/Users/PIV/Documents/mike_ensight/NACA0015_MB_G/15ms_PLANE_B_PA_300/rear/15ms_PLANE_B_PA_300_000270.T000.D000.P007.H000.L.vec", path "C:/Users/PIV/Documents/mike_ensight/NACA0015_MB_G/15ms_PLANE_B_PA_300/rear/15ms_PLANE_B_PA_300_000271.T000.D000.P007.H000.L.vec", path "C:/Users/PIV/Documents/mike_ensight/NACA0015_MB_G/15ms_PLANE_B_PA_300/rear/15ms_PLANE_B_PA_300_000272.T000.D000.P007.H000.L.vec", path "C:/Users/PIV/Documents/mike_ensight/NACA0015_MB_G/15ms_PLANE_B_PA_300/rear/15ms_PLANE_B_PA_300_000273.T000.D000.P007.H000.L.vec", path "C:/Users/PIV/Documents/mike_ensight/NACA0015_MB_G/15ms_PLANE_B_PA_300/rear/15ms_PLANE_B_PA_300_000274.T000.D000.P007.H000.L.vec", path "C:/Users/PIV/Documents/mike_ensight/NACA0015_MB_G/15ms_PLANE_B_PA_300/rear/15ms_PLANE_B_PA_300_000275.T000.D000.P007.H000.L.vec", path "C:/Users/PIV/Documents/mike_ensight/NACA0015_MB_G/15ms_PLANE_B_PA_300/rear/15ms_PLANE_B_PA_300_000276.T000.D000.P007.H000.L.vec", path "C:/Users/PIV/Documents/mike_ensight/NACA0015_MB_G/15ms_PLANE_B_PA_300/rear/15ms_PLANE_B_PA_300_000277.T000.D000.P007.H000.L.vec", path "C:/Users/PIV/Documents/mike_ensight/NACA0015_MB_G/15ms_PLANE_B_PA_300/rear/15ms_PLANE_B_PA_300_000278.T000.D000.P007.H000.L.vec", path "C:/Users/PIV/Documents/mike_ensight/NACA0015_MB_G/15ms_PLANE_B_PA_300/rear/15ms_PLANE_B_PA_300_000279.T000.D000.P007.H000.L.vec", path "C:/Users/PIV/Documents/mike_ensight/NACA0015_MB_G/15ms_PLANE_B_PA_300/rear/15ms_PLANE_B_PA_300_000280.T000.D000.P007.H000.L.vec", path "C:/Users/PIV/Documents/mike_ensight/NACA0015_MB_G/15ms_PLANE_B_PA_300/rear/15ms_PLANE_B_PA_300_000281.T000.D000.P007.H000.L.vec", path "C:/Users/PIV/Documents/mike_ensight/NACA0015_MB_G/15ms_PLANE_B_PA_300/rear/15ms_PLANE_B_PA_300_000282.T000.D000.P007.H000.L.vec", path "C:/Users/PIV/Documents/mike_ensight/NACA0015_MB_G/15ms_PLANE_B_PA_300/rear/15ms_PLANE_B_PA_300_000283.T000.D000.P007.H000.L.vec", path "C:/Users/PIV/Documents/mike_ensight/NACA0015_MB_G/15ms_PLANE_B_PA_300/rear/15ms_PLANE_B_PA_300_000284.T000.D000.P007.H000.L.vec", path "C:/Users/PIV/Documents/mike_ensight/NACA0015_MB_G/15ms_PLANE_B_PA_300/rear/15ms_PLANE_B_PA_300_000285.T000.D000.P007.H000.L.vec", path "C:/Users/PIV/Documents/mike_ensight/NACA0015_MB_G/15ms_PLANE_B_PA_300/rear/15ms_PLANE_B_PA_300_000286.T000.D000.P007.H000.L.vec", path "C:/Users/PIV/Documents/mike_ensight/NACA0015_MB_G/15ms_PLANE_B_PA_300/rear/15ms_PLANE_B_PA_300_000287.T000.D000.P007.H000.L.vec", path "C:/Users/PIV/Documents/mike_ensight/NACA0015_MB_G/15ms_PLANE_B_PA_300/rear/15ms_PLANE_B_PA_300_000288.T000.D000.P007.H000.L.vec", path "C:/Users/PIV/Documents/mike_ensight/NACA0015_MB_G/15ms_PLANE_B_PA_300/rear/15ms_PLANE_B_PA_300_000289.T000.D000.P007.H000.L.vec", path "C:/Users/PIV/Documents/mike_ensight/NACA0015_MB_G/15ms_PLANE_B_PA_300/rear/15ms_PLANE_B_PA_300_000290.T000.D000.P007.H000.L.vec", path "C:/Users/PIV/Documents/mike_ensight/NACA0015_MB_G/15ms_PLANE_B_PA_300/rear/15ms_PLANE_B_PA_300_000291.T000.D000.P007.H000.L.vec", path "C:/Users/PIV/Documents/mike_ensight/NACA0015_MB_G/15ms_PLANE_B_PA_300/rear/15ms_PLANE_B_PA_300_000292.T000.D000.P007.H000.L.vec", path "C:/Users/PIV/Documents/mike_ensight/NACA0015_MB_G/15ms_PLANE_B_PA_300/rear/15ms_PLANE_B_PA_300_000293.T000.D000.P007.H000.L.vec", path "C:/Users/PIV/Documents/mike_ensight/NACA0015_MB_G/15ms_PLANE_B_PA_300/rear/15ms_PLANE_B_PA_300_000294.T000.D000.P007.H000.L.vec", path "C:/Users/PIV/Documents/mike_ensight/NACA0015_MB_G/15ms_PLANE_B_PA_300/rear/15ms_PLANE_B_PA_300_000295.T000.D000.P007.H000.L.vec", path "C:/Users/PIV/Documents/mike_ensight/NACA0015_MB_G/15ms_PLANE_B_PA_300/rear/15ms_PLANE_B_PA_300_000296.T000.D000.P007.H000.L.vec", path "C:/Users/PIV/Documents/mike_ensight/NACA0015_MB_G/15ms_PLANE_B_PA_300/rear/15ms_PLANE_B_PA_300_000297.T000.D000.P007.H000.L.vec", path "C:/Users/PIV/Documents/mike_ensight/NACA0015_MB_G/15ms_PLANE_B_PA_300/rear/15ms_PLANE_B_PA_300_000298.T000.D000.P007.H000.L.vec", path "C:/Users/PIV/Documents/mike_ensight/NACA0015_MB_G/15ms_PLANE_B_PA_300/rear/15ms_PLANE_B_PA_300_000299.T000.D000.P007.H000.L.vec", path "C:/Users/PIV/Documents/mike_ensight/NACA0015_MB_G/15ms_PLANE_B_PA_300/rear/15ms_PLANE_B_PA_300_000300.T000.D000.P007.H000.L.vec", path "C:/Users/PIV/Documents/mike_ensight/NACA0015_MB_G/15ms_PLANE_B_PA_300/rear/15ms_PLANE_B_PA_300_000301.T000.D000.P007.H000.L.vec", path "C:/Users/PIV/Documents/mike_ensight/NACA0015_MB_G/15ms_PLANE_B_PA_300/rear/15ms_PLANE_B_PA_300_000302.T000.D000.P007.H000.L.vec", path "C:/Users/PIV/Documents/mike_ensight/NACA0015_MB_G/15ms_PLANE_B_PA_300/rear/15ms_PLANE_B_PA_300_000303.T000.D000.P007.H000.L.vec", path "C:/Users/PIV/Documents/mike_ensight/NACA0015_MB_G/15ms_PLANE_B_PA_300/rear/15ms_PLANE_B_PA_300_000304.T000.D000.P007.H000.L.vec", path "C:/Users/PIV/Documents/mike_ensight/NACA0015_MB_G/15ms_PLANE_B_PA_300/rear/15ms_PLANE_B_PA_300_000305.T000.D000.P007.H000.L.vec", path "C:/Users/PIV/Documents/mike_ensight/NACA0015_MB_G/15ms_PLANE_B_PA_300/rear/15ms_PLANE_B_PA_300_000306.T000.D000.P007.H000.L.vec", path "C:/Users/PIV/Documents/mike_ensight/NACA0015_MB_G/15ms_PLANE_B_PA_300/rear/15ms_PLANE_B_PA_300_000307.T000.D000.P007.H000.L.vec", path "C:/Users/PIV/Documents/mike_ensight/NACA0015_MB_G/15ms_PLANE_B_PA_300/rear/15ms_PLANE_B_PA_300_000308.T000.D000.P007.H000.L.vec", path "C:/Users/PIV/Documents/mike_ensight/NACA0015_MB_G/15ms_PLANE_B_PA_300/rear/15ms_PLANE_B_PA_300_000309.T000.D000.P007.H000.L.vec", path "C:/Users/PIV/Documents/mike_ensight/NACA0015_MB_G/15ms_PLANE_B_PA_300/rear/15ms_PLANE_B_PA_300_000310.T000.D000.P007.H000.L.vec", path "C:/Users/PIV/Documents/mike_ensight/NACA0015_MB_G/15ms_PLANE_B_PA_300/rear/15ms_PLANE_B_PA_300_000311.T000.D000.P007.H000.L.vec", path "C:/Users/PIV/Documents/mike_ensight/NACA0015_MB_G/15ms_PLANE_B_PA_300/rear/15ms_PLANE_B_PA_300_000312.T000.D000.P007.H000.L.vec", path "C:/Users/PIV/Documents/mike_ensight/NACA0015_MB_G/15ms_PLANE_B_PA_300/rear/15ms_PLANE_B_PA_300_000313.T000.D000.P007.H000.L.vec", path "C:/Users/PIV/Documents/mike_ensight/NACA0015_MB_G/15ms_PLANE_B_PA_300/rear/15ms_PLANE_B_PA_300_000314.T000.D000.P007.H000.L.vec", path "C:/Users/PIV/Documents/mike_ensight/NACA0015_MB_G/15ms_PLANE_B_PA_300/rear/15ms_PLANE_B_PA_300_000315.T000.D000.P007.H000.L.vec", path "C:/Users/PIV/Documents/mike_ensight/NACA0015_MB_G/15ms_PLANE_B_PA_300/rear/15ms_PLANE_B_PA_300_000316.T000.D000.P007.H000.L.vec", path "C:/Users/PIV/Documents/mike_ensight/NACA0015_MB_G/15ms_PLANE_B_PA_300/rear/15ms_PLANE_B_PA_300_000317.T000.D000.P007.H000.L.vec", path "C:/Users/PIV/Documents/mike_ensight/NACA0015_MB_G/15ms_PLANE_B_PA_300/rear/15ms_PLANE_B_PA_300_000318.T000.D000.P007.H000.L.vec", path "C:/Users/PIV/Documents/mike_ensight/NACA0015_MB_G/15ms_PLANE_B_PA_300/rear/15ms_PLANE_B_PA_300_000319.T000.D000.P007.H000.L.vec", path "C:/Users/PIV/Documents/mike_ensight/NACA0015_MB_G/15ms_PLANE_B_PA_300/rear/15ms_PLANE_B_PA_300_000320.T000.D000.P007.H000.L.vec", path "C:/Users/PIV/Documents/mike_ensight/NACA0015_MB_G/15ms_PLANE_B_PA_300/rear/15ms_PLANE_B_PA_300_000321.T000.D000.P007.H000.L.vec", path "C:/Users/PIV/Documents/mike_ensight/NACA0015_MB_G/15ms_PLANE_B_PA_300/rear/15ms_PLANE_B_PA_300_000322.T000.D000.P007.H000.L.vec", path "C:/Users/PIV/Documents/mike_ensight/NACA0015_MB_G/15ms_PLANE_B_PA_300/rear/15ms_PLANE_B_PA_300_000323.T000.D000.P007.H000.L.vec", path "C:/Users/PIV/Documents/mike_ensight/NACA0015_MB_G/15ms_PLANE_B_PA_300/rear/15ms_PLANE_B_PA_300_000324.T000.D000.P007.H000.L.vec", path "C:/Users/PIV/Documents/mike_ensight/NACA0015_MB_G/15ms_PLANE_B_PA_300/rear/15ms_PLANE_B_PA_300_000325.T000.D000.P007.H000.L.vec", path "C:/Users/PIV/Documents/mike_ensight/NACA0015_MB_G/15ms_PLANE_B_PA_300/rear/15ms_PLANE_B_PA_300_000326.T000.D000.P007.H000.L.vec", path "C:/Users/PIV/Documents/mike_ensight/NACA0015_MB_G/15ms_PLANE_B_PA_300/rear/15ms_PLANE_B_PA_300_000327.T000.D000.P007.H000.L.vec", path "C:/Users/PIV/Documents/mike_ensight/NACA0015_MB_G/15ms_PLANE_B_PA_300/rear/15ms_PLANE_B_PA_300_000328.T000.D000.P007.H000.L.vec", path "C:/Users/PIV/Documents/mike_ensight/NACA0015_MB_G/15ms_PLANE_B_PA_300/rear/15ms_PLANE_B_PA_300_000329.T000.D000.P007.H000.L.vec", path "C:/Users/PIV/Documents/mike_ensight/NACA0015_MB_G/15ms_PLANE_B_PA_300/rear/15ms_PLANE_B_PA_300_000330.T000.D000.P007.H000.L.vec", path "C:/Users/PIV/Documents/mike_ensight/NACA0015_MB_G/15ms_PLANE_B_PA_300/rear/15ms_PLANE_B_PA_300_000331.T000.D000.P007.H000.L.vec", path "C:/Users/PIV/Documents/mike_ensight/NACA0015_MB_G/15ms_PLANE_B_PA_300/rear/15ms_PLANE_B_PA_300_000332.T000.D000.P007.H000.L.vec", path "C:/Users/PIV/Documents/mike_ensight/NACA0015_MB_G/15ms_PLANE_B_PA_300/rear/15ms_PLANE_B_PA_300_000333.T000.D000.P007.H000.L.vec", path "C:/Users/PIV/Documents/mike_ensight/NACA0015_MB_G/15ms_PLANE_B_PA_300/rear/15ms_PLANE_B_PA_300_000334.T000.D000.P007.H000.L.vec", path "C:/Users/PIV/Documents/mike_ensight/NACA0015_MB_G/15ms_PLANE_B_PA_300/rear/15ms_PLANE_B_PA_300_000335.T000.D000.P007.H000.L.vec", path "C:/Users/PIV/Documents/mike_ensight/NACA0015_MB_G/15ms_PLANE_B_PA_300/rear/15ms_PLANE_B_PA_300_000336.T000.D000.P007.H000.L.vec", path "C:/Users/PIV/Documents/mike_ensight/NACA0015_MB_G/15ms_PLANE_B_PA_300/rear/15ms_PLANE_B_PA_300_000337.T000.D000.P007.H000.L.vec", path "C:/Users/PIV/Documents/mike_ensight/NACA0015_MB_G/15ms_PLANE_B_PA_300/rear/15ms_PLANE_B_PA_300_000338.T000.D000.P007.H000.L.vec", path "C:/Users/PIV/Documents/mike_ensight/NACA0015_MB_G/15ms_PLANE_B_PA_300/rear/15ms_PLANE_B_PA_300_000339.T000.D000.P007.H000.L.vec", path "C:/Users/PIV/Documents/mike_ensight/NACA0015_MB_G/15ms_PLANE_B_PA_300/rear/15ms_PLANE_B_PA_300_000340.T000.D000.P007.H000.L.vec", path "C:/Users/PIV/Documents/mike_ensight/NACA0015_MB_G/15ms_PLANE_B_PA_300/rear/15ms_PLANE_B_PA_300_000341.T000.D000.P007.H000.L.vec", path "C:/Users/PIV/Documents/mike_ensight/NACA0015_MB_G/15ms_PLANE_B_PA_300/rear/15ms_PLANE_B_PA_300_000342.T000.D000.P007.H000.L.vec", path "C:/Users/PIV/Documents/mike_ensight/NACA0015_MB_G/15ms_PLANE_B_PA_300/rear/15ms_PLANE_B_PA_300_000343.T000.D000.P007.H000.L.vec", path "C:/Users/PIV/Documents/mike_ensight/NACA0015_MB_G/15ms_PLANE_B_PA_300/rear/15ms_PLANE_B_PA_300_000344.T000.D000.P007.H000.L.vec", path "C:/Users/PIV/Documents/mike_ensight/NACA0015_MB_G/15ms_PLANE_B_PA_300/rear/15ms_PLANE_B_PA_300_000345.T000.D000.P007.H000.L.vec", path "C:/Users/PIV/Documents/mike_ensight/NACA0015_MB_G/15ms_PLANE_B_PA_300/rear/15ms_PLANE_B_PA_300_000346.T000.D000.P007.H000.L.vec", path "C:/Users/PIV/Documents/mike_ensight/NACA0015_MB_G/15ms_PLANE_B_PA_300/rear/15ms_PLANE_B_PA_300_000347.T000.D000.P007.H000.L.vec", path "C:/Users/PIV/Documents/mike_ensight/NACA0015_MB_G/15ms_PLANE_B_PA_300/rear/15ms_PLANE_B_PA_300_000348.T000.D000.P007.H000.L.vec", path "C:/Users/PIV/Documents/mike_ensight/NACA0015_MB_G/15ms_PLANE_B_PA_300/rear/15ms_PLANE_B_PA_300_000349.T000.D000.P007.H000.L.vec", path "C:/Users/PIV/Documents/mike_ensight/NACA0015_MB_G/15ms_PLANE_B_PA_300/rear/15ms_PLANE_B_PA_300_000350.T000.D000.P007.H000.L.vec", path "C:/Users/PIV/Documents/mike_ensight/NACA0015_MB_G/15ms_PLANE_B_PA_300/rear/15ms_PLANE_B_PA_300_000351.T000.D000.P007.H000.L.vec", path "C:/Users/PIV/Documents/mike_ensight/NACA0015_MB_G/15ms_PLANE_B_PA_300/rear/15ms_PLANE_B_PA_300_000352.T000.D000.P007.H000.L.vec", path "C:/Users/PIV/Documents/mike_ensight/NACA0015_MB_G/15ms_PLANE_B_PA_300/rear/15ms_PLANE_B_PA_300_000353.T000.D000.P007.H000.L.vec", path "C:/Users/PIV/Documents/mike_ensight/NACA0015_MB_G/15ms_PLANE_B_PA_300/rear/15ms_PLANE_B_PA_300_000354.T000.D000.P007.H000.L.vec", path "C:/Users/PIV/Documents/mike_ensight/NACA0015_MB_G/15ms_PLANE_B_PA_300/rear/15ms_PLANE_B_PA_300_000355.T000.D000.P007.H000.L.vec", path "C:/Users/PIV/Documents/mike_ensight/NACA0015_MB_G/15ms_PLANE_B_PA_300/rear/15ms_PLANE_B_PA_300_000356.T000.D000.P007.H000.L.vec", path "C:/Users/PIV/Documents/mike_ensight/NACA0015_MB_G/15ms_PLANE_B_PA_300/rear/15ms_PLANE_B_PA_300_000357.T000.D000.P007.H000.L.vec", path "C:/Users/PIV/Documents/mike_ensight/NACA0015_MB_G/15ms_PLANE_B_PA_300/rear/15ms_PLANE_B_PA_300_000358.T000.D000.P007.H000.L.vec", path "C:/Users/PIV/Documents/mike_ensight/NACA0015_MB_G/15ms_PLANE_B_PA_300/rear/15ms_PLANE_B_PA_300_000359.T000.D000.P007.H000.L.vec", path "C:/Users/PIV/Documents/mike_ensight/NACA0015_MB_G/15ms_PLANE_B_PA_300/rear/15ms_PLANE_B_PA_300_000360.T000.D000.P007.H000.L.vec", path "C:/Users/PIV/Documents/mike_ensight/NACA0015_MB_G/15ms_PLANE_B_PA_300/rear/15ms_PLANE_B_PA_300_000361.T000.D000.P007.H000.L.vec", path "C:/Users/PIV/Documents/mike_ensight/NACA0015_MB_G/15ms_PLANE_B_PA_300/rear/15ms_PLANE_B_PA_300_000362.T000.D000.P007.H000.L.vec", path "C:/Users/PIV/Documents/mike_ensight/NACA0015_MB_G/15ms_PLANE_B_PA_300/rear/15ms_PLANE_B_PA_300_000363.T000.D000.P007.H000.L.vec", path "C:/Users/PIV/Documents/mike_ensight/NACA0015_MB_G/15ms_PLANE_B_PA_300/rear/15ms_PLANE_B_PA_300_000364.T000.D000.P007.H000.L.vec", path "C:/Users/PIV/Documents/mike_ensight/NACA0015_MB_G/15ms_PLANE_B_PA_300/rear/15ms_PLANE_B_PA_300_000365.T000.D000.P007.H000.L.vec", path "C:/Users/PIV/Documents/mike_ensight/NACA0015_MB_G/15ms_PLANE_B_PA_300/rear/15ms_PLANE_B_PA_300_000366.T000.D000.P007.H000.L.vec", path "C:/Users/PIV/Documents/mike_ensight/NACA0015_MB_G/15ms_PLANE_B_PA_300/rear/15ms_PLANE_B_PA_300_000367.T000.D000.P007.H000.L.vec", path "C:/Users/PIV/Documents/mike_ensight/NACA0015_MB_G/15ms_PLANE_B_PA_300/rear/15ms_PLANE_B_PA_300_000368.T000.D000.P007.H000.L.vec", path "C:/Users/PIV/Documents/mike_ensight/NACA0015_MB_G/15ms_PLANE_B_PA_300/rear/15ms_PLANE_B_PA_300_000369.T000.D000.P007.H000.L.vec", path "C:/Users/PIV/Documents/mike_ensight/NACA0015_MB_G/15ms_PLANE_B_PA_300/rear/15ms_PLANE_B_PA_300_000370.T000.D000.P007.H000.L.vec", path "C:/Users/PIV/Documents/mike_ensight/NACA0015_MB_G/15ms_PLANE_B_PA_300/rear/15ms_PLANE_B_PA_300_000371.T000.D000.P007.H000.L.vec", path "C:/Users/PIV/Documents/mike_ensight/NACA0015_MB_G/15ms_PLANE_B_PA_300/rear/15ms_PLANE_B_PA_300_000372.T000.D000.P007.H000.L.vec", path "C:/Users/PIV/Documents/mike_ensight/NACA0015_MB_G/15ms_PLANE_B_PA_300/rear/15ms_PLANE_B_PA_300_000373.T000.D000.P007.H000.L.vec", path "C:/Users/PIV/Documents/mike_ensight/NACA0015_MB_G/15ms_PLANE_B_PA_300/rear/15ms_PLANE_B_PA_300_000374.T000.D000.P007.H000.L.vec", path "C:/Users/PIV/Documents/mike_ensight/NACA0015_MB_G/15ms_PLANE_B_PA_300/rear/15ms_PLANE_B_PA_300_000375.T000.D000.P007.H000.L.vec", path "C:/Users/PIV/Documents/mike_ensight/NACA0015_MB_G/15ms_PLANE_B_PA_300/rear/15ms_PLANE_B_PA_300_000376.T000.D000.P007.H000.L.vec", path "C:/Users/PIV/Documents/mike_ensight/NACA0015_MB_G/15ms_PLANE_B_PA_300/rear/15ms_PLANE_B_PA_300_000377.T000.D000.P007.H000.L.vec", path "C:/Users/PIV/Documents/mike_ensight/NACA0015_MB_G/15ms_PLANE_B_PA_300/rear/15ms_PLANE_B_PA_300_000378.T000.D000.P007.H000.L.vec", path "C:/Users/PIV/Documents/mike_ensight/NACA0015_MB_G/15ms_PLANE_B_PA_300/rear/15ms_PLANE_B_PA_300_000379.T000.D000.P007.H000.L.vec", path "C:/Users/PIV/Documents/mike_ensight/NACA0015_MB_G/15ms_PLANE_B_PA_300/rear/15ms_PLANE_B_PA_300_000380.T000.D000.P007.H000.L.vec", path "C:/Users/PIV/Documents/mike_ensight/NACA0015_MB_G/15ms_PLANE_B_PA_300/rear/15ms_PLANE_B_PA_300_000381.T000.D000.P007.H000.L.vec", path "C:/Users/PIV/Documents/mike_ensight/NACA0015_MB_G/15ms_PLANE_B_PA_300/rear/15ms_PLANE_B_PA_300_000382.T000.D000.P007.H000.L.vec", path "C:/Users/PIV/Documents/mike_ensight/NACA0015_MB_G/15ms_PLANE_B_PA_300/rear/15ms_PLANE_B_PA_300_000383.T000.D000.P007.H000.L.vec", path "C:/Users/PIV/Documents/mike_ensight/NACA0015_MB_G/15ms_PLANE_B_PA_300/rear/15ms_PLANE_B_PA_300_000384.T000.D000.P007.H000.L.vec", path "C:/Users/PIV/Documents/mike_ensight/NACA0015_MB_G/15ms_PLANE_B_PA_300/rear/15ms_PLANE_B_PA_300_000385.T000.D000.P007.H000.L.vec", path "C:/Users/PIV/Documents/mike_ensight/NACA0015_MB_G/15ms_PLANE_B_PA_300/rear/15ms_PLANE_B_PA_300_000386.T000.D000.P007.H000.L.vec", path "C:/Users/PIV/Documents/mike_ensight/NACA0015_MB_G/15ms_PLANE_B_PA_300/rear/15ms_PLANE_B_PA_300_000387.T000.D000.P007.H000.L.vec", path "C:/Users/PIV/Documents/mike_ensight/NACA0015_MB_G/15ms_PLANE_B_PA_300/rear/15ms_PLANE_B_PA_300_000388.T000.D000.P007.H000.L.vec", path "C:/Users/PIV/Documents/mike_ensight/NACA0015_MB_G/15ms_PLANE_B_PA_300/rear/15ms_PLANE_B_PA_300_000389.T000.D000.P007.H000.L.vec", path "C:/Users/PIV/Documents/mike_ensight/NACA0015_MB_G/15ms_PLANE_B_PA_300/rear/15ms_PLANE_B_PA_300_000390.T000.D000.P007.H000.L.vec", path "C:/Users/PIV/Documents/mike_ensight/NACA0015_MB_G/15ms_PLANE_B_PA_300/rear/15ms_PLANE_B_PA_300_000391.T000.D000.P007.H000.L.vec", path "C:/Users/PIV/Documents/mike_ensight/NACA0015_MB_G/15ms_PLANE_B_PA_300/rear/15ms_PLANE_B_PA_300_000392.T000.D000.P007.H000.L.vec", path "C:/Users/PIV/Documents/mike_ensight/NACA0015_MB_G/15ms_PLANE_B_PA_300/rear/15ms_PLANE_B_PA_300_000393.T000.D000.P007.H000.L.vec", path "C:/Users/PIV/Documents/mike_ensight/NACA0015_MB_G/15ms_PLANE_B_PA_300/rear/15ms_PLANE_B_PA_300_000394.T000.D000.P007.H000.L.vec", path "C:/Users/PIV/Documents/mike_ensight/NACA0015_MB_G/15ms_PLANE_B_PA_300/rear/15ms_PLANE_B_PA_300_000395.T000.D000.P007.H000.L.vec", path "C:/Users/PIV/Documents/mike_ensight/NACA0015_MB_G/15ms_PLANE_B_PA_300/rear/15ms_PLANE_B_PA_300_000396.T000.D000.P007.H000.L.vec", path "C:/Users/PIV/Documents/mike_ensight/NACA0015_MB_G/15ms_PLANE_B_PA_300/rear/15ms_PLANE_B_PA_300_000397.T000.D000.P007.H000.L.vec", path "C:/Users/PIV/Documents/mike_ensight/NACA0015_MB_G/15ms_PLANE_B_PA_300/rear/15ms_PLANE_B_PA_300_000398.T000.D000.P007.H000.L.vec", path "C:/Users/PIV/Documents/mike_ensight/NACA0015_MB_G/15ms_PLANE_B_PA_300/rear/15ms_PLANE_B_PA_300_000399.T000.D000.P007.H000.L.vec", path "C:/Users/PIV/Documents/mike_ensight/NACA0015_MB_G/15ms_PLANE_B_PA_300/rear/15ms_PLANE_B_PA_300_000400.T000.D000.P007.H000.L.vec", path "C:/Users/PIV/Documents/mike_ensight/NACA0015_MB_G/15ms_PLANE_B_PA_300/rear/15ms_PLANE_B_PA_300_000401.T000.D000.P007.H000.L.vec", path "C:/Users/PIV/Documents/mike_ensight/NACA0015_MB_G/15ms_PLANE_B_PA_300/rear/15ms_PLANE_B_PA_300_000402.T000.D000.P007.H000.L.vec", path "C:/Users/PIV/Documents/mike_ensight/NACA0015_MB_G/15ms_PLANE_B_PA_300/rear/15ms_PLANE_B_PA_300_000403.T000.D000.P007.H000.L.vec", path "C:/Users/PIV/Documents/mike_ensight/NACA0015_MB_G/15ms_PLANE_B_PA_300/rear/15ms_PLANE_B_PA_300_000404.T000.D000.P007.H000.L.vec", path "C:/Users/PIV/Documents/mike_ensight/NACA0015_MB_G/15ms_PLANE_B_PA_300/rear/15ms_PLANE_B_PA_300_000405.T000.D000.P007.H000.L.vec", path "C:/Users/PIV/Documents/mike_ensight/NACA0015_MB_G/15ms_PLANE_B_PA_300/rear/15ms_PLANE_B_PA_300_000406.T000.D000.P007.H000.L.vec", path "C:/Users/PIV/Documents/mike_ensight/NACA0015_MB_G/15ms_PLANE_B_PA_300/rear/15ms_PLANE_B_PA_300_000407.T000.D000.P007.H000.L.vec", path "C:/Users/PIV/Documents/mike_ensight/NACA0015_MB_G/15ms_PLANE_B_PA_300/rear/15ms_PLANE_B_PA_300_000408.T000.D000.P007.H000.L.vec", path "C:/Users/PIV/Documents/mike_ensight/NACA0015_MB_G/15ms_PLANE_B_PA_300/rear/15ms_PLANE_B_PA_300_000409.T000.D000.P007.H000.L.vec", path "C:/Users/PIV/Documents/mike_ensight/NACA0015_MB_G/15ms_PLANE_B_PA_300/rear/15ms_PLANE_B_PA_300_000410.T000.D000.P007.H000.L.vec", path "C:/Users/PIV/Documents/mike_ensight/NACA0015_MB_G/15ms_PLANE_B_PA_300/rear/15ms_PLANE_B_PA_300_000411.T000.D000.P007.H000.L.vec", path "C:/Users/PIV/Documents/mike_ensight/NACA0015_MB_G/15ms_PLANE_B_PA_300/rear/15ms_PLANE_B_PA_300_000412.T000.D000.P007.H000.L.vec", path "C:/Users/PIV/Documents/mike_ensight/NACA0015_MB_G/15ms_PLANE_B_PA_300/rear/15ms_PLANE_B_PA_300_000413.T000.D000.P007.H000.L.vec", path "C:/Users/PIV/Documents/mike_ensight/NACA0015_MB_G/15ms_PLANE_B_PA_300/rear/15ms_PLANE_B_PA_300_000414.T000.D000.P007.H000.L.vec", path "C:/Users/PIV/Documents/mike_ensight/NACA0015_MB_G/15ms_PLANE_B_PA_300/rear/15ms_PLANE_B_PA_300_000415.T000.D000.P007.H000.L.vec", path "C:/Users/PIV/Documents/mike_ensight/NACA0015_MB_G/15ms_PLANE_B_PA_300/rear/15ms_PLANE_B_PA_300_000416.T000.D000.P007.H000.L.vec", path "C:/Users/PIV/Documents/mike_ensight/NACA0015_MB_G/15ms_PLANE_B_PA_300/rear/15ms_PLANE_B_PA_300_000417.T000.D000.P007.H000.L.vec", path "C:/Users/PIV/Documents/mike_ensight/NACA0015_MB_G/15ms_PLANE_B_PA_300/rear/15ms_PLANE_B_PA_300_000418.T000.D000.P007.H000.L.vec", path "C:/Users/PIV/Documents/mike_ensight/NACA0015_MB_G/15ms_PLANE_B_PA_300/rear/15ms_PLANE_B_PA_300_000419.T000.D000.P007.H000.L.vec", path "C:/Users/PIV/Documents/mike_ensight/NACA0015_MB_G/15ms_PLANE_B_PA_300/rear/15ms_PLANE_B_PA_300_000420.T000.D000.P007.H000.L.vec", path "C:/Users/PIV/Documents/mike_ensight/NACA0015_MB_G/15ms_PLANE_B_PA_300/rear/15ms_PLANE_B_PA_300_000421.T000.D000.P007.H000.L.vec", path "C:/Users/PIV/Documents/mike_ensight/NACA0015_MB_G/15ms_PLANE_B_PA_300/rear/15ms_PLANE_B_PA_300_000422.T000.D000.P007.H000.L.vec", path "C:/Users/PIV/Documents/mike_ensight/NACA0015_MB_G/15ms_PLANE_B_PA_300/rear/15ms_PLANE_B_PA_300_000423.T000.D000.P007.H000.L.vec", path "C:/Users/PIV/Documents/mike_ensight/NACA0015_MB_G/15ms_PLANE_B_PA_300/rear/15ms_PLANE_B_PA_300_000424.T000.D000.P007.H000.L.vec", path "C:/Users/PIV/Documents/mike_ensight/NACA0015_MB_G/15ms_PLANE_B_PA_300/rear/15ms_PLANE_B_PA_300_000425.T000.D000.P007.H000.L.vec", path "C:/Users/PIV/Documents/mike_ensight/NACA0015_MB_G/15ms_PLANE_B_PA_300/rear/15ms_PLANE_B_PA_300_000426.T000.D000.P007.H000.L.vec", path "C:/Users/PIV/Documents/mike_ensight/NACA0015_MB_G/15ms_PLANE_B_PA_300/rear/15ms_PLANE_B_PA_300_000427.T000.D000.P007.H000.L.vec", path "C:/Users/PIV/Documents/mike_ensight/NACA0015_MB_G/15ms_PLANE_B_PA_300/rear/15ms_PLANE_B_PA_300_000428.T000.D000.P007.H000.L.vec", path "C:/Users/PIV/Documents/mike_ensight/NACA0015_MB_G/15ms_PLANE_B_PA_300/rear/15ms_PLANE_B_PA_300_000429.T000.D000.P007.H000.L.vec", path "C:/Users/PIV/Documents/mike_ensight/NACA0015_MB_G/15ms_PLANE_B_PA_300/rear/15ms_PLANE_B_PA_300_000430.T000.D000.P007.H000.L.vec", path "C:/Users/PIV/Documents/mike_ensight/NACA0015_MB_G/15ms_PLANE_B_PA_300/rear/15ms_PLANE_B_PA_300_000431.T000.D000.P007.H000.L.vec", path "C:/Users/PIV/Documents/mike_ensight/NACA0015_MB_G/15ms_PLANE_B_PA_300/rear/15ms_PLANE_B_PA_300_000432.T000.D000.P007.H000.L.vec", path "C:/Users/PIV/Documents/mike_ensight/NACA0015_MB_G/15ms_PLANE_B_PA_300/rear/15ms_PLANE_B_PA_300_000433.T000.D000.P007.H000.L.vec", path "C:/Users/PIV/Documents/mike_ensight/NACA0015_MB_G/15ms_PLANE_B_PA_300/rear/15ms_PLANE_B_PA_300_000434.T000.D000.P007.H000.L.vec", path "C:/Users/PIV/Documents/mike_ensight/NACA0015_MB_G/15ms_PLANE_B_PA_300/rear/15ms_PLANE_B_PA_300_000435.T000.D000.P007.H000.L.vec", path "C:/Users/PIV/Documents/mike_ensight/NACA0015_MB_G/15ms_PLANE_B_PA_300/rear/15ms_PLANE_B_PA_300_000436.T000.D000.P007.H000.L.vec", path "C:/Users/PIV/Documents/mike_ensight/NACA0015_MB_G/15ms_PLANE_B_PA_300/rear/15ms_PLANE_B_PA_300_000437.T000.D000.P007.H000.L.vec", path "C:/Users/PIV/Documents/mike_ensight/NACA0015_MB_G/15ms_PLANE_B_PA_300/rear/15ms_PLANE_B_PA_300_000438.T000.D000.P007.H000.L.vec", path "C:/Users/PIV/Documents/mike_ensight/NACA0015_MB_G/15ms_PLANE_B_PA_300/rear/15ms_PLANE_B_PA_300_000439.T000.D000.P007.H000.L.vec", path "C:/Users/PIV/Documents/mike_ensight/NACA0015_MB_G/15ms_PLANE_B_PA_300/rear/15ms_PLANE_B_PA_300_000440.T000.D000.P007.H000.L.vec", path "C:/Users/PIV/Documents/mike_ensight/NACA0015_MB_G/15ms_PLANE_B_PA_300/rear/15ms_PLANE_B_PA_300_000441.T000.D000.P007.H000.L.vec", path "C:/Users/PIV/Documents/mike_ensight/NACA0015_MB_G/15ms_PLANE_B_PA_300/rear/15ms_PLANE_B_PA_300_000442.T000.D000.P007.H000.L.vec", path "C:/Users/PIV/Documents/mike_ensight/NACA0015_MB_G/15ms_PLANE_B_PA_300/rear/15ms_PLANE_B_PA_300_000443.T000.D000.P007.H000.L.vec", path "C:/Users/PIV/Documents/mike_ensight/NACA0015_MB_G/15ms_PLANE_B_PA_300/rear/15ms_PLANE_B_PA_300_000444.T000.D000.P007.H000.L.vec", path "C:/Users/PIV/Documents/mike_ensight/NACA0015_MB_G/15ms_PLANE_B_PA_300/rear/15ms_PLANE_B_PA_300_000445.T000.D000.P007.H000.L.vec", path "C:/Users/PIV/Documents/mike_ensight/NACA0015_MB_G/15ms_PLANE_B_PA_300/rear/15ms_PLANE_B_PA_300_000446.T000.D000.P007.H000.L.vec", path "C:/Users/PIV/Documents/mike_ensight/NACA0015_MB_G/15ms_PLANE_B_PA_300/rear/15ms_PLANE_B_PA_300_000447.T000.D000.P007.H000.L.vec", path "C:/Users/PIV/Documents/mike_ensight/NACA0015_MB_G/15ms_PLANE_B_PA_300/rear/15ms_PLANE_B_PA_300_000448.T000.D000.P007.H000.L.vec", path "C:/Users/PIV/Documents/mike_ensight/NACA0015_MB_G/15ms_PLANE_B_PA_300/rear/15ms_PLANE_B_PA_300_000449.T000.D000.P007.H000.L.vec", path "C:/Users/PIV/Documents/mike_ensight/NACA0015_MB_G/15ms_PLANE_B_PA_300/rear/15ms_PLANE_B_PA_300_000450.T000.D000.P007.H000.L.vec", path "C:/Users/PIV/Documents/mike_ensight/NACA0015_MB_G/15ms_PLANE_B_PA_300/rear/15ms_PLANE_B_PA_300_000451.T000.D000.P007.H000.L.vec", path "C:/Users/PIV/Documents/mike_ensight/NACA0015_MB_G/15ms_PLANE_B_PA_300/rear/15ms_PLANE_B_PA_300_000452.T000.D000.P007.H000.L.vec", path "C:/Users/PIV/Documents/mike_ensight/NACA0015_MB_G/15ms_PLANE_B_PA_300/rear/15ms_PLANE_B_PA_300_000453.T000.D000.P007.H000.L.vec", path "C:/Users/PIV/Documents/mike_ensight/NACA0015_MB_G/15ms_PLANE_B_PA_300/rear/15ms_PLANE_B_PA_300_000454.T000.D000.P007.H000.L.vec", path "C:/Users/PIV/Documents/mike_ensight/NACA0015_MB_G/15ms_PLANE_B_PA_300/rear/15ms_PLANE_B_PA_300_000455.T000.D000.P007.H000.L.vec", path "C:/Users/PIV/Documents/mike_ensight/NACA0015_MB_G/15ms_PLANE_B_PA_300/rear/15ms_PLANE_B_PA_300_000456.T000.D000.P007.H000.L.vec", path "C:/Users/PIV/Documents/mike_ensight/NACA0015_MB_G/15ms_PLANE_B_PA_300/rear/15ms_PLANE_B_PA_300_000457.T000.D000.P007.H000.L.vec", path "C:/Users/PIV/Documents/mike_ensight/NACA0015_MB_G/15ms_PLANE_B_PA_300/rear/15ms_PLANE_B_PA_300_000458.T000.D000.P007.H000.L.vec", path "C:/Users/PIV/Documents/mike_ensight/NACA0015_MB_G/15ms_PLANE_B_PA_300/rear/15ms_PLANE_B_PA_300_000459.T000.D000.P007.H000.L.vec", path "C:/Users/PIV/Documents/mike_ensight/NACA0015_MB_G/15ms_PLANE_B_PA_300/rear/15ms_PLANE_B_PA_300_000460.T000.D000.P007.H000.L.vec", path "C:/Users/PIV/Documents/mike_ensight/NACA0015_MB_G/15ms_PLANE_B_PA_300/rear/15ms_PLANE_B_PA_300_000461.T000.D000.P007.H000.L.vec", path "C:/Users/PIV/Documents/mike_ensight/NACA0015_MB_G/15ms_PLANE_B_PA_300/rear/15ms_PLANE_B_PA_300_000462.T000.D000.P007.H000.L.vec", path "C:/Users/PIV/Documents/mike_ensight/NACA0015_MB_G/15ms_PLANE_B_PA_300/rear/15ms_PLANE_B_PA_300_000463.T000.D000.P007.H000.L.vec", path "C:/Users/PIV/Documents/mike_ensight/NACA0015_MB_G/15ms_PLANE_B_PA_300/rear/15ms_PLANE_B_PA_300_000464.T000.D000.P007.H000.L.vec", path "C:/Users/PIV/Documents/mike_ensight/NACA0015_MB_G/15ms_PLANE_B_PA_300/rear/15ms_PLANE_B_PA_300_000465.T000.D000.P007.H000.L.vec", path "C:/Users/PIV/Documents/mike_ensight/NACA0015_MB_G/15ms_PLANE_B_PA_300/rear/15ms_PLANE_B_PA_300_000466.T000.D000.P007.H000.L.vec", path "C:/Users/PIV/Documents/mike_ensight/NACA0015_MB_G/15ms_PLANE_B_PA_300/rear/15ms_PLANE_B_PA_300_000467.T000.D000.P007.H000.L.vec", path "C:/Users/PIV/Documents/mike_ensight/NACA0015_MB_G/15ms_PLANE_B_PA_300/rear/15ms_PLANE_B_PA_300_000468.T000.D000.P007.H000.L.vec", path "C:/Users/PIV/Documents/mike_ensight/NACA0015_MB_G/15ms_PLANE_B_PA_300/rear/15ms_PLANE_B_PA_300_000469.T000.D000.P007.H000.L.vec", path "C:/Users/PIV/Documents/mike_ensight/NACA0015_MB_G/15ms_PLANE_B_PA_300/rear/15ms_PLANE_B_PA_300_000470.T000.D000.P007.H000.L.vec", path "C:/Users/PIV/Documents/mike_ensight/NACA0015_MB_G/15ms_PLANE_B_PA_300/rear/15ms_PLANE_B_PA_300_000471.T000.D000.P007.H000.L.vec", path "C:/Users/PIV/Documents/mike_ensight/NACA0015_MB_G/15ms_PLANE_B_PA_300/rear/15ms_PLANE_B_PA_300_000472.T000.D000.P007.H000.L.vec", path "C:/Users/PIV/Documents/mike_ensight/NACA0015_MB_G/15ms_PLANE_B_PA_300/rear/15ms_PLANE_B_PA_300_000473.T000.D000.P007.H000.L.vec", path "C:/Users/PIV/Documents/mike_ensight/NACA0015_MB_G/15ms_PLANE_B_PA_300/rear/15ms_PLANE_B_PA_300_000474.T000.D000.P007.H000.L.vec", path "C:/Users/PIV/Documents/mike_ensight/NACA0015_MB_G/15ms_PLANE_B_PA_300/rear/15ms_PLANE_B_PA_300_000475.T000.D000.P007.H000.L.vec", path "C:/Users/PIV/Documents/mike_ensight/NACA0015_MB_G/15ms_PLANE_B_PA_300/rear/15ms_PLANE_B_PA_300_000476.T000.D000.P007.H000.L.vec", path "C:/Users/PIV/Documents/mike_ensight/NACA0015_MB_G/15ms_PLANE_B_PA_300/rear/15ms_PLANE_B_PA_300_000477.T000.D000.P007.H000.L.vec", path "C:/Users/PIV/Documents/mike_ensight/NACA0015_MB_G/15ms_PLANE_B_PA_300/rear/15ms_PLANE_B_PA_300_000478.T000.D000.P007.H000.L.vec", path "C:/Users/PIV/Documents/mike_ensight/NACA0015_MB_G/15ms_PLANE_B_PA_300/rear/15ms_PLANE_B_PA_300_000479.T000.D000.P007.H000.L.vec", path "C:/Users/PIV/Documents/mike_ensight/NACA0015_MB_G/15ms_PLANE_B_PA_300/rear/15ms_PLANE_B_PA_300_000480.T000.D000.P007.H000.L.vec", path "C:/Users/PIV/Documents/mike_ensight/NACA0015_MB_G/15ms_PLANE_B_PA_300/rear/15ms_PLANE_B_PA_300_000481.T000.D000.P007.H000.L.vec", path "C:/Users/PIV/Documents/mike_ensight/NACA0015_MB_G/15ms_PLANE_B_PA_300/rear/15ms_PLANE_B_PA_300_000482.T000.D000.P007.H000.L.vec", path "C:/Users/PIV/Documents/mike_ensight/NACA0015_MB_G/15ms_PLANE_B_PA_300/rear/15ms_PLANE_B_PA_300_000483.T000.D000.P007.H000.L.vec", path "C:/Users/PIV/Documents/mike_ensight/NACA0015_MB_G/15ms_PLANE_B_PA_300/rear/15ms_PLANE_B_PA_300_000484.T000.D000.P007.H000.L.vec", path "C:/Users/PIV/Documents/mike_ensight/NACA0015_MB_G/15ms_PLANE_B_PA_300/rear/15ms_PLANE_B_PA_300_000485.T000.D000.P007.H000.L.vec", path "C:/Users/PIV/Documents/mike_ensight/NACA0015_MB_G/15ms_PLANE_B_PA_300/rear/15ms_PLANE_B_PA_300_000486.T000.D000.P007.H000.L.vec", path "C:/Users/PIV/Documents/mike_ensight/NACA0015_MB_G/15ms_PLANE_B_PA_300/rear/15ms_PLANE_B_PA_300_000487.T000.D000.P007.H000.L.vec", path "C:/Users/PIV/Documents/mike_ensight/NACA0015_MB_G/15ms_PLANE_B_PA_300/rear/15ms_PLANE_B_PA_300_000488.T000.D000.P007.H000.L.vec", path "C:/Users/PIV/Documents/mike_ensight/NACA0015_MB_G/15ms_PLANE_B_PA_300/rear/15ms_PLANE_B_PA_300_000489.T000.D000.P007.H000.L.vec", path "C:/Users/PIV/Documents/mike_ensight/NACA0015_MB_G/15ms_PLANE_B_PA_300/rear/15ms_PLANE_B_PA_300_000490.T000.D000.P007.H000.L.vec", path "C:/Users/PIV/Documents/mike_ensight/NACA0015_MB_G/15ms_PLANE_B_PA_300/rear/15ms_PLANE_B_PA_300_000491.T000.D000.P007.H000.L.vec", path "C:/Users/PIV/Documents/mike_ensight/NACA0015_MB_G/15ms_PLANE_B_PA_300/rear/15ms_PLANE_B_PA_300_000492.T000.D000.P007.H000.L.vec", path "C:/Users/PIV/Documents/mike_ensight/NACA0015_MB_G/15ms_PLANE_B_PA_300/rear/15ms_PLANE_B_PA_300_000493.T000.D000.P007.H000.L.vec", path "C:/Users/PIV/Documents/mike_ensight/NACA0015_MB_G/15ms_PLANE_B_PA_300/rear/15ms_PLANE_B_PA_300_000494.T000.D000.P007.H000.L.vec", path "C:/Users/PIV/Documents/mike_ensight/NACA0015_MB_G/15ms_PLANE_B_PA_300/rear/15ms_PLANE_B_PA_300_000495.T000.D000.P007.H000.L.vec", path "C:/Users/PIV/Documents/mike_ensight/NACA0015_MB_G/15ms_PLANE_B_PA_300/rear/15ms_PLANE_B_PA_300_000496.T000.D000.P007.H000.L.vec", path "C:/Users/PIV/Documents/mike_ensight/NACA0015_MB_G/15ms_PLANE_B_PA_300/rear/15ms_PLANE_B_PA_300_000497.T000.D000.P007.H000.L.vec", path "C:/Users/PIV/Documents/mike_ensight/NACA0015_MB_G/15ms_PLANE_B_PA_300/rear/15ms_PLANE_B_PA_300_000498.T000.D000.P007.H000.L.vec", path "C:/Users/PIV/Documents/mike_ensight/NACA0015_MB_G/15ms_PLANE_B_PA_300/rear/15ms_PLANE_B_PA_300_000499.T000.D000.P007.H000.L.vec", path "C:/Users/PIV/Documents/mike_ensight/NACA0015_MB_G/15ms_PLANE_B_PA_300/rear/15ms_PLANE_B_PA_300_000500.T000.D000.P007.H000.L.vec", path "C:/Users/PIV/Documents/mike_ensight/NACA0015_MB_G/15ms_PLANE_B_PA_300/rear/15ms_PLANE_B_PA_300_000501.T000.D000.P007.H000.L.vec", path "C:/Users/PIV/Documents/mike_ensight/NACA0015_MB_G/15ms_PLANE_B_PA_300/rear/15ms_PLANE_B_PA_300_000502.T000.D000.P007.H000.L.vec", path "C:/Users/PIV/Documents/mike_ensight/NACA0015_MB_G/15ms_PLANE_B_PA_300/rear/15ms_PLANE_B_PA_300_000503.T000.D000.P007.H000.L.vec", path "C:/Users/PIV/Documents/mike_ensight/NACA0015_MB_G/15ms_PLANE_B_PA_300/rear/15ms_PLANE_B_PA_300_000504.T000.D000.P007.H000.L.vec", path "C:/Users/PIV/Documents/mike_ensight/NACA0015_MB_G/15ms_PLANE_B_PA_300/rear/15ms_PLANE_B_PA_300_000505.T000.D000.P007.H000.L.vec", path "C:/Users/PIV/Documents/mike_ensight/NACA0015_MB_G/15ms_PLANE_B_PA_300/rear/15ms_PLANE_B_PA_300_000506.T000.D000.P007.H000.L.vec", path "C:/Users/PIV/Documents/mike_ensight/NACA0015_MB_G/15ms_PLANE_B_PA_300/rear/15ms_PLANE_B_PA_300_000507.T000.D000.P007.H000.L.vec", path "C:/Users/PIV/Documents/mike_ensight/NACA0015_MB_G/15ms_PLANE_B_PA_300/rear/15ms_PLANE_B_PA_300_000508.T000.D000.P007.H000.L.vec", path "C:/Users/PIV/Documents/mike_ensight/NACA0015_MB_G/15ms_PLANE_B_PA_300/rear/15ms_PLANE_B_PA_300_000509.T000.D000.P007.H000.L.vec", path "C:/Users/PIV/Documents/mike_ensight/NACA0015_MB_G/15ms_PLANE_B_PA_300/rear/15ms_PLANE_B_PA_300_000510.T000.D000.P007.H000.L.vec", path "C:/Users/PIV/Documents/mike_ensight/NACA0015_MB_G/15ms_PLANE_B_PA_300/rear/15ms_PLANE_B_PA_300_000511.T000.D000.P007.H000.L.vec", path "C:/Users/PIV/Documents/mike_ensight/NACA0015_MB_G/15ms_PLANE_B_PA_300/rear/15ms_PLANE_B_PA_300_000512.T000.D000.P007.H000.L.vec", path "C:/Users/PIV/Documents/mike_ensight/NACA0015_MB_G/15ms_PLANE_B_PA_300/rear/15ms_PLANE_B_PA_300_000513.T000.D000.P007.H000.L.vec", path "C:/Users/PIV/Documents/mike_ensight/NACA0015_MB_G/15ms_PLANE_B_PA_300/rear/15ms_PLANE_B_PA_300_000514.T000.D000.P007.H000.L.vec", path "C:/Users/PIV/Documents/mike_ensight/NACA0015_MB_G/15ms_PLANE_B_PA_300/rear/15ms_PLANE_B_PA_300_000515.T000.D000.P007.H000.L.vec", path "C:/Users/PIV/Documents/mike_ensight/NACA0015_MB_G/15ms_PLANE_B_PA_300/rear/15ms_PLANE_B_PA_300_000516.T000.D000.P007.H000.L.vec", path "C:/Users/PIV/Documents/mike_ensight/NACA0015_MB_G/15ms_PLANE_B_PA_300/rear/15ms_PLANE_B_PA_300_000517.T000.D000.P007.H000.L.vec", path "C:/Users/PIV/Documents/mike_ensight/NACA0015_MB_G/15ms_PLANE_B_PA_300/rear/15ms_PLANE_B_PA_300_000518.T000.D000.P007.H000.L.vec", path "C:/Users/PIV/Documents/mike_ensight/NACA0015_MB_G/15ms_PLANE_B_PA_300/rear/15ms_PLANE_B_PA_300_000519.T000.D000.P007.H000.L.vec", path "C:/Users/PIV/Documents/mike_ensight/NACA0015_MB_G/15ms_PLANE_B_PA_300/rear/15ms_PLANE_B_PA_300_000520.T000.D000.P007.H000.L.vec", path "C:/Users/PIV/Documents/mike_ensight/NACA0015_MB_G/15ms_PLANE_B_PA_300/rear/15ms_PLANE_B_PA_300_000521.T000.D000.P007.H000.L.vec", path "C:/Users/PIV/Documents/mike_ensight/NACA0015_MB_G/15ms_PLANE_B_PA_300/rear/15ms_PLANE_B_PA_300_000522.T000.D000.P007.H000.L.vec", path "C:/Users/PIV/Documents/mike_ensight/NACA0015_MB_G/15ms_PLANE_B_PA_300/rear/15ms_PLANE_B_PA_300_000523.T000.D000.P007.H000.L.vec", path "C:/Users/PIV/Documents/mike_ensight/NACA0015_MB_G/15ms_PLANE_B_PA_300/rear/15ms_PLANE_B_PA_300_000524.T000.D000.P007.H000.L.vec", path "C:/Users/PIV/Documents/mike_ensight/NACA0015_MB_G/15ms_PLANE_B_PA_300/rear/15ms_PLANE_B_PA_300_000525.T000.D000.P007.H000.L.vec", path "C:/Users/PIV/Documents/mike_ensight/NACA0015_MB_G/15ms_PLANE_B_PA_300/rear/15ms_PLANE_B_PA_300_000526.T000.D000.P007.H000.L.vec", path "C:/Users/PIV/Documents/mike_ensight/NACA0015_MB_G/15ms_PLANE_B_PA_300/rear/15ms_PLANE_B_PA_300_000527.T000.D000.P007.H000.L.vec", path "C:/Users/PIV/Documents/mike_ensight/NACA0015_MB_G/15ms_PLANE_B_PA_300/rear/15ms_PLANE_B_PA_300_000528.T000.D000.P007.H000.L.vec", path "C:/Users/PIV/Documents/mike_ensight/NACA0015_MB_G/15ms_PLANE_B_PA_300/rear/15ms_PLANE_B_PA_300_000529.T000.D000.P007.H000.L.vec", path "C:/Users/PIV/Documents/mike_ensight/NACA0015_MB_G/15ms_PLANE_B_PA_300/rear/15ms_PLANE_B_PA_300_000530.T000.D000.P007.H000.L.vec", path "C:/Users/PIV/Documents/mike_ensight/NACA0015_MB_G/15ms_PLANE_B_PA_300/rear/15ms_PLANE_B_PA_300_000531.T000.D000.P007.H000.L.vec", path "C:/Users/PIV/Documents/mike_ensight/NACA0015_MB_G/15ms_PLANE_B_PA_300/rear/15ms_PLANE_B_PA_300_000532.T000.D000.P007.H000.L.vec", path "C:/Users/PIV/Documents/mike_ensight/NACA0015_MB_G/15ms_PLANE_B_PA_300/rear/15ms_PLANE_B_PA_300_000533.T000.D000.P007.H000.L.vec", path "C:/Users/PIV/Documents/mike_ensight/NACA0015_MB_G/15ms_PLANE_B_PA_300/rear/15ms_PLANE_B_PA_300_000534.T000.D000.P007.H000.L.vec", path "C:/Users/PIV/Documents/mike_ensight/NACA0015_MB_G/15ms_PLANE_B_PA_300/rear/15ms_PLANE_B_PA_300_000535.T000.D000.P007.H000.L.vec", path "C:/Users/PIV/Documents/mike_ensight/NACA0015_MB_G/15ms_PLANE_B_PA_300/rear/15ms_PLANE_B_PA_300_000536.T000.D000.P007.H000.L.vec", path "C:/Users/PIV/Documents/mike_ensight/NACA0015_MB_G/15ms_PLANE_B_PA_300/rear/15ms_PLANE_B_PA_300_000537.T000.D000.P007.H000.L.vec", path "C:/Users/PIV/Documents/mike_ensight/NACA0015_MB_G/15ms_PLANE_B_PA_300/rear/15ms_PLANE_B_PA_300_000538.T000.D000.P007.H000.L.vec", path "C:/Users/PIV/Documents/mike_ensight/NACA0015_MB_G/15ms_PLANE_B_PA_300/rear/15ms_PLANE_B_PA_300_000539.T000.D000.P007.H000.L.vec", path "C:/Users/PIV/Documents/mike_ensight/NACA0015_MB_G/15ms_PLANE_B_PA_300/rear/15ms_PLANE_B_PA_300_000540.T000.D000.P007.H000.L.vec", path "C:/Users/PIV/Documents/mike_ensight/NACA0015_MB_G/15ms_PLANE_B_PA_300/rear/15ms_PLANE_B_PA_300_000541.T000.D000.P007.H000.L.vec", path "C:/Users/PIV/Documents/mike_ensight/NACA0015_MB_G/15ms_PLANE_B_PA_300/rear/15ms_PLANE_B_PA_300_000542.T000.D000.P007.H000.L.vec", path "C:/Users/PIV/Documents/mike_ensight/NACA0015_MB_G/15ms_PLANE_B_PA_300/rear/15ms_PLANE_B_PA_300_000543.T000.D000.P007.H000.L.vec", path "C:/Users/PIV/Documents/mike_ensight/NACA0015_MB_G/15ms_PLANE_B_PA_300/rear/15ms_PLANE_B_PA_300_000544.T000.D000.P007.H000.L.vec", path "C:/Users/PIV/Documents/mike_ensight/NACA0015_MB_G/15ms_PLANE_B_PA_300/rear/15ms_PLANE_B_PA_300_000545.T000.D000.P007.H000.L.vec", path "C:/Users/PIV/Documents/mike_ensight/NACA0015_MB_G/15ms_PLANE_B_PA_300/rear/15ms_PLANE_B_PA_300_000546.T000.D000.P007.H000.L.vec", path "C:/Users/PIV/Documents/mike_ensight/NACA0015_MB_G/15ms_PLANE_B_PA_300/rear/15ms_PLANE_B_PA_300_000547.T000.D000.P007.H000.L.vec", path "C:/Users/PIV/Documents/mike_ensight/NACA0015_MB_G/15ms_PLANE_B_PA_300/rear/15ms_PLANE_B_PA_300_000548.T000.D000.P007.H000.L.vec", path "C:/Users/PIV/Documents/mike_ensight/NACA0015_MB_G/15ms_PLANE_B_PA_300/rear/15ms_PLANE_B_PA_300_000549.T000.D000.P007.H000.L.vec", path "C:/Users/PIV/Documents/mike_ensight/NACA0015_MB_G/15ms_PLANE_B_PA_300/rear/15ms_PLANE_B_PA_300_000550.T000.D000.P007.H000.L.vec", path "C:/Users/PIV/Documents/mike_ensight/NACA0015_MB_G/15ms_PLANE_B_PA_300/rear/15ms_PLANE_B_PA_300_000551.T000.D000.P007.H000.L.vec", path "C:/Users/PIV/Documents/mike_ensight/NACA0015_MB_G/15ms_PLANE_B_PA_300/rear/15ms_PLANE_B_PA_300_000552.T000.D000.P007.H000.L.vec", path "C:/Users/PIV/Documents/mike_ensight/NACA0015_MB_G/15ms_PLANE_B_PA_300/rear/15ms_PLANE_B_PA_300_000553.T000.D000.P007.H000.L.vec", path "C:/Users/PIV/Documents/mike_ensight/NACA0015_MB_G/15ms_PLANE_B_PA_300/rear/15ms_PLANE_B_PA_300_000554.T000.D000.P007.H000.L.vec", path "C:/Users/PIV/Documents/mike_ensight/NACA0015_MB_G/15ms_PLANE_B_PA_300/rear/15ms_PLANE_B_PA_300_000555.T000.D000.P007.H000.L.vec", path "C:/Users/PIV/Documents/mike_ensight/NACA0015_MB_G/15ms_PLANE_B_PA_300/rear/15ms_PLANE_B_PA_300_000556.T000.D000.P007.H000.L.vec", path "C:/Users/PIV/Documents/mike_ensight/NACA0015_MB_G/15ms_PLANE_B_PA_300/rear/15ms_PLANE_B_PA_300_000557.T000.D000.P007.H000.L.vec", path "C:/Users/PIV/Documents/mike_ensight/NACA0015_MB_G/15ms_PLANE_B_PA_300/rear/15ms_PLANE_B_PA_300_000558.T000.D000.P007.H000.L.vec", path "C:/Users/PIV/Documents/mike_ensight/NACA0015_MB_G/15ms_PLANE_B_PA_300/rear/15ms_PLANE_B_PA_300_000559.T000.D000.P007.H000.L.vec", path "C:/Users/PIV/Documents/mike_ensight/NACA0015_MB_G/15ms_PLANE_B_PA_300/rear/15ms_PLANE_B_PA_300_000560.T000.D000.P007.H000.L.vec", path "C:/Users/PIV/Documents/mike_ensight/NACA0015_MB_G/15ms_PLANE_B_PA_300/rear/15ms_PLANE_B_PA_300_000561.T000.D000.P007.H000.L.vec", path "C:/Users/PIV/Documents/mike_ensight/NACA0015_MB_G/15ms_PLANE_B_PA_300/rear/15ms_PLANE_B_PA_300_000562.T000.D000.P007.H000.L.vec", path "C:/Users/PIV/Documents/mike_ensight/NACA0015_MB_G/15ms_PLANE_B_PA_300/rear/15ms_PLANE_B_PA_300_000563.T000.D000.P007.H000.L.vec", path "C:/Users/PIV/Documents/mike_ensight/NACA0015_MB_G/15ms_PLANE_B_PA_300/rear/15ms_PLANE_B_PA_300_000564.T000.D000.P007.H000.L.vec", path "C:/Users/PIV/Documents/mike_ensight/NACA0015_MB_G/15ms_PLANE_B_PA_300/rear/15ms_PLANE_B_PA_300_000565.T000.D000.P007.H000.L.vec", path "C:/Users/PIV/Documents/mike_ensight/NACA0015_MB_G/15ms_PLANE_B_PA_300/rear/15ms_PLANE_B_PA_300_000566.T000.D000.P007.H000.L.vec", path "C:/Users/PIV/Documents/mike_ensight/NACA0015_MB_G/15ms_PLANE_B_PA_300/rear/15ms_PLANE_B_PA_300_000567.T000.D000.P007.H000.L.vec", path "C:/Users/PIV/Documents/mike_ensight/NACA0015_MB_G/15ms_PLANE_B_PA_300/rear/15ms_PLANE_B_PA_300_000568.T000.D000.P007.H000.L.vec", path "C:/Users/PIV/Documents/mike_ensight/NACA0015_MB_G/15ms_PLANE_B_PA_300/rear/15ms_PLANE_B_PA_300_000569.T000.D000.P007.H000.L.vec", path "C:/Users/PIV/Documents/mike_ensight/NACA0015_MB_G/15ms_PLANE_B_PA_300/rear/15ms_PLANE_B_PA_300_000570.T000.D000.P007.H000.L.vec", path "C:/Users/PIV/Documents/mike_ensight/NACA0015_MB_G/15ms_PLANE_B_PA_300/rear/15ms_PLANE_B_PA_300_000571.T000.D000.P007.H000.L.vec", path "C:/Users/PIV/Documents/mike_ensight/NACA0015_MB_G/15ms_PLANE_B_PA_300/rear/15ms_PLANE_B_PA_300_000572.T000.D000.P007.H000.L.vec", path "C:/Users/PIV/Documents/mike_ensight/NACA0015_MB_G/15ms_PLANE_B_PA_300/rear/15ms_PLANE_B_PA_300_000573.T000.D000.P007.H000.L.vec", path "C:/Users/PIV/Documents/mike_ensight/NACA0015_MB_G/15ms_PLANE_B_PA_300/rear/15ms_PLANE_B_PA_300_000574.T000.D000.P007.H000.L.vec", path "C:/Users/PIV/Documents/mike_ensight/NACA0015_MB_G/15ms_PLANE_B_PA_300/rear/15ms_PLANE_B_PA_300_000575.T000.D000.P007.H000.L.vec", path "C:/Users/PIV/Documents/mike_ensight/NACA0015_MB_G/15ms_PLANE_B_PA_300/rear/15ms_PLANE_B_PA_300_000576.T000.D000.P007.H000.L.vec", path "C:/Users/PIV/Documents/mike_ensight/NACA0015_MB_G/15ms_PLANE_B_PA_300/rear/15ms_PLANE_B_PA_300_000577.T000.D000.P007.H000.L.vec", path "C:/Users/PIV/Documents/mike_ensight/NACA0015_MB_G/15ms_PLANE_B_PA_300/rear/15ms_PLANE_B_PA_300_000578.T000.D000.P007.H000.L.vec", path "C:/Users/PIV/Documents/mike_ensight/NACA0015_MB_G/15ms_PLANE_B_PA_300/rear/15ms_PLANE_B_PA_300_000579.T000.D000.P007.H000.L.vec", path "C:/Users/PIV/Documents/mike_ensight/NACA0015_MB_G/15ms_PLANE_B_PA_300/rear/15ms_PLANE_B_PA_300_000580.T000.D000.P007.H000.L.vec", path "C:/Users/PIV/Documents/mike_ensight/NACA0015_MB_G/15ms_PLANE_B_PA_300/rear/15ms_PLANE_B_PA_300_000581.T000.D000.P007.H000.L.vec", path "C:/Users/PIV/Documents/mike_ensight/NACA0015_MB_G/15ms_PLANE_B_PA_300/rear/15ms_PLANE_B_PA_300_000582.T000.D000.P007.H000.L.vec", path "C:/Users/PIV/Documents/mike_ensight/NACA0015_MB_G/15ms_PLANE_B_PA_300/rear/15ms_PLANE_B_PA_300_000583.T000.D000.P007.H000.L.vec", path "C:/Users/PIV/Documents/mike_ensight/NACA0015_MB_G/15ms_PLANE_B_PA_300/rear/15ms_PLANE_B_PA_300_000584.T000.D000.P007.H000.L.vec", path "C:/Users/PIV/Documents/mike_ensight/NACA0015_MB_G/15ms_PLANE_B_PA_300/rear/15ms_PLANE_B_PA_300_000585.T000.D000.P007.H000.L.vec", path "C:/Users/PIV/Documents/mike_ensight/NACA0015_MB_G/15ms_PLANE_B_PA_300/rear/15ms_PLANE_B_PA_300_000586.T000.D000.P007.H000.L.vec", path "C:/Users/PIV/Documents/mike_ensight/NACA0015_MB_G/15ms_PLANE_B_PA_300/rear/15ms_PLANE_B_PA_300_000587.T000.D000.P007.H000.L.vec", path "C:/Users/PIV/Documents/mike_ensight/NACA0015_MB_G/15ms_PLANE_B_PA_300/rear/15ms_PLANE_B_PA_300_000588.T000.D000.P007.H000.L.vec", path "C:/Users/PIV/Documents/mike_ensight/NACA0015_MB_G/15ms_PLANE_B_PA_300/rear/15ms_PLANE_B_PA_300_000589.T000.D000.P007.H000.L.vec", path "C:/Users/PIV/Documents/mike_ensight/NACA0015_MB_G/15ms_PLANE_B_PA_300/rear/15ms_PLANE_B_PA_300_000590.T000.D000.P007.H000.L.vec", path "C:/Users/PIV/Documents/mike_ensight/NACA0015_MB_G/15ms_PLANE_B_PA_300/rear/15ms_PLANE_B_PA_300_000591.T000.D000.P007.H000.L.vec", path "C:/Users/PIV/Documents/mike_ensight/NACA0015_MB_G/15ms_PLANE_B_PA_300/rear/15ms_PLANE_B_PA_300_000592.T000.D000.P007.H000.L.vec", path "C:/Users/PIV/Documents/mike_ensight/NACA0015_MB_G/15ms_PLANE_B_PA_300/rear/15ms_PLANE_B_PA_300_000593.T000.D000.P007.H000.L.vec", path "C:/Users/PIV/Documents/mike_ensight/NACA0015_MB_G/15ms_PLANE_B_PA_300/rear/15ms_PLANE_B_PA_300_000594.T000.D000.P007.H000.L.vec", path "C:/Users/PIV/Documents/mike_ensight/NACA0015_MB_G/15ms_PLANE_B_PA_300/rear/15ms_PLANE_B_PA_300_000595.T000.D000.P007.H000.L.vec", path "C:/Users/PIV/Documents/mike_ensight/NACA0015_MB_G/15ms_PLANE_B_PA_300/rear/15ms_PLANE_B_PA_300_000596.T000.D000.P007.H000.L.vec", path "C:/Users/PIV/Documents/mike_ensight/NACA0015_MB_G/15ms_PLANE_B_PA_300/rear/15ms_PLANE_B_PA_300_000597.T000.D000.P007.H000.L.vec", path "C:/Users/PIV/Documents/mike_ensight/NACA0015_MB_G/15ms_PLANE_B_PA_300/rear/15ms_PLANE_B_PA_300_000598.T000.D000.P007.H000.L.vec", path "C:/Users/PIV/Documents/mike_ensight/NACA0015_MB_G/15ms_PLANE_B_PA_300/rear/15ms_PLANE_B_PA_300_000599.T000.D000.P007.H000.L.vec", path "C:/Users/PIV/Documents/mike_ensight/NACA0015_MB_G/15ms_PLANE_B_PA_300/rear/15ms_PLANE_B_PA_300_000600.T000.D000.P007.H000.L.vec", path "C:/Users/PIV/Documents/mike_ensight/NACA0015_MB_G/15ms_PLANE_B_PA_300/rear/15ms_PLANE_B_PA_300_000601.T000.D000.P007.H000.L.vec", path "C:/Users/PIV/Documents/mike_ensight/NACA0015_MB_G/15ms_PLANE_B_PA_300/rear/15ms_PLANE_B_PA_300_000602.T000.D000.P007.H000.L.vec", path "C:/Users/PIV/Documents/mike_ensight/NACA0015_MB_G/15ms_PLANE_B_PA_300/rear/15ms_PLANE_B_PA_300_000603.T000.D000.P007.H000.L.vec", path "C:/Users/PIV/Documents/mike_ensight/NACA0015_MB_G/15ms_PLANE_B_PA_300/rear/15ms_PLANE_B_PA_300_000604.T000.D000.P007.H000.L.vec", path "C:/Users/PIV/Documents/mike_ensight/NACA0015_MB_G/15ms_PLANE_B_PA_300/rear/15ms_PLANE_B_PA_300_000605.T000.D000.P007.H000.L.vec", path "C:/Users/PIV/Documents/mike_ensight/NACA0015_MB_G/15ms_PLANE_B_PA_300/rear/15ms_PLANE_B_PA_300_000606.T000.D000.P007.H000.L.vec", path "C:/Users/PIV/Documents/mike_ensight/NACA0015_MB_G/15ms_PLANE_B_PA_300/rear/15ms_PLANE_B_PA_300_000607.T000.D000.P007.H000.L.vec", path "C:/Users/PIV/Documents/mike_ensight/NACA0015_MB_G/15ms_PLANE_B_PA_300/rear/15ms_PLANE_B_PA_300_000608.T000.D000.P007.H000.L.vec", path "C:/Users/PIV/Documents/mike_ensight/NACA0015_MB_G/15ms_PLANE_B_PA_300/rear/15ms_PLANE_B_PA_300_000609.T000.D000.P007.H000.L.vec", path "C:/Users/PIV/Documents/mike_ensight/NACA0015_MB_G/15ms_PLANE_B_PA_300/rear/15ms_PLANE_B_PA_300_000610.T000.D000.P007.H000.L.vec", path "C:/Users/PIV/Documents/mike_ensight/NACA0015_MB_G/15ms_PLANE_B_PA_300/rear/15ms_PLANE_B_PA_300_000611.T000.D000.P007.H000.L.vec", path "C:/Users/PIV/Documents/mike_ensight/NACA0015_MB_G/15ms_PLANE_B_PA_300/rear/15ms_PLANE_B_PA_300_000612.T000.D000.P007.H000.L.vec", path "C:/Users/PIV/Documents/mike_ensight/NACA0015_MB_G/15ms_PLANE_B_PA_300/rear/15ms_PLANE_B_PA_300_000613.T000.D000.P007.H000.L.vec", path "C:/Users/PIV/Documents/mike_ensight/NACA0015_MB_G/15ms_PLANE_B_PA_300/rear/15ms_PLANE_B_PA_300_000614.T000.D000.P007.H000.L.vec", path "C:/Users/PIV/Documents/mike_ensight/NACA0015_MB_G/15ms_PLANE_B_PA_300/rear/15ms_PLANE_B_PA_300_000615.T000.D000.P007.H000.L.vec", path "C:/Users/PIV/Documents/mike_ensight/NACA0015_MB_G/15ms_PLANE_B_PA_300/rear/15ms_PLANE_B_PA_300_000616.T000.D000.P007.H000.L.vec", path "C:/Users/PIV/Documents/mike_ensight/NACA0015_MB_G/15ms_PLANE_B_PA_300/rear/15ms_PLANE_B_PA_300_000617.T000.D000.P007.H000.L.vec", path "C:/Users/PIV/Documents/mike_ensight/NACA0015_MB_G/15ms_PLANE_B_PA_300/rear/15ms_PLANE_B_PA_300_000618.T000.D000.P007.H000.L.vec", path "C:/Users/PIV/Documents/mike_ensight/NACA0015_MB_G/15ms_PLANE_B_PA_300/rear/15ms_PLANE_B_PA_300_000619.T000.D000.P007.H000.L.vec", path "C:/Users/PIV/Documents/mike_ensight/NACA0015_MB_G/15ms_PLANE_B_PA_300/rear/15ms_PLANE_B_PA_300_000620.T000.D000.P007.H000.L.vec", path "C:/Users/PIV/Documents/mike_ensight/NACA0015_MB_G/15ms_PLANE_B_PA_300/rear/15ms_PLANE_B_PA_300_000621.T000.D000.P007.H000.L.vec", path "C:/Users/PIV/Documents/mike_ensight/NACA0015_MB_G/15ms_PLANE_B_PA_300/rear/15ms_PLANE_B_PA_300_000622.T000.D000.P007.H000.L.vec", path "C:/Users/PIV/Documents/mike_ensight/NACA0015_MB_G/15ms_PLANE_B_PA_300/rear/15ms_PLANE_B_PA_300_000623.T000.D000.P007.H000.L.vec", path "C:/Users/PIV/Documents/mike_ensight/NACA0015_MB_G/15ms_PLANE_B_PA_300/rear/15ms_PLANE_B_PA_300_000624.T000.D000.P007.H000.L.vec", path "C:/Users/PIV/Documents/mike_ensight/NACA0015_MB_G/15ms_PLANE_B_PA_300/rear/15ms_PLANE_B_PA_300_000625.T000.D000.P007.H000.L.vec", path "C:/Users/PIV/Documents/mike_ensight/NACA0015_MB_G/15ms_PLANE_B_PA_300/rear/15ms_PLANE_B_PA_300_000626.T000.D000.P007.H000.L.vec", path "C:/Users/PIV/Documents/mike_ensight/NACA0015_MB_G/15ms_PLANE_B_PA_300/rear/15ms_PLANE_B_PA_300_000627.T000.D000.P007.H000.L.vec", path "C:/Users/PIV/Documents/mike_ensight/NACA0015_MB_G/15ms_PLANE_B_PA_300/rear/15ms_PLANE_B_PA_300_000628.T000.D000.P007.H000.L.vec", path "C:/Users/PIV/Documents/mike_ensight/NACA0015_MB_G/15ms_PLANE_B_PA_300/rear/15ms_PLANE_B_PA_300_000629.T000.D000.P007.H000.L.vec", path "C:/Users/PIV/Documents/mike_ensight/NACA0015_MB_G/15ms_PLANE_B_PA_300/rear/15ms_PLANE_B_PA_300_000630.T000.D000.P007.H000.L.vec", path "C:/Users/PIV/Documents/mike_ensight/NACA0015_MB_G/15ms_PLANE_B_PA_300/rear/15ms_PLANE_B_PA_300_000631.T000.D000.P007.H000.L.vec", path "C:/Users/PIV/Documents/mike_ensight/NACA0015_MB_G/15ms_PLANE_B_PA_300/rear/15ms_PLANE_B_PA_300_000632.T000.D000.P007.H000.L.vec", path "C:/Users/PIV/Documents/mike_ensight/NACA0015_MB_G/15ms_PLANE_B_PA_300/rear/15ms_PLANE_B_PA_300_000633.T000.D000.P007.H000.L.vec", path "C:/Users/PIV/Documents/mike_ensight/NACA0015_MB_G/15ms_PLANE_B_PA_300/rear/15ms_PLANE_B_PA_300_000634.T000.D000.P007.H000.L.vec", path "C:/Users/PIV/Documents/mike_ensight/NACA0015_MB_G/15ms_PLANE_B_PA_300/rear/15ms_PLANE_B_PA_300_000635.T000.D000.P007.H000.L.vec", path "C:/Users/PIV/Documents/mike_ensight/NACA0015_MB_G/15ms_PLANE_B_PA_300/rear/15ms_PLANE_B_PA_300_000636.T000.D000.P007.H000.L.vec", path "C:/Users/PIV/Documents/mike_ensight/NACA0015_MB_G/15ms_PLANE_B_PA_300/rear/15ms_PLANE_B_PA_300_000637.T000.D000.P007.H000.L.vec", path "C:/Users/PIV/Documents/mike_ensight/NACA0015_MB_G/15ms_PLANE_B_PA_300/rear/15ms_PLANE_B_PA_300_000638.T000.D000.P007.H000.L.vec", path "C:/Users/PIV/Documents/mike_ensight/NACA0015_MB_G/15ms_PLANE_B_PA_300/rear/15ms_PLANE_B_PA_300_000639.T000.D000.P007.H000.L.vec", path "C:/Users/PIV/Documents/mike_ensight/NACA0015_MB_G/15ms_PLANE_B_PA_300/rear/15ms_PLANE_B_PA_300_000640.T000.D000.P007.H000.L.vec", path "C:/Users/PIV/Documents/mike_ensight/NACA0015_MB_G/15ms_PLANE_B_PA_300/rear/15ms_PLANE_B_PA_300_000641.T000.D000.P007.H000.L.vec", path "C:/Users/PIV/Documents/mike_ensight/NACA0015_MB_G/15ms_PLANE_B_PA_300/rear/15ms_PLANE_B_PA_300_000642.T000.D000.P007.H000.L.vec", path "C:/Users/PIV/Documents/mike_ensight/NACA0015_MB_G/15ms_PLANE_B_PA_300/rear/15ms_PLANE_B_PA_300_000643.T000.D000.P007.H000.L.vec", path "C:/Users/PIV/Documents/mike_ensight/NACA0015_MB_G/15ms_PLANE_B_PA_300/rear/15ms_PLANE_B_PA_300_000644.T000.D000.P007.H000.L.vec", path "C:/Users/PIV/Documents/mike_ensight/NACA0015_MB_G/15ms_PLANE_B_PA_300/rear/15ms_PLANE_B_PA_300_000645.T000.D000.P007.H000.L.vec", path "C:/Users/PIV/Documents/mike_ensight/NACA0015_MB_G/15ms_PLANE_B_PA_300/rear/15ms_PLANE_B_PA_300_000646.T000.D000.P007.H000.L.vec", path "C:/Users/PIV/Documents/mike_ensight/NACA0015_MB_G/15ms_PLANE_B_PA_300/rear/15ms_PLANE_B_PA_300_000647.T000.D000.P007.H000.L.vec", path "C:/Users/PIV/Documents/mike_ensight/NACA0015_MB_G/15ms_PLANE_B_PA_300/rear/15ms_PLANE_B_PA_300_000648.T000.D000.P007.H000.L.vec", path "C:/Users/PIV/Documents/mike_ensight/NACA0015_MB_G/15ms_PLANE_B_PA_300/rear/15ms_PLANE_B_PA_300_000649.T000.D000.P007.H000.L.vec", path "C:/Users/PIV/Documents/mike_ensight/NACA0015_MB_G/15ms_PLANE_B_PA_300/rear/15ms_PLANE_B_PA_300_000650.T000.D000.P007.H000.L.vec", path "C:/Users/PIV/Documents/mike_ensight/NACA0015_MB_G/15ms_PLANE_B_PA_300/rear/15ms_PLANE_B_PA_300_000651.T000.D000.P007.H000.L.vec", path "C:/Users/PIV/Documents/mike_ensight/NACA0015_MB_G/15ms_PLANE_B_PA_300/rear/15ms_PLANE_B_PA_300_000652.T000.D000.P007.H000.L.vec", path "C:/Users/PIV/Documents/mike_ensight/NACA0015_MB_G/15ms_PLANE_B_PA_300/rear/15ms_PLANE_B_PA_300_000653.T000.D000.P007.H000.L.vec", path "C:/Users/PIV/Documents/mike_ensight/NACA0015_MB_G/15ms_PLANE_B_PA_300/rear/15ms_PLANE_B_PA_300_000654.T000.D000.P007.H000.L.vec", path "C:/Users/PIV/Documents/mike_ensight/NACA0015_MB_G/15ms_PLANE_B_PA_300/rear/15ms_PLANE_B_PA_300_000655.T000.D000.P007.H000.L.vec", path "C:/Users/PIV/Documents/mike_ensight/NACA0015_MB_G/15ms_PLANE_B_PA_300/rear/15ms_PLANE_B_PA_300_000656.T000.D000.P007.H000.L.vec", path "C:/Users/PIV/Documents/mike_ensight/NACA0015_MB_G/15ms_PLANE_B_PA_300/rear/15ms_PLANE_B_PA_300_000657.T000.D000.P007.H000.L.vec", path "C:/Users/PIV/Documents/mike_ensight/NACA0015_MB_G/15ms_PLANE_B_PA_300/rear/15ms_PLANE_B_PA_300_000658.T000.D000.P007.H000.L.vec", path "C:/Users/PIV/Documents/mike_ensight/NACA0015_MB_G/15ms_PLANE_B_PA_300/rear/15ms_PLANE_B_PA_300_000659.T000.D000.P007.H000.L.vec", path "C:/Users/PIV/Documents/mike_ensight/NACA0015_MB_G/15ms_PLANE_B_PA_300/rear/15ms_PLANE_B_PA_300_000660.T000.D000.P007.H000.L.vec", path "C:/Users/PIV/Documents/mike_ensight/NACA0015_MB_G/15ms_PLANE_B_PA_300/rear/15ms_PLANE_B_PA_300_000661.T000.D000.P007.H000.L.vec", path "C:/Users/PIV/Documents/mike_ensight/NACA0015_MB_G/15ms_PLANE_B_PA_300/rear/15ms_PLANE_B_PA_300_000662.T000.D000.P007.H000.L.vec", path "C:/Users/PIV/Documents/mike_ensight/NACA0015_MB_G/15ms_PLANE_B_PA_300/rear/15ms_PLANE_B_PA_300_000663.T000.D000.P007.H000.L.vec", path "C:/Users/PIV/Documents/mike_ensight/NACA0015_MB_G/15ms_PLANE_B_PA_300/rear/15ms_PLANE_B_PA_300_000664.T000.D000.P007.H000.L.vec", path "C:/Users/PIV/Documents/mike_ensight/NACA0015_MB_G/15ms_PLANE_B_PA_300/rear/15ms_PLANE_B_PA_300_000665.T000.D000.P007.H000.L.vec", path "C:/Users/PIV/Documents/mike_ensight/NACA0015_MB_G/15ms_PLANE_B_PA_300/rear/15ms_PLANE_B_PA_300_000666.T000.D000.P007.H000.L.vec", path "C:/Users/PIV/Documents/mike_ensight/NACA0015_MB_G/15ms_PLANE_B_PA_300/rear/15ms_PLANE_B_PA_300_000667.T000.D000.P007.H000.L.vec", path "C:/Users/PIV/Documents/mike_ensight/NACA0015_MB_G/15ms_PLANE_B_PA_300/rear/15ms_PLANE_B_PA_300_000668.T000.D000.P007.H000.L.vec", path "C:/Users/PIV/Documents/mike_ensight/NACA0015_MB_G/15ms_PLANE_B_PA_300/rear/15ms_PLANE_B_PA_300_000669.T000.D000.P007.H000.L.vec", path "C:/Users/PIV/Documents/mike_ensight/NACA0015_MB_G/15ms_PLANE_B_PA_300/rear/15ms_PLANE_B_PA_300_000670.T000.D000.P007.H000.L.vec", path "C:/Users/PIV/Documents/mike_ensight/NACA0015_MB_G/15ms_PLANE_B_PA_300/rear/15ms_PLANE_B_PA_300_000671.T000.D000.P007.H000.L.vec", path "C:/Users/PIV/Documents/mike_ensight/NACA0015_MB_G/15ms_PLANE_B_PA_300/rear/15ms_PLANE_B_PA_300_000672.T000.D000.P007.H000.L.vec", path "C:/Users/PIV/Documents/mike_ensight/NACA0015_MB_G/15ms_PLANE_B_PA_300/rear/15ms_PLANE_B_PA_300_000673.T000.D000.P007.H000.L.vec", path "C:/Users/PIV/Documents/mike_ensight/NACA0015_MB_G/15ms_PLANE_B_PA_300/rear/15ms_PLANE_B_PA_300_000674.T000.D000.P007.H000.L.vec", path "C:/Users/PIV/Documents/mike_ensight/NACA0015_MB_G/15ms_PLANE_B_PA_300/rear/15ms_PLANE_B_PA_300_000675.T000.D000.P007.H000.L.vec", path "C:/Users/PIV/Documents/mike_ensight/NACA0015_MB_G/15ms_PLANE_B_PA_300/rear/15ms_PLANE_B_PA_300_000676.T000.D000.P007.H000.L.vec", path "C:/Users/PIV/Documents/mike_ensight/NACA0015_MB_G/15ms_PLANE_B_PA_300/rear/15ms_PLANE_B_PA_300_000677.T000.D000.P007.H000.L.vec", path "C:/Users/PIV/Documents/mike_ensight/NACA0015_MB_G/15ms_PLANE_B_PA_300/rear/15ms_PLANE_B_PA_300_000678.T000.D000.P007.H000.L.vec", path "C:/Users/PIV/Documents/mike_ensight/NACA0015_MB_G/15ms_PLANE_B_PA_300/rear/15ms_PLANE_B_PA_300_000679.T000.D000.P007.H000.L.vec", path "C:/Users/PIV/Documents/mike_ensight/NACA0015_MB_G/15ms_PLANE_B_PA_300/rear/15ms_PLANE_B_PA_300_000680.T000.D000.P007.H000.L.vec", path "C:/Users/PIV/Documents/mike_ensight/NACA0015_MB_G/15ms_PLANE_B_PA_300/rear/15ms_PLANE_B_PA_300_000681.T000.D000.P007.H000.L.vec", path "C:/Users/PIV/Documents/mike_ensight/NACA0015_MB_G/15ms_PLANE_B_PA_300/rear/15ms_PLANE_B_PA_300_000682.T000.D000.P007.H000.L.vec", path "C:/Users/PIV/Documents/mike_ensight/NACA0015_MB_G/15ms_PLANE_B_PA_300/rear/15ms_PLANE_B_PA_300_000683.T000.D000.P007.H000.L.vec", path "C:/Users/PIV/Documents/mike_ensight/NACA0015_MB_G/15ms_PLANE_B_PA_300/rear/15ms_PLANE_B_PA_300_000684.T000.D000.P007.H000.L.vec", path "C:/Users/PIV/Documents/mike_ensight/NACA0015_MB_G/15ms_PLANE_B_PA_300/rear/15ms_PLANE_B_PA_300_000685.T000.D000.P007.H000.L.vec", path "C:/Users/PIV/Documents/mike_ensight/NACA0015_MB_G/15ms_PLANE_B_PA_300/rear/15ms_PLANE_B_PA_300_000686.T000.D000.P007.H000.L.vec", path "C:/Users/PIV/Documents/mike_ensight/NACA0015_MB_G/15ms_PLANE_B_PA_300/rear/15ms_PLANE_B_PA_300_000687.T000.D000.P007.H000.L.vec", path "C:/Users/PIV/Documents/mike_ensight/NACA0015_MB_G/15ms_PLANE_B_PA_300/rear/15ms_PLANE_B_PA_300_000688.T000.D000.P007.H000.L.vec", path "C:/Users/PIV/Documents/mike_ensight/NACA0015_MB_G/15ms_PLANE_B_PA_300/rear/15ms_PLANE_B_PA_300_000689.T000.D000.P007.H000.L.vec", path "C:/Users/PIV/Documents/mike_ensight/NACA0015_MB_G/15ms_PLANE_B_PA_300/rear/15ms_PLANE_B_PA_300_000690.T000.D000.P007.H000.L.vec", path "C:/Users/PIV/Documents/mike_ensight/NACA0015_MB_G/15ms_PLANE_B_PA_300/rear/15ms_PLANE_B_PA_300_000691.T000.D000.P007.H000.L.vec", path "C:/Users/PIV/Documents/mike_ensight/NACA0015_MB_G/15ms_PLANE_B_PA_300/rear/15ms_PLANE_B_PA_300_000692.T000.D000.P007.H000.L.vec", path "C:/Users/PIV/Documents/mike_ensight/NACA0015_MB_G/15ms_PLANE_B_PA_300/rear/15ms_PLANE_B_PA_300_000693.T000.D000.P007.H000.L.vec", path "C:/Users/PIV/Documents/mike_ensight/NACA0015_MB_G/15ms_PLANE_B_PA_300/rear/15ms_PLANE_B_PA_300_000694.T000.D000.P007.H000.L.vec", path "C:/Users/PIV/Documents/mike_ensight/NACA0015_MB_G/15ms_PLANE_B_PA_300/rear/15ms_PLANE_B_PA_300_000695.T000.D000.P007.H000.L.vec", path "C:/Users/PIV/Documents/mike_ensight/NACA0015_MB_G/15ms_PLANE_B_PA_300/rear/15ms_PLANE_B_PA_300_000696.T000.D000.P007.H000.L.vec", path "C:/Users/PIV/Documents/mike_ensight/NACA0015_MB_G/15ms_PLANE_B_PA_300/rear/15ms_PLANE_B_PA_300_000697.T000.D000.P007.H000.L.vec", path "C:/Users/PIV/Documents/mike_ensight/NACA0015_MB_G/15ms_PLANE_B_PA_300/rear/15ms_PLANE_B_PA_300_000698.T000.D000.P007.H000.L.vec", path "C:/Users/PIV/Documents/mike_ensight/NACA0015_MB_G/15ms_PLANE_B_PA_300/rear/15ms_PLANE_B_PA_300_000699.T000.D000.P007.H000.L.vec", path "C:/Users/PIV/Documents/mike_ensight/NACA0015_MB_G/15ms_PLANE_B_PA_300/rear/15ms_PLANE_B_PA_300_000700.T000.D000.P007.H000.L.vec", path "C:/Users/PIV/Documents/mike_ensight/NACA0015_MB_G/15ms_PLANE_B_PA_300/rear/15ms_PLANE_B_PA_300_000701.T000.D000.P007.H000.L.vec", path "C:/Users/PIV/Documents/mike_ensight/NACA0015_MB_G/15ms_PLANE_B_PA_300/rear/15ms_PLANE_B_PA_300_000702.T000.D000.P007.H000.L.vec", path "C:/Users/PIV/Documents/mike_ensight/NACA0015_MB_G/15ms_PLANE_B_PA_300/rear/15ms_PLANE_B_PA_300_000703.T000.D000.P007.H000.L.vec", path "C:/Users/PIV/Documents/mike_ensight/NACA0015_MB_G/15ms_PLANE_B_PA_300/rear/15ms_PLANE_B_PA_300_000704.T000.D000.P007.H000.L.vec", path "C:/Users/PIV/Documents/mike_ensight/NACA0015_MB_G/15ms_PLANE_B_PA_300/rear/15ms_PLANE_B_PA_300_000705.T000.D000.P007.H000.L.vec", path "C:/Users/PIV/Documents/mike_ensight/NACA0015_MB_G/15ms_PLANE_B_PA_300/rear/15ms_PLANE_B_PA_300_000706.T000.D000.P007.H000.L.vec", path "C:/Users/PIV/Documents/mike_ensight/NACA0015_MB_G/15ms_PLANE_B_PA_300/rear/15ms_PLANE_B_PA_300_000707.T000.D000.P007.H000.L.vec", path "C:/Users/PIV/Documents/mike_ensight/NACA0015_MB_G/15ms_PLANE_B_PA_300/rear/15ms_PLANE_B_PA_300_000708.T000.D000.P007.H000.L.vec", path "C:/Users/PIV/Documents/mike_ensight/NACA0015_MB_G/15ms_PLANE_B_PA_300/rear/15ms_PLANE_B_PA_300_000709.T000.D000.P007.H000.L.vec", path "C:/Users/PIV/Documents/mike_ensight/NACA0015_MB_G/15ms_PLANE_B_PA_300/rear/15ms_PLANE_B_PA_300_000710.T000.D000.P007.H000.L.vec", path "C:/Users/PIV/Documents/mike_ensight/NACA0015_MB_G/15ms_PLANE_B_PA_300/rear/15ms_PLANE_B_PA_300_000711.T000.D000.P007.H000.L.vec", path "C:/Users/PIV/Documents/mike_ensight/NACA0015_MB_G/15ms_PLANE_B_PA_300/rear/15ms_PLANE_B_PA_300_000712.T000.D000.P007.H000.L.vec", path "C:/Users/PIV/Documents/mike_ensight/NACA0015_MB_G/15ms_PLANE_B_PA_300/rear/15ms_PLANE_B_PA_300_000713.T000.D000.P007.H000.L.vec", path "C:/Users/PIV/Documents/mike_ensight/NACA0015_MB_G/15ms_PLANE_B_PA_300/rear/15ms_PLANE_B_PA_300_000714.T000.D000.P007.H000.L.vec", path "C:/Users/PIV/Documents/mike_ensight/NACA0015_MB_G/15ms_PLANE_B_PA_300/rear/15ms_PLANE_B_PA_300_000715.T000.D000.P007.H000.L.vec", path "C:/Users/PIV/Documents/mike_ensight/NACA0015_MB_G/15ms_PLANE_B_PA_300/rear/15ms_PLANE_B_PA_300_000716.T000.D000.P007.H000.L.vec", path "C:/Users/PIV/Documents/mike_ensight/NACA0015_MB_G/15ms_PLANE_B_PA_300/rear/15ms_PLANE_B_PA_300_000717.T000.D000.P007.H000.L.vec", path "C:/Users/PIV/Documents/mike_ensight/NACA0015_MB_G/15ms_PLANE_B_PA_300/rear/15ms_PLANE_B_PA_300_000718.T000.D000.P007.H000.L.vec", path "C:/Users/PIV/Documents/mike_ensight/NACA0015_MB_G/15ms_PLANE_B_PA_300/rear/15ms_PLANE_B_PA_300_000719.T000.D000.P007.H000.L.vec", path "C:/Users/PIV/Documents/mike_ensight/NACA0015_MB_G/15ms_PLANE_B_PA_300/rear/15ms_PLANE_B_PA_300_000720.T000.D000.P007.H000.L.vec", path "C:/Users/PIV/Documents/mike_ensight/NACA0015_MB_G/15ms_PLANE_B_PA_300/rear/15ms_PLANE_B_PA_300_000721.T000.D000.P007.H000.L.vec", path "C:/Users/PIV/Documents/mike_ensight/NACA0015_MB_G/15ms_PLANE_B_PA_300/rear/15ms_PLANE_B_PA_300_000722.T000.D000.P007.H000.L.vec", path "C:/Users/PIV/Documents/mike_ensight/NACA0015_MB_G/15ms_PLANE_B_PA_300/rear/15ms_PLANE_B_PA_300_000723.T000.D000.P007.H000.L.vec", path "C:/Users/PIV/Documents/mike_ensight/NACA0015_MB_G/15ms_PLANE_B_PA_300/rear/15ms_PLANE_B_PA_300_000724.T000.D000.P007.H000.L.vec", path "C:/Users/PIV/Documents/mike_ensight/NACA0015_MB_G/15ms_PLANE_B_PA_300/rear/15ms_PLANE_B_PA_300_000725.T000.D000.P007.H000.L.vec", path "C:/Users/PIV/Documents/mike_ensight/NACA0015_MB_G/15ms_PLANE_B_PA_300/rear/15ms_PLANE_B_PA_300_000726.T000.D000.P007.H000.L.vec", path "C:/Users/PIV/Documents/mike_ensight/NACA0015_MB_G/15ms_PLANE_B_PA_300/rear/15ms_PLANE_B_PA_300_000727.T000.D000.P007.H000.L.vec", path "C:/Users/PIV/Documents/mike_ensight/NACA0015_MB_G/15ms_PLANE_B_PA_300/rear/15ms_PLANE_B_PA_300_000728.T000.D000.P007.H000.L.vec", path "C:/Users/PIV/Documents/mike_ensight/NACA0015_MB_G/15ms_PLANE_B_PA_300/rear/15ms_PLANE_B_PA_300_000729.T000.D000.P007.H000.L.vec", path "C:/Users/PIV/Documents/mike_ensight/NACA0015_MB_G/15ms_PLANE_B_PA_300/rear/15ms_PLANE_B_PA_300_000730.T000.D000.P007.H000.L.vec", path "C:/Users/PIV/Documents/mike_ensight/NACA0015_MB_G/15ms_PLANE_B_PA_300/rear/15ms_PLANE_B_PA_300_000731.T000.D000.P007.H000.L.vec", path "C:/Users/PIV/Documents/mike_ensight/NACA0015_MB_G/15ms_PLANE_B_PA_300/rear/15ms_PLANE_B_PA_300_000732.T000.D000.P007.H000.L.vec", path "C:/Users/PIV/Documents/mike_ensight/NACA0015_MB_G/15ms_PLANE_B_PA_300/rear/15ms_PLANE_B_PA_300_000733.T000.D000.P007.H000.L.vec", path "C:/Users/PIV/Documents/mike_ensight/NACA0015_MB_G/15ms_PLANE_B_PA_300/rear/15ms_PLANE_B_PA_300_000734.T000.D000.P007.H000.L.vec", path "C:/Users/PIV/Documents/mike_ensight/NACA0015_MB_G/15ms_PLANE_B_PA_300/rear/15ms_PLANE_B_PA_300_000735.T000.D000.P007.H000.L.vec", path "C:/Users/PIV/Documents/mike_ensight/NACA0015_MB_G/15ms_PLANE_B_PA_300/rear/15ms_PLANE_B_PA_300_000736.T000.D000.P007.H000.L.vec", path "C:/Users/PIV/Documents/mike_ensight/NACA0015_MB_G/15ms_PLANE_B_PA_300/rear/15ms_PLANE_B_PA_300_000737.T000.D000.P007.H000.L.vec", path "C:/Users/PIV/Documents/mike_ensight/NACA0015_MB_G/15ms_PLANE_B_PA_300/rear/15ms_PLANE_B_PA_300_000738.T000.D000.P007.H000.L.vec", path "C:/Users/PIV/Documents/mike_ensight/NACA0015_MB_G/15ms_PLANE_B_PA_300/rear/15ms_PLANE_B_PA_300_000739.T000.D000.P007.H000.L.vec", path "C:/Users/PIV/Documents/mike_ensight/NACA0015_MB_G/15ms_PLANE_B_PA_300/rear/15ms_PLANE_B_PA_300_000740.T000.D000.P007.H000.L.vec", path "C:/Users/PIV/Documents/mike_ensight/NACA0015_MB_G/15ms_PLANE_B_PA_300/rear/15ms_PLANE_B_PA_300_000741.T000.D000.P007.H000.L.vec", path "C:/Users/PIV/Documents/mike_ensight/NACA0015_MB_G/15ms_PLANE_B_PA_300/rear/15ms_PLANE_B_PA_300_000742.T000.D000.P007.H000.L.vec", path "C:/Users/PIV/Documents/mike_ensight/NACA0015_MB_G/15ms_PLANE_B_PA_300/rear/15ms_PLANE_B_PA_300_000743.T000.D000.P007.H000.L.vec", path "C:/Users/PIV/Documents/mike_ensight/NACA0015_MB_G/15ms_PLANE_B_PA_300/rear/15ms_PLANE_B_PA_300_000744.T000.D000.P007.H000.L.vec", path "C:/Users/PIV/Documents/mike_ensight/NACA0015_MB_G/15ms_PLANE_B_PA_300/rear/15ms_PLANE_B_PA_300_000745.T000.D000.P007.H000.L.vec", path "C:/Users/PIV/Documents/mike_ensight/NACA0015_MB_G/15ms_PLANE_B_PA_300/rear/15ms_PLANE_B_PA_300_000746.T000.D000.P007.H000.L.vec", path "C:/Users/PIV/Documents/mike_ensight/NACA0015_MB_G/15ms_PLANE_B_PA_300/rear/15ms_PLANE_B_PA_300_000747.T000.D000.P007.H000.L.vec", path "C:/Users/PIV/Documents/mike_ensight/NACA0015_MB_G/15ms_PLANE_B_PA_300/rear/15ms_PLANE_B_PA_300_000748.T000.D000.P007.H000.L.vec", path "C:/Users/PIV/Documents/mike_ensight/NACA0015_MB_G/15ms_PLANE_B_PA_300/rear/15ms_PLANE_B_PA_300_000749.T000.D000.P007.H000.L.vec", path "C:/Users/PIV/Documents/mike_ensight/NACA0015_MB_G/15ms_PLANE_B_PA_300/rear/15ms_PLANE_B_PA_300_000750.T000.D000.P007.H000.L.vec", path "C:/Users/PIV/Documents/mike_ensight/NACA0015_MB_G/15ms_PLANE_B_PA_300/rear/15ms_PLANE_B_PA_300_000751.T000.D000.P007.H000.L.vec", path "C:/Users/PIV/Documents/mike_ensight/NACA0015_MB_G/15ms_PLANE_B_PA_300/rear/15ms_PLANE_B_PA_300_000752.T000.D000.P007.H000.L.vec", path "C:/Users/PIV/Documents/mike_ensight/NACA0015_MB_G/15ms_PLANE_B_PA_300/rear/15ms_PLANE_B_PA_300_000753.T000.D000.P007.H000.L.vec", path "C:/Users/PIV/Documents/mike_ensight/NACA0015_MB_G/15ms_PLANE_B_PA_300/rear/15ms_PLANE_B_PA_300_000754.T000.D000.P007.H000.L.vec", path "C:/Users/PIV/Documents/mike_ensight/NACA0015_MB_G/15ms_PLANE_B_PA_300/rear/15ms_PLANE_B_PA_300_000755.T000.D000.P007.H000.L.vec", path "C:/Users/PIV/Documents/mike_ensight/NACA0015_MB_G/15ms_PLANE_B_PA_300/rear/15ms_PLANE_B_PA_300_000756.T000.D000.P007.H000.L.vec", path "C:/Users/PIV/Documents/mike_ensight/NACA0015_MB_G/15ms_PLANE_B_PA_300/rear/15ms_PLANE_B_PA_300_000757.T000.D000.P007.H000.L.vec", path "C:/Users/PIV/Documents/mike_ensight/NACA0015_MB_G/15ms_PLANE_B_PA_300/rear/15ms_PLANE_B_PA_300_000758.T000.D000.P007.H000.L.vec", path "C:/Users/PIV/Documents/mike_ensight/NACA0015_MB_G/15ms_PLANE_B_PA_300/rear/15ms_PLANE_B_PA_300_000759.T000.D000.P007.H000.L.vec", path "C:/Users/PIV/Documents/mike_ensight/NACA0015_MB_G/15ms_PLANE_B_PA_300/rear/15ms_PLANE_B_PA_300_000760.T000.D000.P007.H000.L.vec", path "C:/Users/PIV/Documents/mike_ensight/NACA0015_MB_G/15ms_PLANE_B_PA_300/rear/15ms_PLANE_B_PA_300_000761.T000.D000.P007.H000.L.vec", path "C:/Users/PIV/Documents/mike_ensight/NACA0015_MB_G/15ms_PLANE_B_PA_300/rear/15ms_PLANE_B_PA_300_000762.T000.D000.P007.H000.L.vec", path "C:/Users/PIV/Documents/mike_ensight/NACA0015_MB_G/15ms_PLANE_B_PA_300/rear/15ms_PLANE_B_PA_300_000763.T000.D000.P007.H000.L.vec", path "C:/Users/PIV/Documents/mike_ensight/NACA0015_MB_G/15ms_PLANE_B_PA_300/rear/15ms_PLANE_B_PA_300_000764.T000.D000.P007.H000.L.vec", path "C:/Users/PIV/Documents/mike_ensight/NACA0015_MB_G/15ms_PLANE_B_PA_300/rear/15ms_PLANE_B_PA_300_000765.T000.D000.P007.H000.L.vec", path "C:/Users/PIV/Documents/mike_ensight/NACA0015_MB_G/15ms_PLANE_B_PA_300/rear/15ms_PLANE_B_PA_300_000766.T000.D000.P007.H000.L.vec", path "C:/Users/PIV/Documents/mike_ensight/NACA0015_MB_G/15ms_PLANE_B_PA_300/rear/15ms_PLANE_B_PA_300_000767.T000.D000.P007.H000.L.vec", path "C:/Users/PIV/Documents/mike_ensight/NACA0015_MB_G/15ms_PLANE_B_PA_300/rear/15ms_PLANE_B_PA_300_000768.T000.D000.P007.H000.L.vec", path "C:/Users/PIV/Documents/mike_ensight/NACA0015_MB_G/15ms_PLANE_B_PA_300/rear/15ms_PLANE_B_PA_300_000769.T000.D000.P007.H000.L.vec", path "C:/Users/PIV/Documents/mike_ensight/NACA0015_MB_G/15ms_PLANE_B_PA_300/rear/15ms_PLANE_B_PA_300_000770.T000.D000.P007.H000.L.vec", path "C:/Users/PIV/Documents/mike_ensight/NACA0015_MB_G/15ms_PLANE_B_PA_300/rear/15ms_PLANE_B_PA_300_000771.T000.D000.P007.H000.L.vec", path "C:/Users/PIV/Documents/mike_ensight/NACA0015_MB_G/15ms_PLANE_B_PA_300/rear/15ms_PLANE_B_PA_300_000772.T000.D000.P007.H000.L.vec", path "C:/Users/PIV/Documents/mike_ensight/NACA0015_MB_G/15ms_PLANE_B_PA_300/rear/15ms_PLANE_B_PA_300_000773.T000.D000.P007.H000.L.vec", path "C:/Users/PIV/Documents/mike_ensight/NACA0015_MB_G/15ms_PLANE_B_PA_300/rear/15ms_PLANE_B_PA_300_000774.T000.D000.P007.H000.L.vec", path "C:/Users/PIV/Documents/mike_ensight/NACA0015_MB_G/15ms_PLANE_B_PA_300/rear/15ms_PLANE_B_PA_300_000775.T000.D000.P007.H000.L.vec", path "C:/Users/PIV/Documents/mike_ensight/NACA0015_MB_G/15ms_PLANE_B_PA_300/rear/15ms_PLANE_B_PA_300_000776.T000.D000.P007.H000.L.vec", path "C:/Users/PIV/Documents/mike_ensight/NACA0015_MB_G/15ms_PLANE_B_PA_300/rear/15ms_PLANE_B_PA_300_000777.T000.D000.P007.H000.L.vec", path "C:/Users/PIV/Documents/mike_ensight/NACA0015_MB_G/15ms_PLANE_B_PA_300/rear/15ms_PLANE_B_PA_300_000778.T000.D000.P007.H000.L.vec", path "C:/Users/PIV/Documents/mike_ensight/NACA0015_MB_G/15ms_PLANE_B_PA_300/rear/15ms_PLANE_B_PA_300_000779.T000.D000.P007.H000.L.vec", path "C:/Users/PIV/Documents/mike_ensight/NACA0015_MB_G/15ms_PLANE_B_PA_300/rear/15ms_PLANE_B_PA_300_000780.T000.D000.P007.H000.L.vec", path "C:/Users/PIV/Documents/mike_ensight/NACA0015_MB_G/15ms_PLANE_B_PA_300/rear/15ms_PLANE_B_PA_300_000781.T000.D000.P007.H000.L.vec", path "C:/Users/PIV/Documents/mike_ensight/NACA0015_MB_G/15ms_PLANE_B_PA_300/rear/15ms_PLANE_B_PA_300_000782.T000.D000.P007.H000.L.vec", path "C:/Users/PIV/Documents/mike_ensight/NACA0015_MB_G/15ms_PLANE_B_PA_300/rear/15ms_PLANE_B_PA_300_000783.T000.D000.P007.H000.L.vec", path "C:/Users/PIV/Documents/mike_ensight/NACA0015_MB_G/15ms_PLANE_B_PA_300/rear/15ms_PLANE_B_PA_300_000784.T000.D000.P007.H000.L.vec", path "C:/Users/PIV/Documents/mike_ensight/NACA0015_MB_G/15ms_PLANE_B_PA_300/rear/15ms_PLANE_B_PA_300_000785.T000.D000.P007.H000.L.vec", path "C:/Users/PIV/Documents/mike_ensight/NACA0015_MB_G/15ms_PLANE_B_PA_300/rear/15ms_PLANE_B_PA_300_000786.T000.D000.P007.H000.L.vec", path "C:/Users/PIV/Documents/mike_ensight/NACA0015_MB_G/15ms_PLANE_B_PA_300/rear/15ms_PLANE_B_PA_300_000787.T000.D000.P007.H000.L.vec", path "C:/Users/PIV/Documents/mike_ensight/NACA0015_MB_G/15ms_PLANE_B_PA_300/rear/15ms_PLANE_B_PA_300_000788.T000.D000.P007.H000.L.vec", path "C:/Users/PIV/Documents/mike_ensight/NACA0015_MB_G/15ms_PLANE_B_PA_300/rear/15ms_PLANE_B_PA_300_000789.T000.D000.P007.H000.L.vec", path "C:/Users/PIV/Documents/mike_ensight/NACA0015_MB_G/15ms_PLANE_B_PA_300/rear/15ms_PLANE_B_PA_300_000790.T000.D000.P007.H000.L.vec", path "C:/Users/PIV/Documents/mike_ensight/NACA0015_MB_G/15ms_PLANE_B_PA_300/rear/15ms_PLANE_B_PA_300_000791.T000.D000.P007.H000.L.vec", path "C:/Users/PIV/Documents/mike_ensight/NACA0015_MB_G/15ms_PLANE_B_PA_300/rear/15ms_PLANE_B_PA_300_000792.T000.D000.P007.H000.L.vec", path "C:/Users/PIV/Documents/mike_ensight/NACA0015_MB_G/15ms_PLANE_B_PA_300/rear/15ms_PLANE_B_PA_300_000793.T000.D000.P007.H000.L.vec", path "C:/Users/PIV/Documents/mike_ensight/NACA0015_MB_G/15ms_PLANE_B_PA_300/rear/15ms_PLANE_B_PA_300_000794.T000.D000.P007.H000.L.vec", path "C:/Users/PIV/Documents/mike_ensight/NACA0015_MB_G/15ms_PLANE_B_PA_300/rear/15ms_PLANE_B_PA_300_000795.T000.D000.P007.H000.L.vec", path "C:/Users/PIV/Documents/mike_ensight/NACA0015_MB_G/15ms_PLANE_B_PA_300/rear/15ms_PLANE_B_PA_300_000796.T000.D000.P007.H000.L.vec", path "C:/Users/PIV/Documents/mike_ensight/NACA0015_MB_G/15ms_PLANE_B_PA_300/rear/15ms_PLANE_B_PA_300_000797.T000.D000.P007.H000.L.vec", path "C:/Users/PIV/Documents/mike_ensight/NACA0015_MB_G/15ms_PLANE_B_PA_300/rear/15ms_PLANE_B_PA_300_000798.T000.D000.P007.H000.L.vec", path "C:/Users/PIV/Documents/mike_ensight/NACA0015_MB_G/15ms_PLANE_B_PA_300/rear/15ms_PLANE_B_PA_300_000799.T000.D000.P007.H000.L.vec", path "C:/Users/PIV/Documents/mike_ensight/NACA0015_MB_G/15ms_PLANE_B_PA_300/rear/15ms_PLANE_B_PA_300_000800.T000.D000.P007.H000.L.vec", path "C:/Users/PIV/Documents/mike_ensight/NACA0015_MB_G/15ms_PLANE_B_PA_300/rear/15ms_PLANE_B_PA_300_000801.T000.D000.P007.H000.L.vec", path "C:/Users/PIV/Documents/mike_ensight/NACA0015_MB_G/15ms_PLANE_B_PA_300/rear/15ms_PLANE_B_PA_300_000802.T000.D000.P007.H000.L.vec", path "C:/Users/PIV/Documents/mike_ensight/NACA0015_MB_G/15ms_PLANE_B_PA_300/rear/15ms_PLANE_B_PA_300_000803.T000.D000.P007.H000.L.vec", path "C:/Users/PIV/Documents/mike_ensight/NACA0015_MB_G/15ms_PLANE_B_PA_300/rear/15ms_PLANE_B_PA_300_000804.T000.D000.P007.H000.L.vec", path "C:/Users/PIV/Documents/mike_ensight/NACA0015_MB_G/15ms_PLANE_B_PA_300/rear/15ms_PLANE_B_PA_300_000805.T000.D000.P007.H000.L.vec", path "C:/Users/PIV/Documents/mike_ensight/NACA0015_MB_G/15ms_PLANE_B_PA_300/rear/15ms_PLANE_B_PA_300_000806.T000.D000.P007.H000.L.vec", path "C:/Users/PIV/Documents/mike_ensight/NACA0015_MB_G/15ms_PLANE_B_PA_300/rear/15ms_PLANE_B_PA_300_000807.T000.D000.P007.H000.L.vec", path "C:/Users/PIV/Documents/mike_ensight/NACA0015_MB_G/15ms_PLANE_B_PA_300/rear/15ms_PLANE_B_PA_300_000808.T000.D000.P007.H000.L.vec", path "C:/Users/PIV/Documents/mike_ensight/NACA0015_MB_G/15ms_PLANE_B_PA_300/rear/15ms_PLANE_B_PA_300_000809.T000.D000.P007.H000.L.vec", path "C:/Users/PIV/Documents/mike_ensight/NACA0015_MB_G/15ms_PLANE_B_PA_300/rear/15ms_PLANE_B_PA_300_000810.T000.D000.P007.H000.L.vec", path "C:/Users/PIV/Documents/mike_ensight/NACA0015_MB_G/15ms_PLANE_B_PA_300/rear/15ms_PLANE_B_PA_300_000811.T000.D000.P007.H000.L.vec", path "C:/Users/PIV/Documents/mike_ensight/NACA0015_MB_G/15ms_PLANE_B_PA_300/rear/15ms_PLANE_B_PA_300_000812.T000.D000.P007.H000.L.vec", path "C:/Users/PIV/Documents/mike_ensight/NACA0015_MB_G/15ms_PLANE_B_PA_300/rear/15ms_PLANE_B_PA_300_000813.T000.D000.P007.H000.L.vec", path "C:/Users/PIV/Documents/mike_ensight/NACA0015_MB_G/15ms_PLANE_B_PA_300/rear/15ms_PLANE_B_PA_300_000814.T000.D000.P007.H000.L.vec", path "C:/Users/PIV/Documents/mike_ensight/NACA0015_MB_G/15ms_PLANE_B_PA_300/rear/15ms_PLANE_B_PA_300_000815.T000.D000.P007.H000.L.vec", path "C:/Users/PIV/Documents/mike_ensight/NACA0015_MB_G/15ms_PLANE_B_PA_300/rear/15ms_PLANE_B_PA_300_000816.T000.D000.P007.H000.L.vec", path "C:/Users/PIV/Documents/mike_ensight/NACA0015_MB_G/15ms_PLANE_B_PA_300/rear/15ms_PLANE_B_PA_300_000817.T000.D000.P007.H000.L.vec", path "C:/Users/PIV/Documents/mike_ensight/NACA0015_MB_G/15ms_PLANE_B_PA_300/rear/15ms_PLANE_B_PA_300_000818.T000.D000.P007.H000.L.vec", path "C:/Users/PIV/Documents/mike_ensight/NACA0015_MB_G/15ms_PLANE_B_PA_300/rear/15ms_PLANE_B_PA_300_000819.T000.D000.P007.H000.L.vec", path "C:/Users/PIV/Documents/mike_ensight/NACA0015_MB_G/15ms_PLANE_B_PA_300/rear/15ms_PLANE_B_PA_300_000820.T000.D000.P007.H000.L.vec", path "C:/Users/PIV/Documents/mike_ensight/NACA0015_MB_G/15ms_PLANE_B_PA_300/rear/15ms_PLANE_B_PA_300_000821.T000.D000.P007.H000.L.vec", path "C:/Users/PIV/Documents/mike_ensight/NACA0015_MB_G/15ms_PLANE_B_PA_300/rear/15ms_PLANE_B_PA_300_000822.T000.D000.P007.H000.L.vec", path "C:/Users/PIV/Documents/mike_ensight/NACA0015_MB_G/15ms_PLANE_B_PA_300/rear/15ms_PLANE_B_PA_300_000823.T000.D000.P007.H000.L.vec", path "C:/Users/PIV/Documents/mike_ensight/NACA0015_MB_G/15ms_PLANE_B_PA_300/rear/15ms_PLANE_B_PA_300_000824.T000.D000.P007.H000.L.vec", path "C:/Users/PIV/Documents/mike_ensight/NACA0015_MB_G/15ms_PLANE_B_PA_300/rear/15ms_PLANE_B_PA_300_000825.T000.D000.P007.H000.L.vec", path "C:/Users/PIV/Documents/mike_ensight/NACA0015_MB_G/15ms_PLANE_B_PA_300/rear/15ms_PLANE_B_PA_300_000826.T000.D000.P007.H000.L.vec", path "C:/Users/PIV/Documents/mike_ensight/NACA0015_MB_G/15ms_PLANE_B_PA_300/rear/15ms_PLANE_B_PA_300_000827.T000.D000.P007.H000.L.vec", path "C:/Users/PIV/Documents/mike_ensight/NACA0015_MB_G/15ms_PLANE_B_PA_300/rear/15ms_PLANE_B_PA_300_000828.T000.D000.P007.H000.L.vec", path "C:/Users/PIV/Documents/mike_ensight/NACA0015_MB_G/15ms_PLANE_B_PA_300/rear/15ms_PLANE_B_PA_300_000829.T000.D000.P007.H000.L.vec", path "C:/Users/PIV/Documents/mike_ensight/NACA0015_MB_G/15ms_PLANE_B_PA_300/rear/15ms_PLANE_B_PA_300_000830.T000.D000.P007.H000.L.vec", path "C:/Users/PIV/Documents/mike_ensight/NACA0015_MB_G/15ms_PLANE_B_PA_300/rear/15ms_PLANE_B_PA_300_000831.T000.D000.P007.H000.L.vec", path "C:/Users/PIV/Documents/mike_ensight/NACA0015_MB_G/15ms_PLANE_B_PA_300/rear/15ms_PLANE_B_PA_300_000832.T000.D000.P007.H000.L.vec", path "C:/Users/PIV/Documents/mike_ensight/NACA0015_MB_G/15ms_PLANE_B_PA_300/rear/15ms_PLANE_B_PA_300_000833.T000.D000.P007.H000.L.vec", path "C:/Users/PIV/Documents/mike_ensight/NACA0015_MB_G/15ms_PLANE_B_PA_300/rear/15ms_PLANE_B_PA_300_000834.T000.D000.P007.H000.L.vec", path "C:/Users/PIV/Documents/mike_ensight/NACA0015_MB_G/15ms_PLANE_B_PA_300/rear/15ms_PLANE_B_PA_300_000835.T000.D000.P007.H000.L.vec", path "C:/Users/PIV/Documents/mike_ensight/NACA0015_MB_G/15ms_PLANE_B_PA_300/rear/15ms_PLANE_B_PA_300_000836.T000.D000.P007.H000.L.vec", path "C:/Users/PIV/Documents/mike_ensight/NACA0015_MB_G/15ms_PLANE_B_PA_300/rear/15ms_PLANE_B_PA_300_000837.T000.D000.P007.H000.L.vec", path "C:/Users/PIV/Documents/mike_ensight/NACA0015_MB_G/15ms_PLANE_B_PA_300/rear/15ms_PLANE_B_PA_300_000838.T000.D000.P007.H000.L.vec", path "C:/Users/PIV/Documents/mike_ensight/NACA0015_MB_G/15ms_PLANE_B_PA_300/rear/15ms_PLANE_B_PA_300_000839.T000.D000.P007.H000.L.vec", path "C:/Users/PIV/Documents/mike_ensight/NACA0015_MB_G/15ms_PLANE_B_PA_300/rear/15ms_PLANE_B_PA_300_000840.T000.D000.P007.H000.L.vec", path "C:/Users/PIV/Documents/mike_ensight/NACA0015_MB_G/15ms_PLANE_B_PA_300/rear/15ms_PLANE_B_PA_300_000841.T000.D000.P007.H000.L.vec", path "C:/Users/PIV/Documents/mike_ensight/NACA0015_MB_G/15ms_PLANE_B_PA_300/rear/15ms_PLANE_B_PA_300_000842.T000.D000.P007.H000.L.vec", path "C:/Users/PIV/Documents/mike_ensight/NACA0015_MB_G/15ms_PLANE_B_PA_300/rear/15ms_PLANE_B_PA_300_000843.T000.D000.P007.H000.L.vec", path "C:/Users/PIV/Documents/mike_ensight/NACA0015_MB_G/15ms_PLANE_B_PA_300/rear/15ms_PLANE_B_PA_300_000844.T000.D000.P007.H000.L.vec", path "C:/Users/PIV/Documents/mike_ensight/NACA0015_MB_G/15ms_PLANE_B_PA_300/rear/15ms_PLANE_B_PA_300_000845.T000.D000.P007.H000.L.vec", path "C:/Users/PIV/Documents/mike_ensight/NACA0015_MB_G/15ms_PLANE_B_PA_300/rear/15ms_PLANE_B_PA_300_000846.T000.D000.P007.H000.L.vec", path "C:/Users/PIV/Documents/mike_ensight/NACA0015_MB_G/15ms_PLANE_B_PA_300/rear/15ms_PLANE_B_PA_300_000847.T000.D000.P007.H000.L.vec", path "C:/Users/PIV/Documents/mike_ensight/NACA0015_MB_G/15ms_PLANE_B_PA_300/rear/15ms_PLANE_B_PA_300_000848.T000.D000.P007.H000.L.vec", path "C:/Users/PIV/Documents/mike_ensight/NACA0015_MB_G/15ms_PLANE_B_PA_300/rear/15ms_PLANE_B_PA_300_000849.T000.D000.P007.H000.L.vec", path "C:/Users/PIV/Documents/mike_ensight/NACA0015_MB_G/15ms_PLANE_B_PA_300/rear/15ms_PLANE_B_PA_300_000850.T000.D000.P007.H000.L.vec", path "C:/Users/PIV/Documents/mike_ensight/NACA0015_MB_G/15ms_PLANE_B_PA_300/rear/15ms_PLANE_B_PA_300_000851.T000.D000.P007.H000.L.vec", path "C:/Users/PIV/Documents/mike_ensight/NACA0015_MB_G/15ms_PLANE_B_PA_300/rear/15ms_PLANE_B_PA_300_000852.T000.D000.P007.H000.L.vec", path "C:/Users/PIV/Documents/mike_ensight/NACA0015_MB_G/15ms_PLANE_B_PA_300/rear/15ms_PLANE_B_PA_300_000853.T000.D000.P007.H000.L.vec", path "C:/Users/PIV/Documents/mike_ensight/NACA0015_MB_G/15ms_PLANE_B_PA_300/rear/15ms_PLANE_B_PA_300_000854.T000.D000.P007.H000.L.vec", path "C:/Users/PIV/Documents/mike_ensight/NACA0015_MB_G/15ms_PLANE_B_PA_300/rear/15ms_PLANE_B_PA_300_000855.T000.D000.P007.H000.L.vec", path "C:/Users/PIV/Documents/mike_ensight/NACA0015_MB_G/15ms_PLANE_B_PA_300/rear/15ms_PLANE_B_PA_300_000856.T000.D000.P007.H000.L.vec", path "C:/Users/PIV/Documents/mike_ensight/NACA0015_MB_G/15ms_PLANE_B_PA_300/rear/15ms_PLANE_B_PA_300_000857.T000.D000.P007.H000.L.vec", path "C:/Users/PIV/Documents/mike_ensight/NACA0015_MB_G/15ms_PLANE_B_PA_300/rear/15ms_PLANE_B_PA_300_000858.T000.D000.P007.H000.L.vec", path "C:/Users/PIV/Documents/mike_ensight/NACA0015_MB_G/15ms_PLANE_B_PA_300/rear/15ms_PLANE_B_PA_300_000859.T000.D000.P007.H000.L.vec", path "C:/Users/PIV/Documents/mike_ensight/NACA0015_MB_G/15ms_PLANE_B_PA_300/rear/15ms_PLANE_B_PA_300_000860.T000.D000.P007.H000.L.vec", path "C:/Users/PIV/Documents/mike_ensight/NACA0015_MB_G/15ms_PLANE_B_PA_300/rear/15ms_PLANE_B_PA_300_000861.T000.D000.P007.H000.L.vec", path "C:/Users/PIV/Documents/mike_ensight/NACA0015_MB_G/15ms_PLANE_B_PA_300/rear/15ms_PLANE_B_PA_300_000862.T000.D000.P007.H000.L.vec", path "C:/Users/PIV/Documents/mike_ensight/NACA0015_MB_G/15ms_PLANE_B_PA_300/rear/15ms_PLANE_B_PA_300_000863.T000.D000.P007.H000.L.vec", path "C:/Users/PIV/Documents/mike_ensight/NACA0015_MB_G/15ms_PLANE_B_PA_300/rear/15ms_PLANE_B_PA_300_000864.T000.D000.P007.H000.L.vec", path "C:/Users/PIV/Documents/mike_ensight/NACA0015_MB_G/15ms_PLANE_B_PA_300/rear/15ms_PLANE_B_PA_300_000865.T000.D000.P007.H000.L.vec", path "C:/Users/PIV/Documents/mike_ensight/NACA0015_MB_G/15ms_PLANE_B_PA_300/rear/15ms_PLANE_B_PA_300_000866.T000.D000.P007.H000.L.vec", path "C:/Users/PIV/Documents/mike_ensight/NACA0015_MB_G/15ms_PLANE_B_PA_300/rear/15ms_PLANE_B_PA_300_000867.T000.D000.P007.H000.L.vec", path "C:/Users/PIV/Documents/mike_ensight/NACA0015_MB_G/15ms_PLANE_B_PA_300/rear/15ms_PLANE_B_PA_300_000868.T000.D000.P007.H000.L.vec", path "C:/Users/PIV/Documents/mike_ensight/NACA0015_MB_G/15ms_PLANE_B_PA_300/rear/15ms_PLANE_B_PA_300_000869.T000.D000.P007.H000.L.vec", path "C:/Users/PIV/Documents/mike_ensight/NACA0015_MB_G/15ms_PLANE_B_PA_300/rear/15ms_PLANE_B_PA_300_000870.T000.D000.P007.H000.L.vec", path "C:/Users/PIV/Documents/mike_ensight/NACA0015_MB_G/15ms_PLANE_B_PA_300/rear/15ms_PLANE_B_PA_300_000871.T000.D000.P007.H000.L.vec", path "C:/Users/PIV/Documents/mike_ensight/NACA0015_MB_G/15ms_PLANE_B_PA_300/rear/15ms_PLANE_B_PA_300_000872.T000.D000.P007.H000.L.vec", path "C:/Users/PIV/Documents/mike_ensight/NACA0015_MB_G/15ms_PLANE_B_PA_300/rear/15ms_PLANE_B_PA_300_000873.T000.D000.P007.H000.L.vec", path "C:/Users/PIV/Documents/mike_ensight/NACA0015_MB_G/15ms_PLANE_B_PA_300/rear/15ms_PLANE_B_PA_300_000874.T000.D000.P007.H000.L.vec", path "C:/Users/PIV/Documents/mike_ensight/NACA0015_MB_G/15ms_PLANE_B_PA_300/rear/15ms_PLANE_B_PA_300_000875.T000.D000.P007.H000.L.vec", path "C:/Users/PIV/Documents/mike_ensight/NACA0015_MB_G/15ms_PLANE_B_PA_300/rear/15ms_PLANE_B_PA_300_000876.T000.D000.P007.H000.L.vec", path "C:/Users/PIV/Documents/mike_ensight/NACA0015_MB_G/15ms_PLANE_B_PA_300/rear/15ms_PLANE_B_PA_300_000877.T000.D000.P007.H000.L.vec", path "C:/Users/PIV/Documents/mike_ensight/NACA0015_MB_G/15ms_PLANE_B_PA_300/rear/15ms_PLANE_B_PA_300_000878.T000.D000.P007.H000.L.vec", path "C:/Users/PIV/Documents/mike_ensight/NACA0015_MB_G/15ms_PLANE_B_PA_300/rear/15ms_PLANE_B_PA_300_000879.T000.D000.P007.H000.L.vec", path "C:/Users/PIV/Documents/mike_ensight/NACA0015_MB_G/15ms_PLANE_B_PA_300/rear/15ms_PLANE_B_PA_300_000880.T000.D000.P007.H000.L.vec", path "C:/Users/PIV/Documents/mike_ensight/NACA0015_MB_G/15ms_PLANE_B_PA_300/rear/15ms_PLANE_B_PA_300_000881.T000.D000.P007.H000.L.vec", path "C:/Users/PIV/Documents/mike_ensight/NACA0015_MB_G/15ms_PLANE_B_PA_300/rear/15ms_PLANE_B_PA_300_000882.T000.D000.P007.H000.L.vec", path "C:/Users/PIV/Documents/mike_ensight/NACA0015_MB_G/15ms_PLANE_B_PA_300/rear/15ms_PLANE_B_PA_300_000883.T000.D000.P007.H000.L.vec", path "C:/Users/PIV/Documents/mike_ensight/NACA0015_MB_G/15ms_PLANE_B_PA_300/rear/15ms_PLANE_B_PA_300_000884.T000.D000.P007.H000.L.vec", path "C:/Users/PIV/Documents/mike_ensight/NACA0015_MB_G/15ms_PLANE_B_PA_300/rear/15ms_PLANE_B_PA_300_000885.T000.D000.P007.H000.L.vec", path "C:/Users/PIV/Documents/mike_ensight/NACA0015_MB_G/15ms_PLANE_B_PA_300/rear/15ms_PLANE_B_PA_300_000886.T000.D000.P007.H000.L.vec", path "C:/Users/PIV/Documents/mike_ensight/NACA0015_MB_G/15ms_PLANE_B_PA_300/rear/15ms_PLANE_B_PA_300_000887.T000.D000.P007.H000.L.vec", path "C:/Users/PIV/Documents/mike_ensight/NACA0015_MB_G/15ms_PLANE_B_PA_300/rear/15ms_PLANE_B_PA_300_000888.T000.D000.P007.H000.L.vec", path "C:/Users/PIV/Documents/mike_ensight/NACA0015_MB_G/15ms_PLANE_B_PA_300/rear/15ms_PLANE_B_PA_300_000889.T000.D000.P007.H000.L.vec", path "C:/Users/PIV/Documents/mike_ensight/NACA0015_MB_G/15ms_PLANE_B_PA_300/rear/15ms_PLANE_B_PA_300_000890.T000.D000.P007.H000.L.vec", path "C:/Users/PIV/Documents/mike_ensight/NACA0015_MB_G/15ms_PLANE_B_PA_300/rear/15ms_PLANE_B_PA_300_000891.T000.D000.P007.H000.L.vec", path "C:/Users/PIV/Documents/mike_ensight/NACA0015_MB_G/15ms_PLANE_B_PA_300/rear/15ms_PLANE_B_PA_300_000892.T000.D000.P007.H000.L.vec", path "C:/Users/PIV/Documents/mike_ensight/NACA0015_MB_G/15ms_PLANE_B_PA_300/rear/15ms_PLANE_B_PA_300_000893.T000.D000.P007.H000.L.vec", path "C:/Users/PIV/Documents/mike_ensight/NACA0015_MB_G/15ms_PLANE_B_PA_300/rear/15ms_PLANE_B_PA_300_000894.T000.D000.P007.H000.L.vec", path "C:/Users/PIV/Documents/mike_ensight/NACA0015_MB_G/15ms_PLANE_B_PA_300/rear/15ms_PLANE_B_PA_300_000895.T000.D000.P007.H000.L.vec", path "C:/Users/PIV/Documents/mike_ensight/NACA0015_MB_G/15ms_PLANE_B_PA_300/rear/15ms_PLANE_B_PA_300_000896.T000.D000.P007.H000.L.vec", path "C:/Users/PIV/Documents/mike_ensight/NACA0015_MB_G/15ms_PLANE_B_PA_300/rear/15ms_PLANE_B_PA_300_000897.T000.D000.P007.H000.L.vec", path "C:/Users/PIV/Documents/mike_ensight/NACA0015_MB_G/15ms_PLANE_B_PA_300/rear/15ms_PLANE_B_PA_300_000898.T000.D000.P007.H000.L.vec", path "C:/Users/PIV/Documents/mike_ensight/NACA0015_MB_G/15ms_PLANE_B_PA_300/rear/15ms_PLANE_B_PA_300_000899.T000.D000.P007.H000.L.vec", path "C:/Users/PIV/Documents/mike_ensight/NACA0015_MB_G/15ms_PLANE_B_PA_300/rear/15ms_PLANE_B_PA_300_000900.T000.D000.P007.H000.L.vec", path "C:/Users/PIV/Documents/mike_ensight/NACA0015_MB_G/15ms_PLANE_B_PA_300/rear/15ms_PLANE_B_PA_300_000901.T000.D000.P007.H000.L.vec", path "C:/Users/PIV/Documents/mike_ensight/NACA0015_MB_G/15ms_PLANE_B_PA_300/rear/15ms_PLANE_B_PA_300_000902.T000.D000.P007.H000.L.vec", path "C:/Users/PIV/Documents/mike_ensight/NACA0015_MB_G/15ms_PLANE_B_PA_300/rear/15ms_PLANE_B_PA_300_000903.T000.D000.P007.H000.L.vec", path "C:/Users/PIV/Documents/mike_ensight/NACA0015_MB_G/15ms_PLANE_B_PA_300/rear/15ms_PLANE_B_PA_300_000904.T000.D000.P007.H000.L.vec", path "C:/Users/PIV/Documents/mike_ensight/NACA0015_MB_G/15ms_PLANE_B_PA_300/rear/15ms_PLANE_B_PA_300_000905.T000.D000.P007.H000.L.vec", path "C:/Users/PIV/Documents/mike_ensight/NACA0015_MB_G/15ms_PLANE_B_PA_300/rear/15ms_PLANE_B_PA_300_000906.T000.D000.P007.H000.L.vec", path "C:/Users/PIV/Documents/mike_ensight/NACA0015_MB_G/15ms_PLANE_B_PA_300/rear/15ms_PLANE_B_PA_300_000907.T000.D000.P007.H000.L.vec", path "C:/Users/PIV/Documents/mike_ensight/NACA0015_MB_G/15ms_PLANE_B_PA_300/rear/15ms_PLANE_B_PA_300_000908.T000.D000.P007.H000.L.vec", path "C:/Users/PIV/Documents/mike_ensight/NACA0015_MB_G/15ms_PLANE_B_PA_300/rear/15ms_PLANE_B_PA_300_000909.T000.D000.P007.H000.L.vec", path "C:/Users/PIV/Documents/mike_ensight/NACA0015_MB_G/15ms_PLANE_B_PA_300/rear/15ms_PLANE_B_PA_300_000910.T000.D000.P007.H000.L.vec", path "C:/Users/PIV/Documents/mike_ensight/NACA0015_MB_G/15ms_PLANE_B_PA_300/rear/15ms_PLANE_B_PA_300_000911.T000.D000.P007.H000.L.vec", path "C:/Users/PIV/Documents/mike_ensight/NACA0015_MB_G/15ms_PLANE_B_PA_300/rear/15ms_PLANE_B_PA_300_000912.T000.D000.P007.H000.L.vec", path "C:/Users/PIV/Documents/mike_ensight/NACA0015_MB_G/15ms_PLANE_B_PA_300/rear/15ms_PLANE_B_PA_300_000913.T000.D000.P007.H000.L.vec", path "C:/Users/PIV/Documents/mike_ensight/NACA0015_MB_G/15ms_PLANE_B_PA_300/rear/15ms_PLANE_B_PA_300_000914.T000.D000.P007.H000.L.vec", path "C:/Users/PIV/Documents/mike_ensight/NACA0015_MB_G/15ms_PLANE_B_PA_300/rear/15ms_PLANE_B_PA_300_000915.T000.D000.P007.H000.L.vec", path "C:/Users/PIV/Documents/mike_ensight/NACA0015_MB_G/15ms_PLANE_B_PA_300/rear/15ms_PLANE_B_PA_300_000916.T000.D000.P007.H000.L.vec", path "C:/Users/PIV/Documents/mike_ensight/NACA0015_MB_G/15ms_PLANE_B_PA_300/rear/15ms_PLANE_B_PA_300_000917.T000.D000.P007.H000.L.vec", path "C:/Users/PIV/Documents/mike_ensight/NACA0015_MB_G/15ms_PLANE_B_PA_300/rear/15ms_PLANE_B_PA_300_000918.T000.D000.P007.H000.L.vec", path "C:/Users/PIV/Documents/mike_ensight/NACA0015_MB_G/15ms_PLANE_B_PA_300/rear/15ms_PLANE_B_PA_300_000919.T000.D000.P007.H000.L.vec", path "C:/Users/PIV/Documents/mike_ensight/NACA0015_MB_G/15ms_PLANE_B_PA_300/rear/15ms_PLANE_B_PA_300_000920.T000.D000.P007.H000.L.vec", path "C:/Users/PIV/Documents/mike_ensight/NACA0015_MB_G/15ms_PLANE_B_PA_300/rear/15ms_PLANE_B_PA_300_000921.T000.D000.P007.H000.L.vec", path "C:/Users/PIV/Documents/mike_ensight/NACA0015_MB_G/15ms_PLANE_B_PA_300/rear/15ms_PLANE_B_PA_300_000922.T000.D000.P007.H000.L.vec", path "C:/Users/PIV/Documents/mike_ensight/NACA0015_MB_G/15ms_PLANE_B_PA_300/rear/15ms_PLANE_B_PA_300_000923.T000.D000.P007.H000.L.vec", path "C:/Users/PIV/Documents/mike_ensight/NACA0015_MB_G/15ms_PLANE_B_PA_300/rear/15ms_PLANE_B_PA_300_000924.T000.D000.P007.H000.L.vec", path "C:/Users/PIV/Documents/mike_ensight/NACA0015_MB_G/15ms_PLANE_B_PA_300/rear/15ms_PLANE_B_PA_300_000925.T000.D000.P007.H000.L.vec", path "C:/Users/PIV/Documents/mike_ensight/NACA0015_MB_G/15ms_PLANE_B_PA_300/rear/15ms_PLANE_B_PA_300_000926.T000.D000.P007.H000.L.vec", path "C:/Users/PIV/Documents/mike_ensight/NACA0015_MB_G/15ms_PLANE_B_PA_300/rear/15ms_PLANE_B_PA_300_000927.T000.D000.P007.H000.L.vec", path "C:/Users/PIV/Documents/mike_ensight/NACA0015_MB_G/15ms_PLANE_B_PA_300/rear/15ms_PLANE_B_PA_300_000928.T000.D000.P007.H000.L.vec", path "C:/Users/PIV/Documents/mike_ensight/NACA0015_MB_G/15ms_PLANE_B_PA_300/rear/15ms_PLANE_B_PA_300_000929.T000.D000.P007.H000.L.vec", path "C:/Users/PIV/Documents/mike_ensight/NACA0015_MB_G/15ms_PLANE_B_PA_300/rear/15ms_PLANE_B_PA_300_000930.T000.D000.P007.H000.L.vec", path "C:/Users/PIV/Documents/mike_ensight/NACA0015_MB_G/15ms_PLANE_B_PA_300/rear/15ms_PLANE_B_PA_300_000931.T000.D000.P007.H000.L.vec", path "C:/Users/PIV/Documents/mike_ensight/NACA0015_MB_G/15ms_PLANE_B_PA_300/rear/15ms_PLANE_B_PA_300_000932.T000.D000.P007.H000.L.vec", path "C:/Users/PIV/Documents/mike_ensight/NACA0015_MB_G/15ms_PLANE_B_PA_300/rear/15ms_PLANE_B_PA_300_000933.T000.D000.P007.H000.L.vec", path "C:/Users/PIV/Documents/mike_ensight/NACA0015_MB_G/15ms_PLANE_B_PA_300/rear/15ms_PLANE_B_PA_300_000934.T000.D000.P007.H000.L.vec", path "C:/Users/PIV/Documents/mike_ensight/NACA0015_MB_G/15ms_PLANE_B_PA_300/rear/15ms_PLANE_B_PA_300_000935.T000.D000.P007.H000.L.vec", path "C:/Users/PIV/Documents/mike_ensight/NACA0015_MB_G/15ms_PLANE_B_PA_300/rear/15ms_PLANE_B_PA_300_000936.T000.D000.P007.H000.L.vec", path "C:/Users/PIV/Documents/mike_ensight/NACA0015_MB_G/15ms_PLANE_B_PA_300/rear/15ms_PLANE_B_PA_300_000937.T000.D000.P007.H000.L.vec", path "C:/Users/PIV/Documents/mike_ensight/NACA0015_MB_G/15ms_PLANE_B_PA_300/rear/15ms_PLANE_B_PA_300_000938.T000.D000.P007.H000.L.vec", path "C:/Users/PIV/Documents/mike_ensight/NACA0015_MB_G/15ms_PLANE_B_PA_300/rear/15ms_PLANE_B_PA_300_000939.T000.D000.P007.H000.L.vec", path "C:/Users/PIV/Documents/mike_ensight/NACA0015_MB_G/15ms_PLANE_B_PA_300/rear/15ms_PLANE_B_PA_300_000940.T000.D000.P007.H000.L.vec", path "C:/Users/PIV/Documents/mike_ensight/NACA0015_MB_G/15ms_PLANE_B_PA_300/rear/15ms_PLANE_B_PA_300_000941.T000.D000.P007.H000.L.vec", path "C:/Users/PIV/Documents/mike_ensight/NACA0015_MB_G/15ms_PLANE_B_PA_300/rear/15ms_PLANE_B_PA_300_000942.T000.D000.P007.H000.L.vec", path "C:/Users/PIV/Documents/mike_ensight/NACA0015_MB_G/15ms_PLANE_B_PA_300/rear/15ms_PLANE_B_PA_300_000943.T000.D000.P007.H000.L.vec", path "C:/Users/PIV/Documents/mike_ensight/NACA0015_MB_G/15ms_PLANE_B_PA_300/rear/15ms_PLANE_B_PA_300_000944.T000.D000.P007.H000.L.vec", path "C:/Users/PIV/Documents/mike_ensight/NACA0015_MB_G/15ms_PLANE_B_PA_300/rear/15ms_PLANE_B_PA_300_000945.T000.D000.P007.H000.L.vec", path "C:/Users/PIV/Documents/mike_ensight/NACA0015_MB_G/15ms_PLANE_B_PA_300/rear/15ms_PLANE_B_PA_300_000946.T000.D000.P007.H000.L.vec", path "C:/Users/PIV/Documents/mike_ensight/NACA0015_MB_G/15ms_PLANE_B_PA_300/rear/15ms_PLANE_B_PA_300_000947.T000.D000.P007.H000.L.vec", path "C:/Users/PIV/Documents/mike_ensight/NACA0015_MB_G/15ms_PLANE_B_PA_300/rear/15ms_PLANE_B_PA_300_000948.T000.D000.P007.H000.L.vec", path "C:/Users/PIV/Documents/mike_ensight/NACA0015_MB_G/15ms_PLANE_B_PA_300/rear/15ms_PLANE_B_PA_300_000949.T000.D000.P007.H000.L.vec", path "C:/Users/PIV/Documents/mike_ensight/NACA0015_MB_G/15ms_PLANE_B_PA_300/rear/15ms_PLANE_B_PA_300_000950.T000.D000.P007.H000.L.vec", path "C:/Users/PIV/Documents/mike_ensight/NACA0015_MB_G/15ms_PLANE_B_PA_300/rear/15ms_PLANE_B_PA_300_000951.T000.D000.P007.H000.L.vec", path "C:/Users/PIV/Documents/mike_ensight/NACA0015_MB_G/15ms_PLANE_B_PA_300/rear/15ms_PLANE_B_PA_300_000952.T000.D000.P007.H000.L.vec", path "C:/Users/PIV/Documents/mike_ensight/NACA0015_MB_G/15ms_PLANE_B_PA_300/rear/15ms_PLANE_B_PA_300_000953.T000.D000.P007.H000.L.vec", path "C:/Users/PIV/Documents/mike_ensight/NACA0015_MB_G/15ms_PLANE_B_PA_300/rear/15ms_PLANE_B_PA_300_000954.T000.D000.P007.H000.L.vec", path "C:/Users/PIV/Documents/mike_ensight/NACA0015_MB_G/15ms_PLANE_B_PA_300/rear/15ms_PLANE_B_PA_300_000955.T000.D000.P007.H000.L.vec", path "C:/Users/PIV/Documents/mike_ensight/NACA0015_MB_G/15ms_PLANE_B_PA_300/rear/15ms_PLANE_B_PA_300_000956.T000.D000.P007.H000.L.vec", path "C:/Users/PIV/Documents/mike_ensight/NACA0015_MB_G/15ms_PLANE_B_PA_300/rear/15ms_PLANE_B_PA_300_000957.T000.D000.P007.H000.L.vec", path "C:/Users/PIV/Documents/mike_ensight/NACA0015_MB_G/15ms_PLANE_B_PA_300/rear/15ms_PLANE_B_PA_300_000958.T000.D000.P007.H000.L.vec", path "C:/Users/PIV/Documents/mike_ensight/NACA0015_MB_G/15ms_PLANE_B_PA_300/rear/15ms_PLANE_B_PA_300_000959.T000.D000.P007.H000.L.vec", path "C:/Users/PIV/Documents/mike_ensight/NACA0015_MB_G/15ms_PLANE_B_PA_300/rear/15ms_PLANE_B_PA_300_000960.T000.D000.P007.H000.L.vec", path "C:/Users/PIV/Documents/mike_ensight/NACA0015_MB_G/15ms_PLANE_B_PA_300/rear/15ms_PLANE_B_PA_300_000961.T000.D000.P007.H000.L.vec", path "C:/Users/PIV/Documents/mike_ensight/NACA0015_MB_G/15ms_PLANE_B_PA_300/rear/15ms_PLANE_B_PA_300_000962.T000.D000.P007.H000.L.vec", path "C:/Users/PIV/Documents/mike_ensight/NACA0015_MB_G/15ms_PLANE_B_PA_300/rear/15ms_PLANE_B_PA_300_000963.T000.D000.P007.H000.L.vec", path "C:/Users/PIV/Documents/mike_ensight/NACA0015_MB_G/15ms_PLANE_B_PA_300/rear/15ms_PLANE_B_PA_300_000964.T000.D000.P007.H000.L.vec", path "C:/Users/PIV/Documents/mike_ensight/NACA0015_MB_G/15ms_PLANE_B_PA_300/rear/15ms_PLANE_B_PA_300_000965.T000.D000.P007.H000.L.vec", path "C:/Users/PIV/Documents/mike_ensight/NACA0015_MB_G/15ms_PLANE_B_PA_300/rear/15ms_PLANE_B_PA_300_000966.T000.D000.P007.H000.L.vec", path "C:/Users/PIV/Documents/mike_ensight/NACA0015_MB_G/15ms_PLANE_B_PA_300/rear/15ms_PLANE_B_PA_300_000967.T000.D000.P007.H000.L.vec", path "C:/Users/PIV/Documents/mike_ensight/NACA0015_MB_G/15ms_PLANE_B_PA_300/rear/15ms_PLANE_B_PA_300_000968.T000.D000.P007.H000.L.vec", path "C:/Users/PIV/Documents/mike_ensight/NACA0015_MB_G/15ms_PLANE_B_PA_300/rear/15ms_PLANE_B_PA_300_000969.T000.D000.P007.H000.L.vec", path "C:/Users/PIV/Documents/mike_ensight/NACA0015_MB_G/15ms_PLANE_B_PA_300/rear/15ms_PLANE_B_PA_300_000970.T000.D000.P007.H000.L.vec", path "C:/Users/PIV/Documents/mike_ensight/NACA0015_MB_G/15ms_PLANE_B_PA_300/rear/15ms_PLANE_B_PA_300_000971.T000.D000.P007.H000.L.vec", path "C:/Users/PIV/Documents/mike_ensight/NACA0015_MB_G/15ms_PLANE_B_PA_300/rear/15ms_PLANE_B_PA_300_000972.T000.D000.P007.H000.L.vec", path "C:/Users/PIV/Documents/mike_ensight/NACA0015_MB_G/15ms_PLANE_B_PA_300/rear/15ms_PLANE_B_PA_300_000973.T000.D000.P007.H000.L.vec", path "C:/Users/PIV/Documents/mike_ensight/NACA0015_MB_G/15ms_PLANE_B_PA_300/rear/15ms_PLANE_B_PA_300_000974.T000.D000.P007.H000.L.vec", path "C:/Users/PIV/Documents/mike_ensight/NACA0015_MB_G/15ms_PLANE_B_PA_300/rear/15ms_PLANE_B_PA_300_000975.T000.D000.P007.H000.L.vec", path "C:/Users/PIV/Documents/mike_ensight/NACA0015_MB_G/15ms_PLANE_B_PA_300/rear/15ms_PLANE_B_PA_300_000976.T000.D000.P007.H000.L.vec", path "C:/Users/PIV/Documents/mike_ensight/NACA0015_MB_G/15ms_PLANE_B_PA_300/rear/15ms_PLANE_B_PA_300_000977.T000.D000.P007.H000.L.vec", path "C:/Users/PIV/Documents/mike_ensight/NACA0015_MB_G/15ms_PLANE_B_PA_300/rear/15ms_PLANE_B_PA_300_000978.T000.D000.P007.H000.L.vec", path "C:/Users/PIV/Documents/mike_ensight/NACA0015_MB_G/15ms_PLANE_B_PA_300/rear/15ms_PLANE_B_PA_300_000979.T000.D000.P007.H000.L.vec", path "C:/Users/PIV/Documents/mike_ensight/NACA0015_MB_G/15ms_PLANE_B_PA_300/rear/15ms_PLANE_B_PA_300_000980.T000.D000.P007.H000.L.vec", path "C:/Users/PIV/Documents/mike_ensight/NACA0015_MB_G/15ms_PLANE_B_PA_300/rear/15ms_PLANE_B_PA_300_000981.T000.D000.P007.H000.L.vec", path "C:/Users/PIV/Documents/mike_ensight/NACA0015_MB_G/15ms_PLANE_B_PA_300/rear/15ms_PLANE_B_PA_300_000982.T000.D000.P007.H000.L.vec", path "C:/Users/PIV/Documents/mike_ensight/NACA0015_MB_G/15ms_PLANE_B_PA_300/rear/15ms_PLANE_B_PA_300_000983.T000.D000.P007.H000.L.vec", path "C:/Users/PIV/Documents/mike_ensight/NACA0015_MB_G/15ms_PLANE_B_PA_300/rear/15ms_PLANE_B_PA_300_000984.T000.D000.P007.H000.L.vec", path "C:/Users/PIV/Documents/mike_ensight/NACA0015_MB_G/15ms_PLANE_B_PA_300/rear/15ms_PLANE_B_PA_300_000985.T000.D000.P007.H000.L.vec", path "C:/Users/PIV/Documents/mike_ensight/NACA0015_MB_G/15ms_PLANE_B_PA_300/rear/15ms_PLANE_B_PA_300_000986.T000.D000.P007.H000.L.vec", path "C:/Users/PIV/Documents/mike_ensight/NACA0015_MB_G/15ms_PLANE_B_PA_300/rear/15ms_PLANE_B_PA_300_000987.T000.D000.P007.H000.L.vec", path "C:/Users/PIV/Documents/mike_ensight/NACA0015_MB_G/15ms_PLANE_B_PA_300/rear/15ms_PLANE_B_PA_300_000988.T000.D000.P007.H000.L.vec", path "C:/Users/PIV/Documents/mike_ensight/NACA0015_MB_G/15ms_PLANE_B_PA_300/rear/15ms_PLANE_B_PA_300_000989.T000.D000.P007.H000.L.vec", path "C:/Users/PIV/Documents/mike_ensight/NACA0015_MB_G/15ms_PLANE_B_PA_300/rear/15ms_PLANE_B_PA_300_000990.T000.D000.P007.H000.L.vec", path "C:/Users/PIV/Documents/mike_ensight/NACA0015_MB_G/15ms_PLANE_B_PA_300/rear/15ms_PLANE_B_PA_300_000991.T000.D000.P007.H000.L.vec", path "C:/Users/PIV/Documents/mike_ensight/NACA0015_MB_G/15ms_PLANE_B_PA_300/rear/15ms_PLANE_B_PA_300_000992.T000.D000.P007.H000.L.vec", path "C:/Users/PIV/Documents/mike_ensight/NACA0015_MB_G/15ms_PLANE_B_PA_300/rear/15ms_PLANE_B_PA_300_000993.T000.D000.P007.H000.L.vec", path "C:/Users/PIV/Documents/mike_ensight/NACA0015_MB_G/15ms_PLANE_B_PA_300/rear/15ms_PLANE_B_PA_300_000994.T000.D000.P007.H000.L.vec", path "C:/Users/PIV/Documents/mike_ensight/NACA0015_MB_G/15ms_PLANE_B_PA_300/rear/15ms_PLANE_B_PA_300_000995.T000.D000.P007.H000.L.vec", path "C:/Users/PIV/Documents/mike_ensight/NACA0015_MB_G/15ms_PLANE_B_PA_300/rear/15ms_PLANE_B_PA_300_000996.T000.D000.P007.H000.L.vec", path "C:/Users/PIV/Documents/mike_ensight/NACA0015_MB_G/15ms_PLANE_B_PA_300/rear/15ms_PLANE_B_PA_300_000997.T000.D000.P007.H000.L.vec", path "C:/Users/PIV/Documents/mike_ensight/NACA0015_MB_G/15ms_PLANE_B_PA_300/rear/15ms_PLANE_B_PA_300_000998.T000.D000.P007.H000.L.vec", path "C:/Users/PIV/Documents/mike_ensight/NACA0015_MB_G/15ms_PLANE_B_PA_300/rear/15ms_PLANE_B_PA_300_000999.T000.D000.P007.H000.L.vec"]
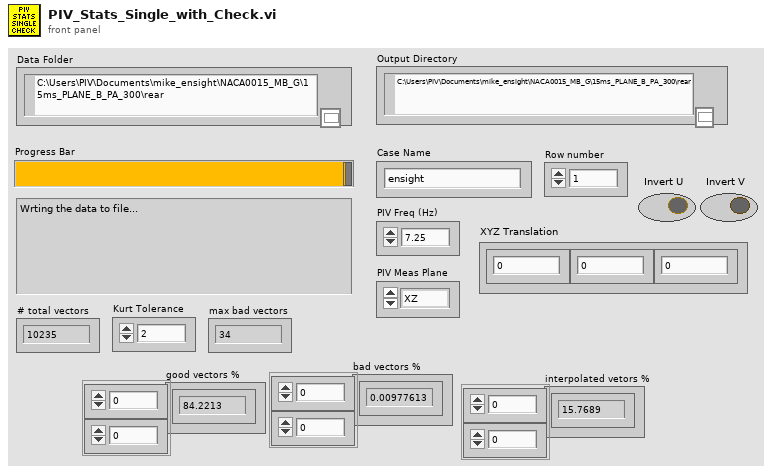
[diagram p1: front panel]
types:
  T1 = cluster{"Record Length":dbl, "CHC":dbl[], "u m/s":dbl[], "v m/s":dbl[], "time s":dbl[], "Vel mag m/s":dbl[], "XYZ Position":dbl[], " Turb Stats":cluster{"U m/s":dbl, "u2 m2/s2":dbl, "u3 m3/s3":dbl, "u4 m4/s4":dbl, "TurbU %":dbl, "Skew_u":dbl, "Kurt_u":dbl, "V m/s":dbl, "v2 m2/s2":dbl, "v3 m3/s3":dbl, "v4 m4/s4":dbl, "TurbV %":dbl, "Skew_v":dbl, "Kurt_v":dbl, "u2v2 m4/s4":dbl, "uv3 m4/s4":dbl, "u3v m4/s4":dbl, "uv2 m3/s3":dbl, "u2v m3/s3":dbl, "uv_cc":dbl, "uv":dbl, "TKE J":dbl}[], "Turb Stats Error":cluster{"U m/s":dbl, "u2 m2/s2":dbl, "u3 m3/s3":dbl, "u4 m4/s4":dbl, "TurbU %":dbl, "Skew_u":dbl, "Kurt_u":dbl, "V m/s":dbl, "v2 m2/s2":dbl, "v3 m3/s3":dbl, "v4 m4/s4":dbl, "TurbV %":dbl, "Skew_v":dbl, "Kurt_v":dbl, "u2v2 m4/s4":dbl, "uv3 m4/s4":dbl, "u3v m4/s4":dbl, "uv2 m3/s3":dbl, "u2v m3/s3":dbl, "uv_cc":dbl, "uv":dbl, "TKE J":dbl}[], "u (good)":dbl[], "v (good)":dbl[]}
  T2 = cluster{"Record Length":dbl, "CHC":dbl[], "u m/s":dbl[], "v m/s":dbl[], "time s":dbl[], "Vel mag m/s":dbl[], "XYZ Position":dbl[], " Turb Stats":cluster{"U m/s":dbl, "u2 m2/s2":dbl, "u3 m3/s3":dbl, "u4 m4/s4":dbl, "TurbU %":dbl, "Skew_u":dbl, "Kurt_u":dbl, "V m/s":dbl, "v2 m2/s2":dbl, "v3 m3/s3":dbl, "v4 m4/s4":dbl, "TurbV %":dbl, "Skew_v":dbl, "Kurt_v":dbl, "u2v2 m4/s4":dbl, "uv3 m4/s4":dbl, "u3v m4/s4":dbl, "uv2 m3/s3":dbl, "u2v m3/s3":dbl, "uv_cc":dbl, "uv":dbl, "TKE J":dbl}[], "Turb Stats Error":cluster{"U m/s":dbl, "u2 m2/s2":dbl, "u3 m3/s3":dbl, "u4 m4/s4":dbl, "TurbU %":dbl, "Skew_u":dbl, "Kurt_u":dbl, "V m/s":dbl, "v2 m2/s2":dbl, "v3 m3/s3":dbl, "v4 m4/s4":dbl, "TurbV %":dbl, "Skew_v":dbl, "Kurt_v":dbl, "u2v2 m4/s4":dbl, "uv3 m4/s4":dbl, "u3v m4/s4":dbl, "uv2 m3/s3":dbl, "u2v m3/s3":dbl, "uv_cc":dbl, "uv":dbl, "TKE J":dbl}[], "u (good)":dbl[], "v (good)":dbl[]}[]
  T3 = cluster{"U m/s":dbl, "u2 m2/s2":dbl, "u3 m3/s3":dbl, "u4 m4/s4":dbl, "TurbU %":dbl, "Skew_u":dbl, "Kurt_u":dbl, "V m/s":dbl, "v2 m2/s2":dbl, "v3 m3/s3":dbl, "v4 m4/s4":dbl, "TurbV %":dbl, "Skew_v":dbl, "Kurt_v":dbl, "u2v2 m4/s4":dbl, "uv3 m4/s4":dbl, "u3v m4/s4":dbl, "uv2 m3/s3":dbl, "u2v m3/s3":dbl, "uv_cc":dbl, "uv":dbl, "TKE J":dbl}
  T4 = cluster{"U m/s":dbl, "u2 m2/s2":dbl, "u3 m3/s3":dbl, "u4 m4/s4":dbl, "TurbU %":dbl, "Skew_u":dbl, "Kurt_u":dbl, "V m/s":dbl, "v2 m2/s2":dbl, "v3 m3/s3":dbl, "v4 m4/s4":dbl, "TurbV %":dbl, "Skew_v":dbl, "Kurt_v":dbl, "u2v2 m4/s4":dbl, "uv3 m4/s4":dbl, "u3v m4/s4":dbl, "uv2 m3/s3":dbl, "u2v m3/s3":dbl, "uv_cc":dbl, "uv":dbl, "TKE J":dbl}[]
  T5 = typedef "DialogType.ctl" = u16
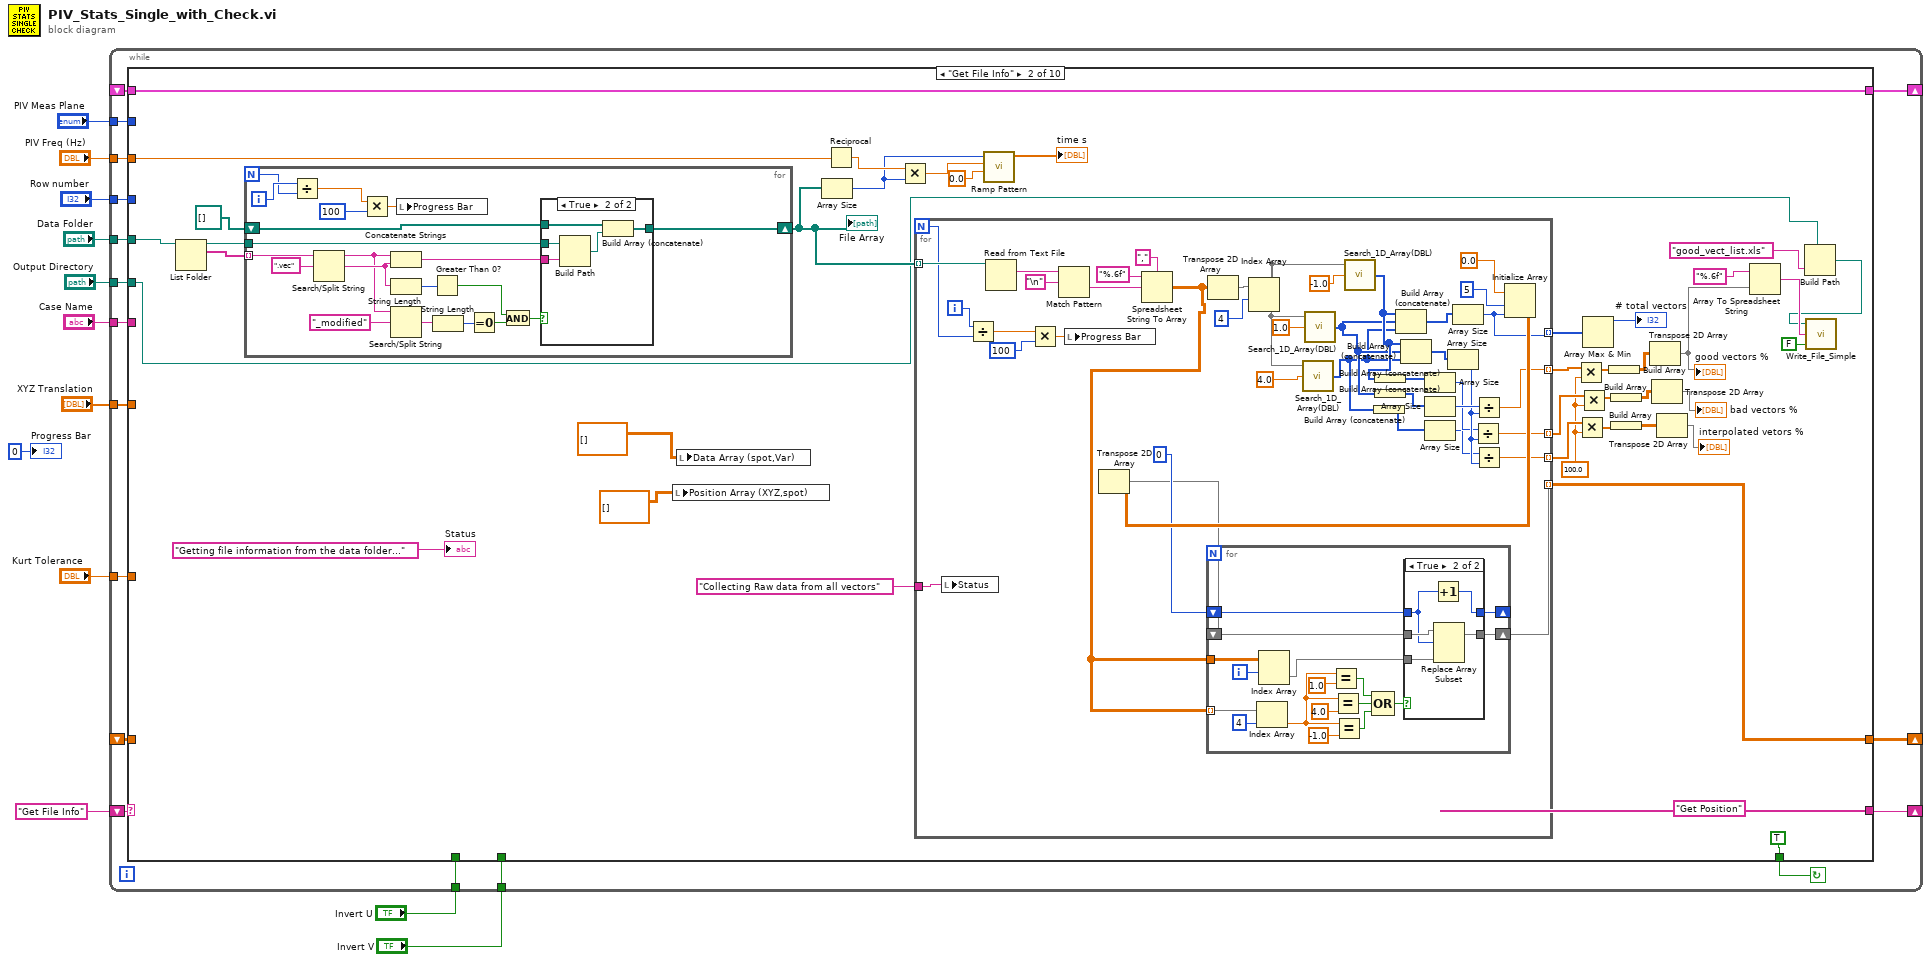
[diagram p0: block diagram]
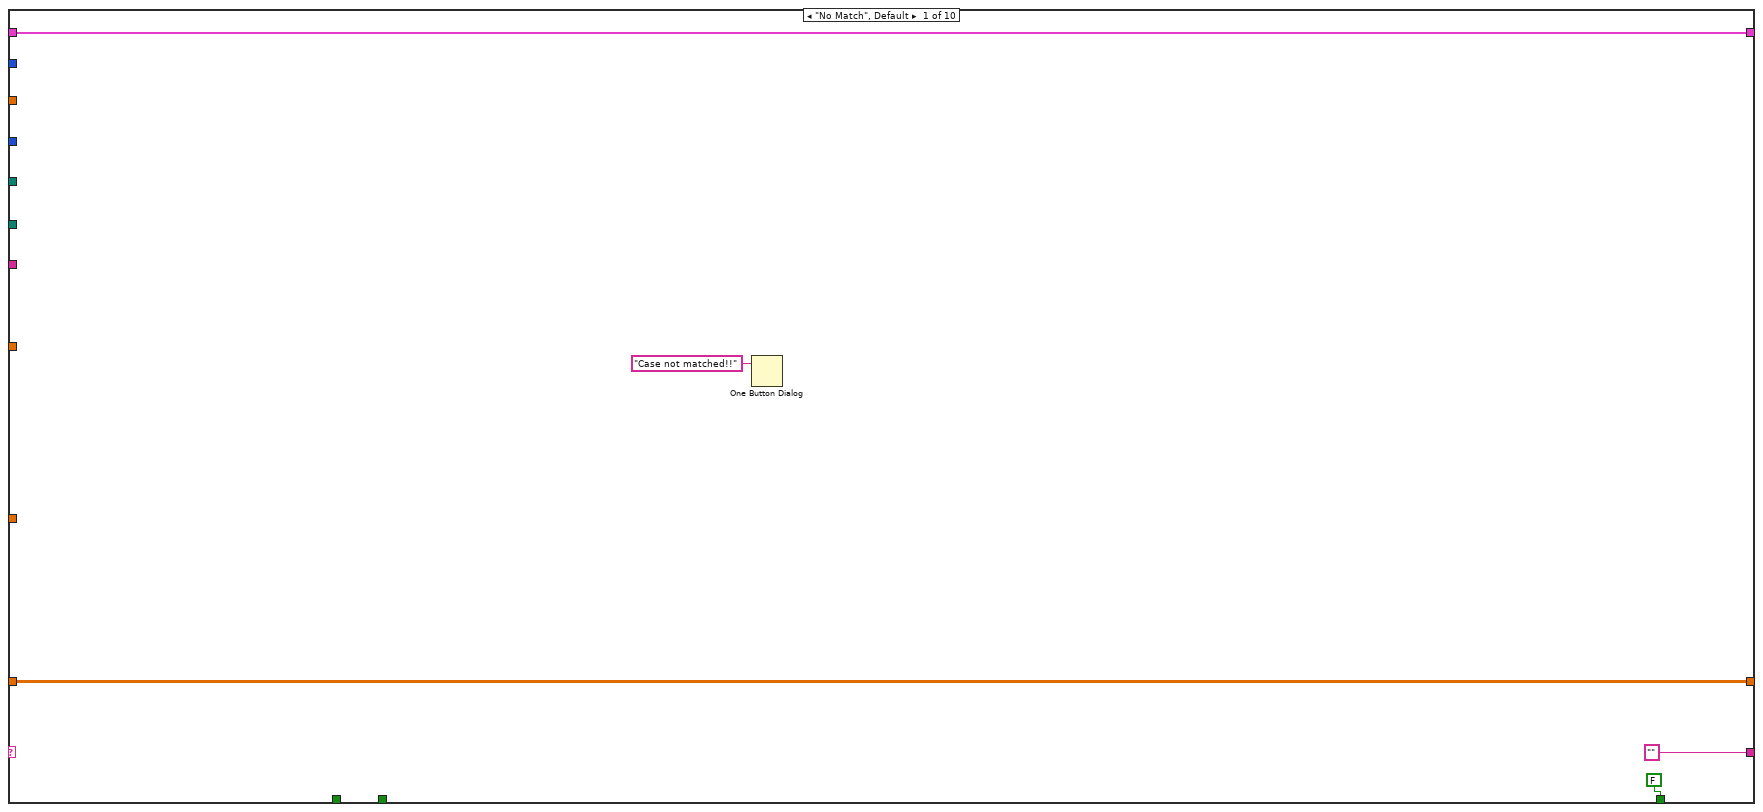
[diagram p2: hidden frame]
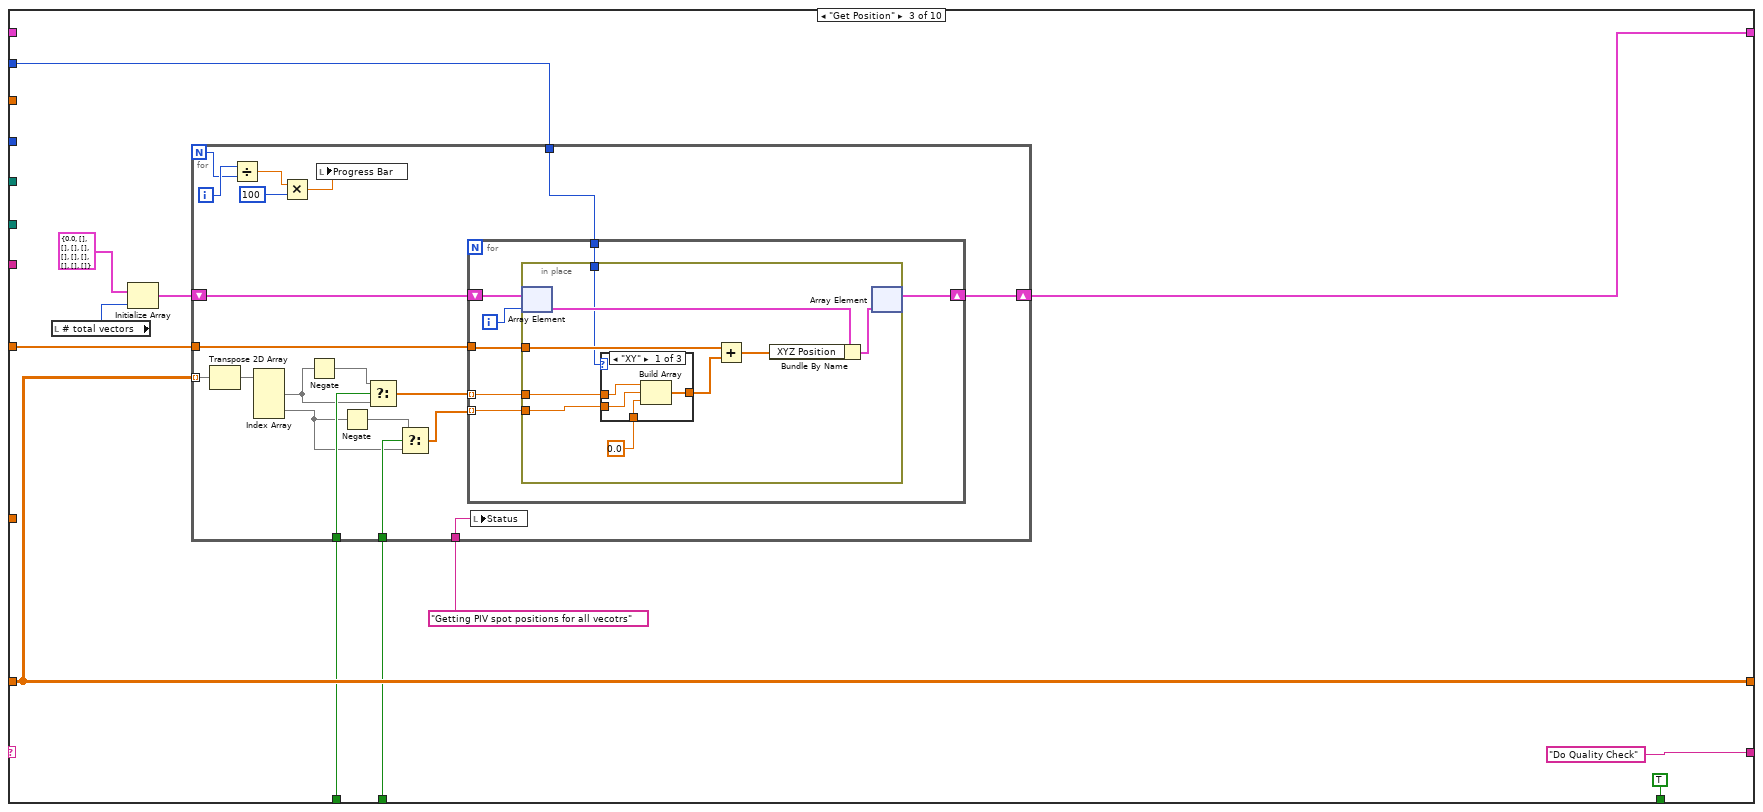
[diagram p5: hidden frame]
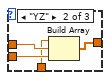
[diagram p6: hidden frame]
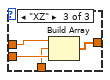
[diagram p7: hidden frame]
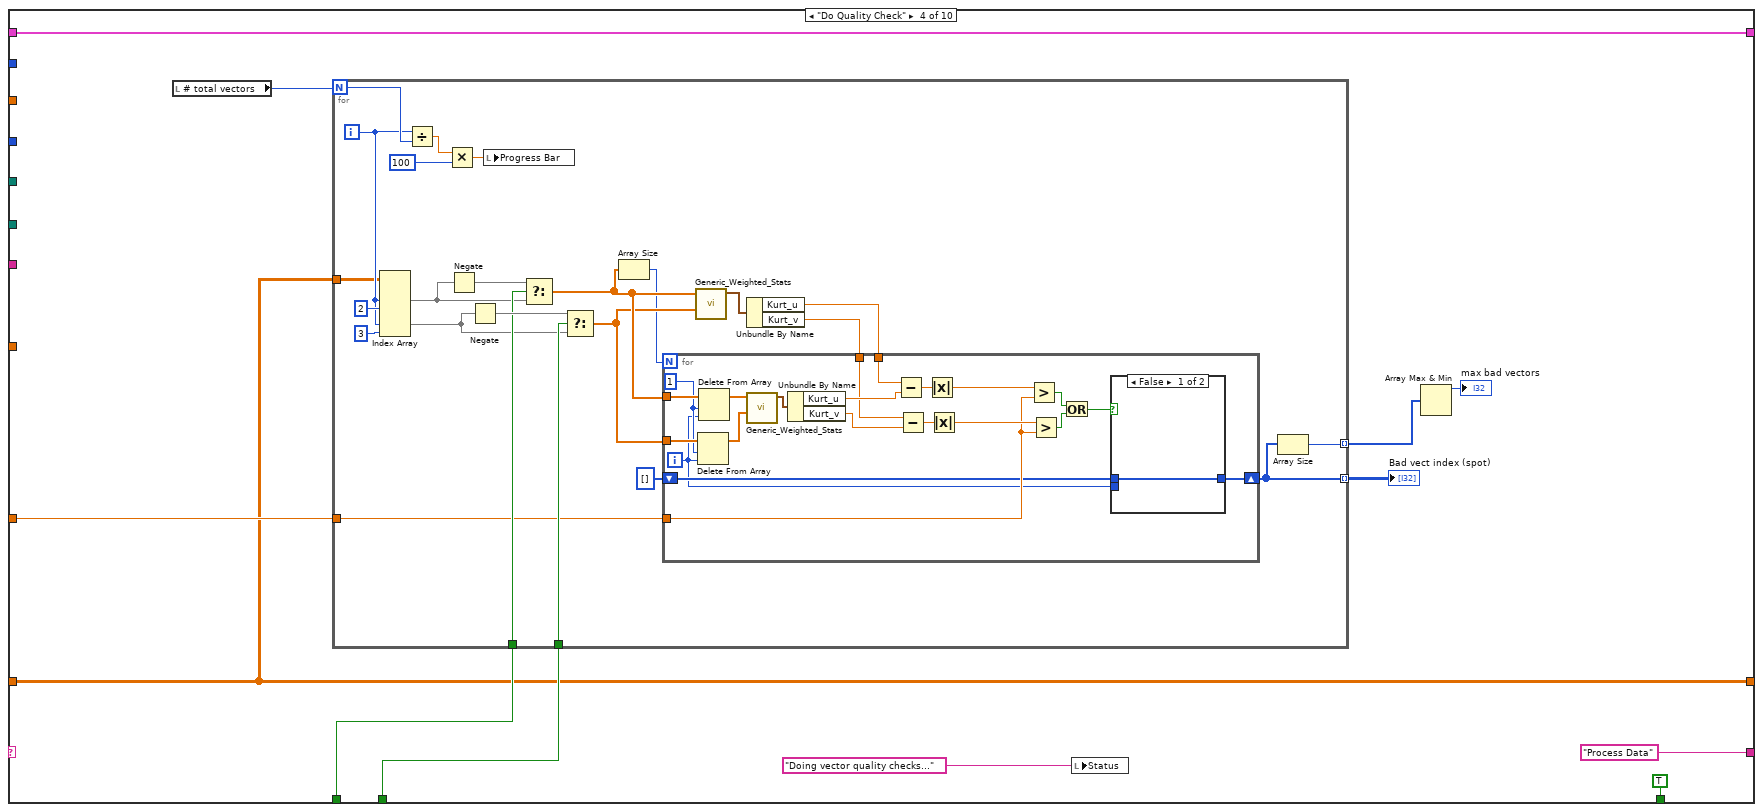
[diagram p8: hidden frame]
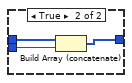
[diagram p9: hidden frame]
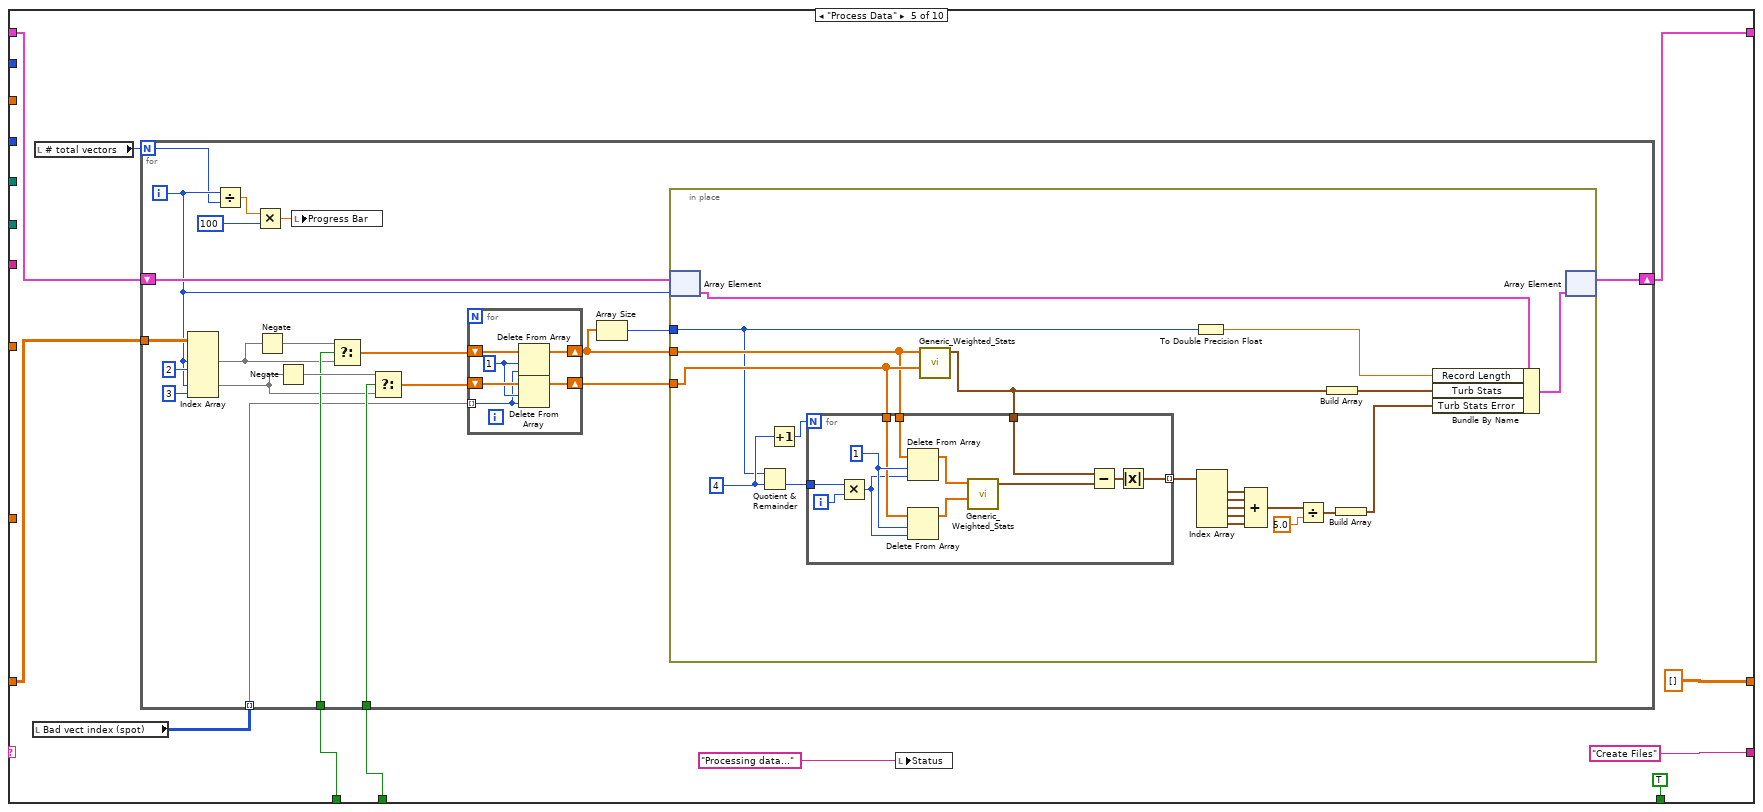
[diagram p10: hidden frame]
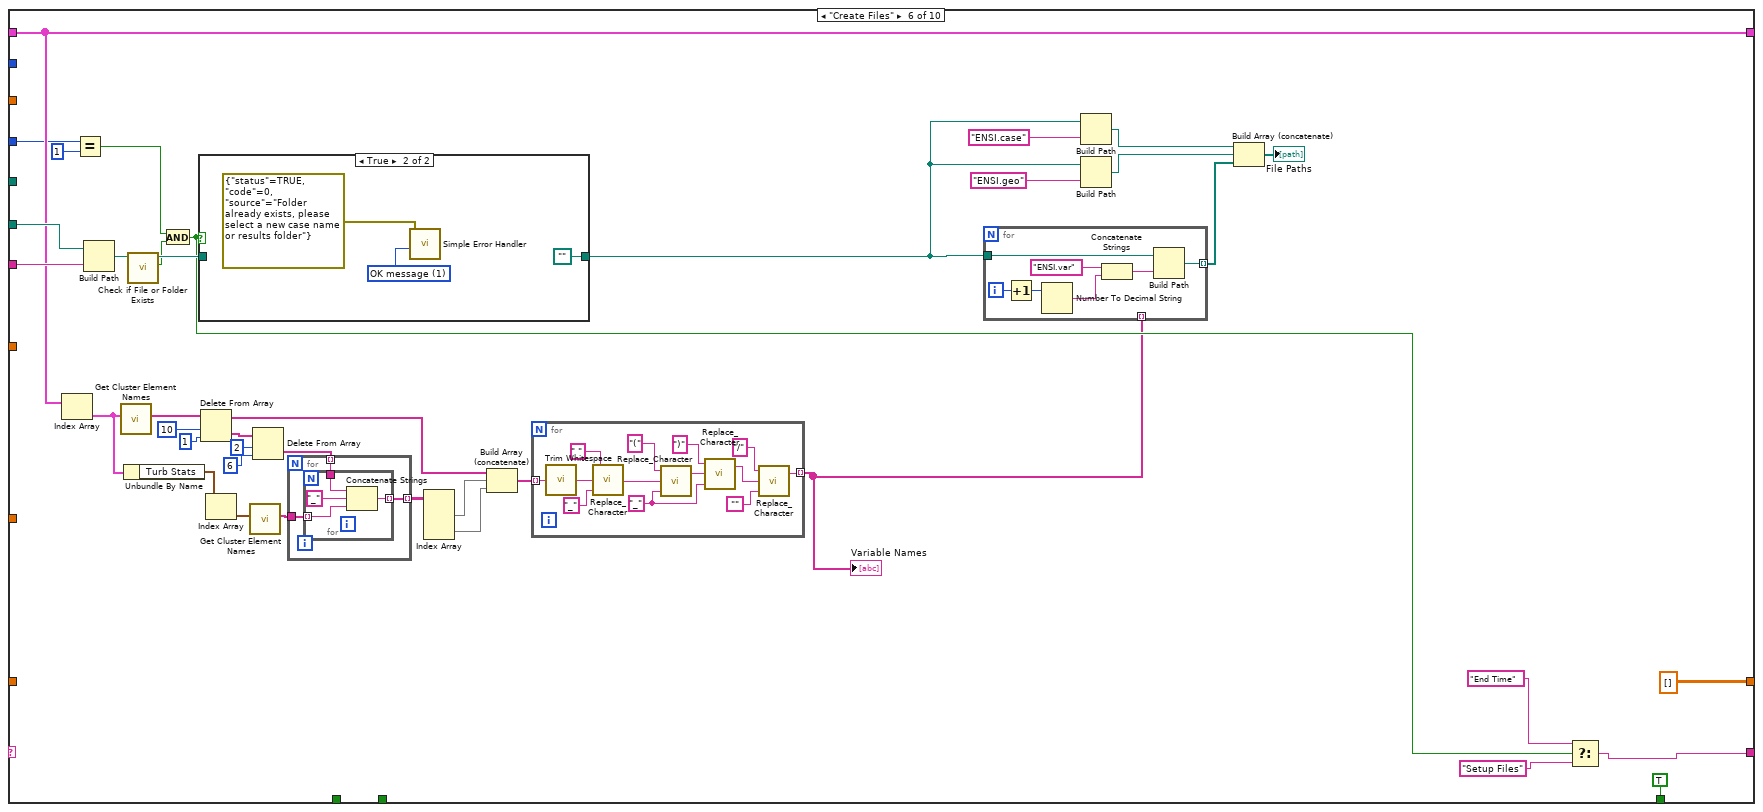
[diagram p11: hidden frame]
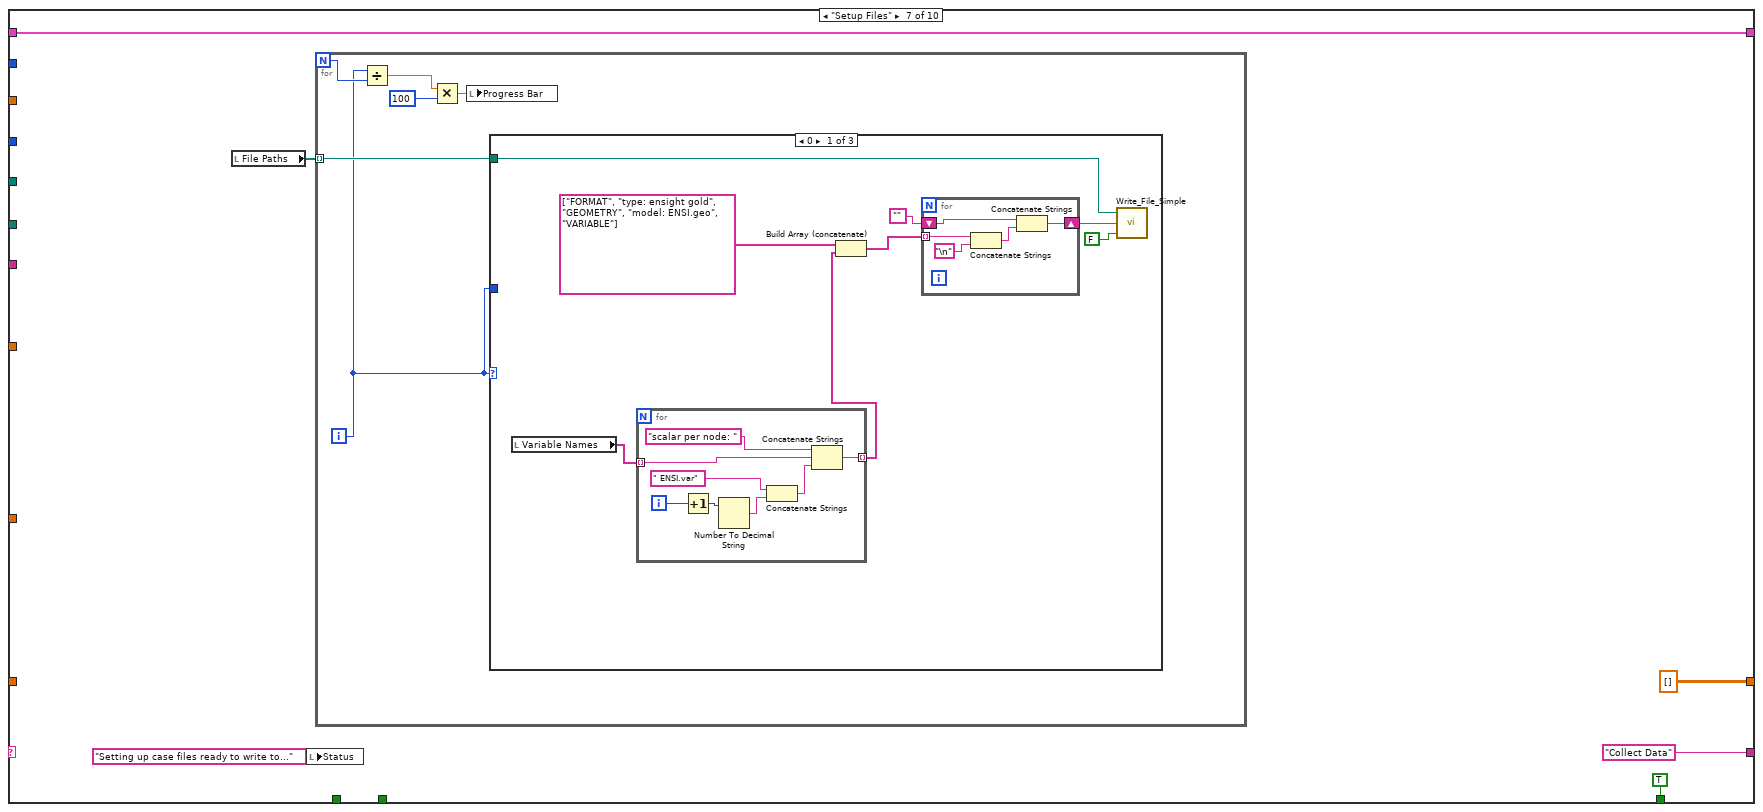
[diagram p13: hidden frame]
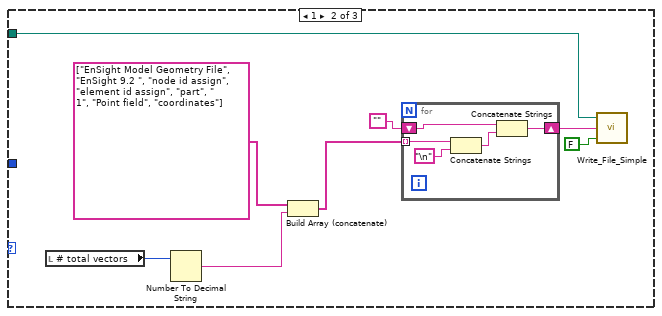
[diagram p14: hidden frame]
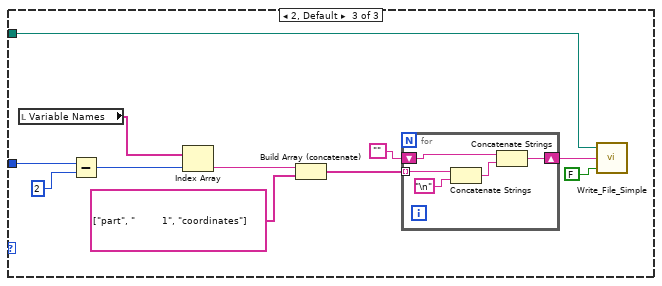
[diagram p15: hidden frame]
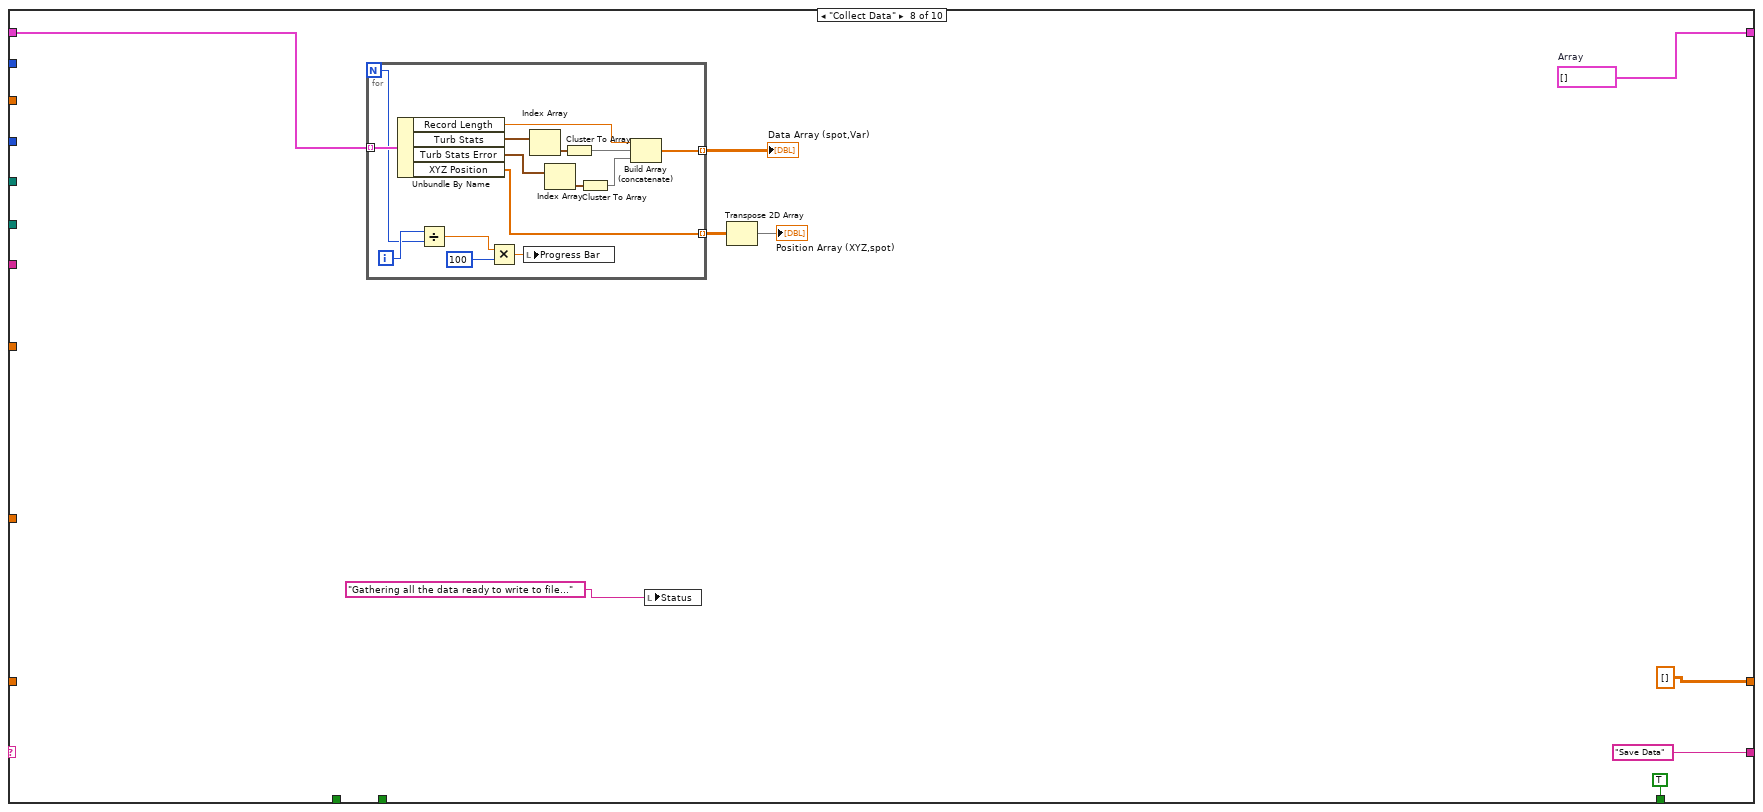
[diagram p16: hidden frame]
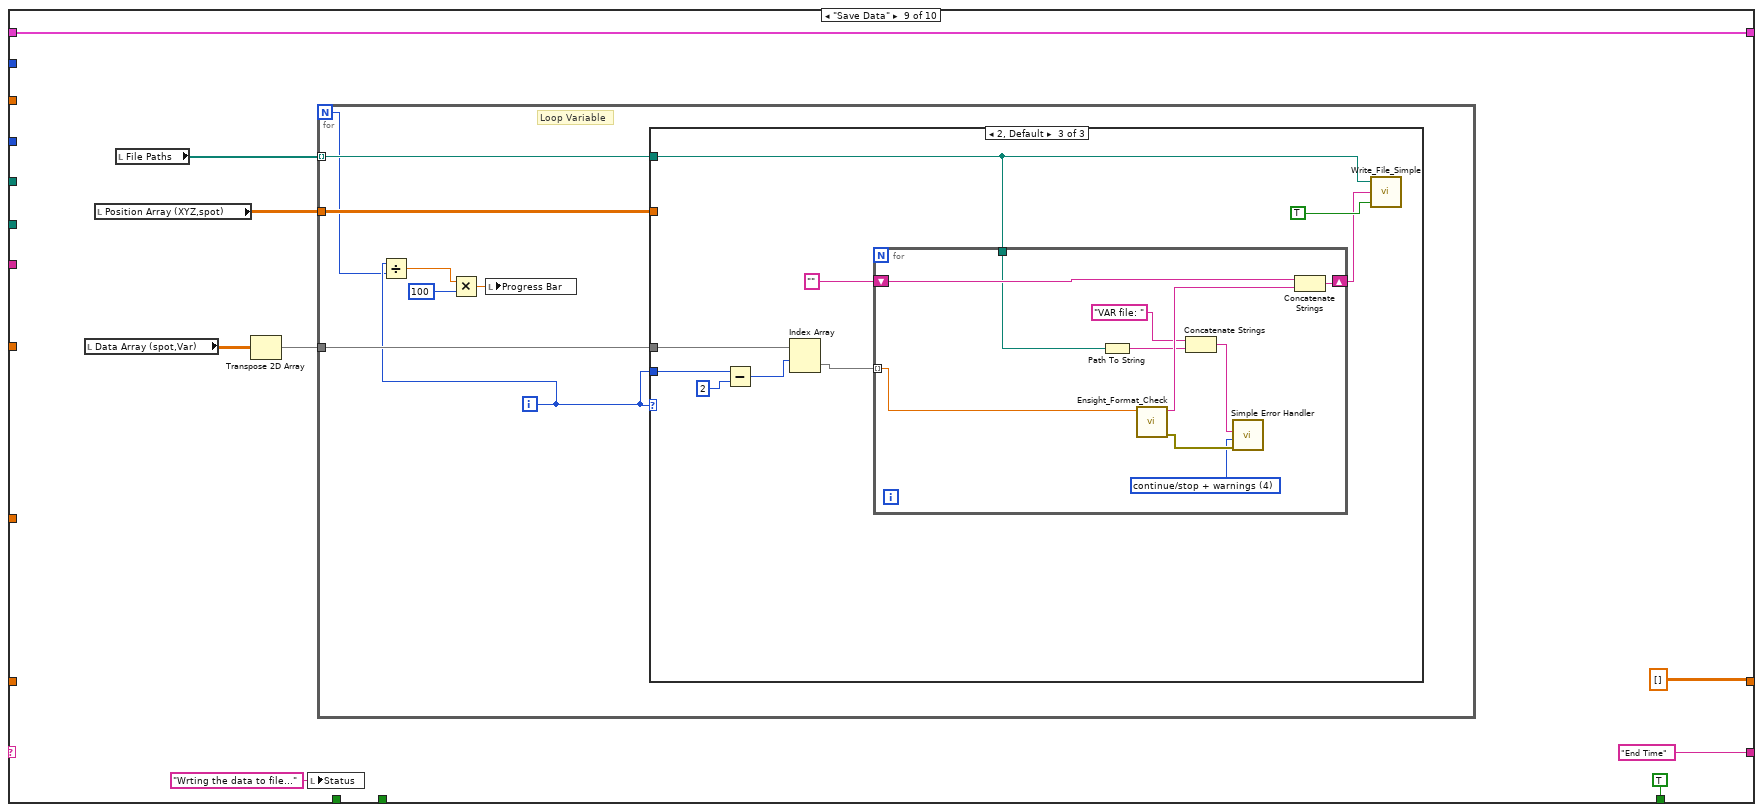
[diagram p17: hidden frame]
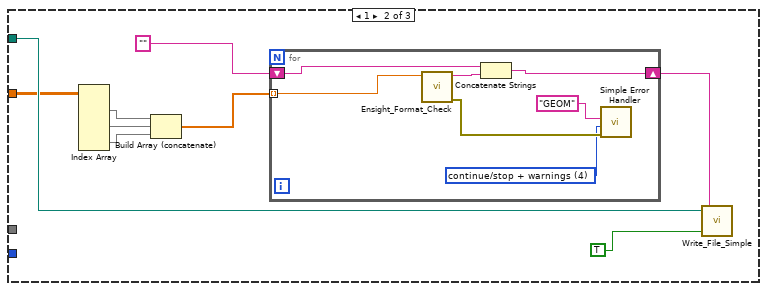
[diagram p19: hidden frame]
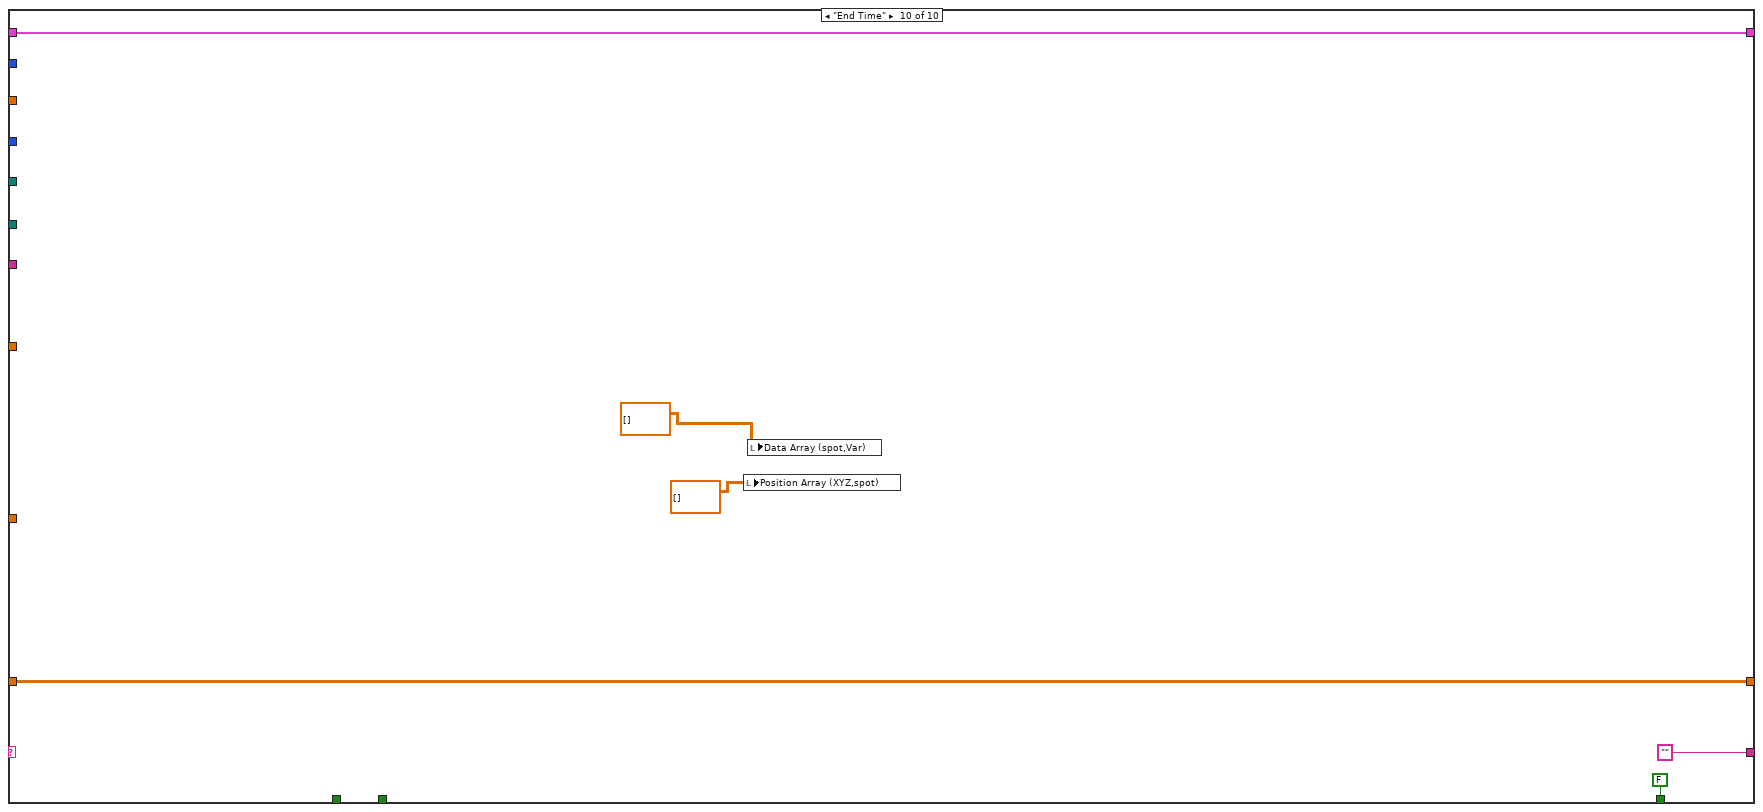
[diagram p20: hidden frame]
diagram:
  n1 = while {
    shift-right: [w28] -> _
    shift-left: "Get File Info" -> [w29]
    tunnel: "Data Folder" -> [w27]
    tunnel: "Output Directory" -> [w25]
    tunnel: "Case Name" -> [w24]
    tunnel: "PIV Freq (Hz)" -> [w23]
    tunnel: "PIV Meas Plane" -> [w22]
    tunnel: "XYZ Translation" -> [w21]
    shift-right: [w20] -> _
    shift-left: _ -> [w19]
    tunnel: "Row number" -> [w18]
    tunnel: "Invert V" -> [w17]
    tunnel: "Invert U" -> [w16]
    shift-right: [w15] -> _
    shift-left: _ -> [w14]
    tunnel: "Kurt Tolerance" -> [w13]
    stop <- w26 continue-if-true
    n2 = case shown="\"Get File Info\"" w29 {
      tunnel: ["" "Get Position" "Do Quality Check" "Process Data" "Create Files" w372 "Collect Data" ("t") "Save Data" ("t") "End Time" ("t") "" ("t")] -> w28
      tunnel: w27 -> [_ w69 _ _ _ _ _ _ _ _]
      tunnel: [FALSE TRUE TRUE TRUE TRUE TRUE TRUE TRUE TRUE FALSE] -> w26
      tunnel: w25 -> [_ w38 _ _ _ w396 _ _ _ _]
      tunnel: w24 -> [_ _ _ _ _ w397 _ _ _ _]
      tunnel: w23 -> [_ w68 _ _ _ _ _ _ _ _]
      tunnel: w22 -> [_ _ w174 _ _ _ _ _ _ _]
      tunnel: w21 -> [_ _ w175 _ _ _ _ _ _ _]
      tunnel: [w32 w56 w169 w231 w292 w382 w431 w495 w521 w568] -> w20
      tunnel: w19 -> [w32 w56 _ w231 w296 w382 w431 w497 w521 w568]
      tunnel: w18 -> [_ _ _ _ _ w378 _ _ _ _]
      tunnel: w17 -> [_ _ w167 w235 w293 _ _ _ _ _]
      tunnel: w16 -> [_ _ w166 w234 w294 _ _ _ _ _]
      tunnel: [w30 w54 w168 w229 dbl[][][] [] ("GoodRawData(time,spot)") dbl[][][] [] ("GoodRawData(time,spot)") dbl[][][] [] ("GoodRawData(time,spot)") dbl[][][] [] ("GoodRawData(time,spot)") dbl[][][] [] ("GoodRawData(time,spot)") w567] -> w15
      tunnel: w14 -> [w30 _ w168 w229 w295 _ _ _ _ w567]
      tunnel: w13 -> [_ _ _ w232 _ _ _ _ _ _]
      frame "No Match", Default {
        n3 = One Button Dialog(message="Case not matched!!") -> ()  [unwired: 1 in, 1 out]
      }
      frame "Get File Info" {
        w47 = 100.0 ("Element Data")
        n4 = List Folder(path=w69) -> (path out=w71:path, filenames=w72:string[])  [unwired: 3 in, 2 out]
        n5 = for {
          N -> [w140]
          tunnel: w72 -> [w159] mode=indexing
          shift-right: [w152] -> w59
          shift-left: path[] [] -> [w154]
          tunnel: w71 -> [w153]
          i -> [w141]
          n6 = Divide(x=w141, y=w140) -> (x/y=w143:dbl)
          n7 = Search/Split String(string=w159, search string/char (-)=".vec") -> (substring before match=w150:string, match + rest of string=w156:string)  [unwired: 1 in, 1 out]
          n8 = Multiply(x=w143, y=100) -> (x*y=w144:dbl)
          n9 = Concatenate Strings(w150, w156) -> (w155:string)
          n10 = String Length(string=w156) -> (length=w157:i32)
          n11 = Search/Split String(string=w150, search string/char (-)="_modified") -> (match + rest of string=w148:string)  [unwired: 1 in, 2 out]
          n12 = local write "Progress Bar"(w144) -> ()
          n13 = Greater Than 0?(x=w157) -> (x > 0?=w151:bool)
          n14 = String Length(string=w148) -> (length=w147:i32)
          n15 = Equal To 0?(x=w147) -> (x = 0?=w146:bool)
          n16 = And(x=w151, y=w146) -> (x .and. y?=w145:bool)
          n17 = case shown="True" w145 {
            tunnel: w155 -> [_ w165]
            tunnel: w154 -> [w160 w161]
            tunnel: w153 -> [_ w164]
            tunnel: [w160 w162] -> w152
            frame False {
            }
            frame True {
              n18 = Build Path(base path=w164, name or relative path=w165) -> (appended path=w163:path)
              n19 = Build Array (concatenate)(w161, w163) -> (w162:path[])
            }
          }
        }
        "File Array" <- w59
        n20 = local write "Position Array (XYZ,spot)"(dbl[][] [] ("Position Array")) -> ()
        n21 = local write "Data Array (spot,Var)"(dbl[][] [] ("Data Array")) -> ()
        n22 = Array Size(array=w59) -> (size(s)=w63:i32)
        n23 = Reciprocal(x=w68) -> (1/x=w66:dbl)
        n24 = Multiply(x=w66, y=w63) -> (x*y=w67:dbl)
        n25 = for {
          N -> [w100]
          tunnel: w59 -> [w106] mode=indexing
          tunnel: [w93] -> w58 mode=indexing
          tunnel: [w104] -> w54 mode=indexing
          tunnel: "Collecting Raw data from all vectors" ("Status") -> [w98]
          tunnel: [w80] -> w53 mode=indexing
          tunnel: [w76] -> w51 mode=indexing
          tunnel: [w75] -> w52 mode=indexing
          i -> [w99]
          n26 = local write "Status"(w98) -> ()
          n27 = Divide(x=w99, y=w100) -> (x/y=w102:dbl)
          n28 = Read from Text File(file (use dialog)=w106) -> (text=w115:string)  [unwired: 3 in, 3 out]
          n29 = Multiply(x=w102, y=100) -> (x*y=w101:dbl)
          n30 = Match Pattern(string=w115, regular expression="\n") -> (after substring=w111:string)  [unwired: 1 in, 3 out]
          n31 = local write "Progress Bar"(w101) -> ()
          n32 = Spreadsheet String To Array(delimiter (Tab)=",", format string="%.6f", spreadsheet string=w111) -> (array=w91:dbl[][])  [unwired: 1 in]
          n33 = Transpose 2D Array(2D array=w91) -> (transposed array=w110:dbl[][])
          n34 = Index Array(array=w110, index (row)=4) -> (element=w88:dbl[])  [unwired: 1 in]
          n35 = call "Search_1D_Array(DBL).vi"("Array"=w88, "Element Data"=4.0) -> ("Indicies of Elements"=w85:i32[])  [unwired: 6 in, 1 out]
          n36 = call "Search_1D_Array(DBL).vi"("Array"=w88, "Element Data"=1.0) -> ("Indicies of Elements"=w86:i32[])  [unwired: 6 in, 1 out]
          n37 = call "Search_1D_Array(DBL).vi"("Array"=w88, "Element Data"=-1.0) -> ("Indicies of Elements"=w87:i32[])  [unwired: 6 in, 1 out]
          n38 = Build Array (concatenate)(w85) -> (w82:i32[])
          n39 = Build Array (concatenate)(w87) -> (w84:i32[])
          n40 = Build Array (concatenate)(w86) -> (w83:i32[])
          n41 = Build Array (concatenate)(w87, w86, w85) -> (w95:i32[])
          n42 = Build Array (concatenate)(w87, w86, w85) -> (w90:i32[])
          n43 = Array Size(array=w84) -> (size(s)=w78:i32)
          n44 = Array Size(array=w83) -> (size(s)=w81:i32)
          n45 = Array Size(array=w82) -> (size(s)=w77:i32)
          n46 = Array Size(array=w90) -> (size(s)=w79:i32)
          n47 = Array Size(array=w95) -> (size(s)=w93:i32)
          n48 = Divide(x=w78, y=w79) -> (x/y=w76:dbl)
          n49 = Divide(x=w81, y=w79) -> (x/y=w80:dbl)
          n50 = Divide(x=w77, y=w79) -> (x/y=w75:dbl)
          n51 = Initialize Array(0.0 ("element"), 5 ("dimension size"), w93) -> (w105:dbl[][])
          n52 = Transpose 2D Array(2D array=w105) -> (transposed array=w92:dbl[][])
          n53 = for {
            tunnel: w91 -> [w127] mode=indexing
            shift-right: [w130] -> w104
            shift-left: w92 -> [w125]
            shift-right: [w129] -> _
            shift-left: 0 ("y") -> [w128]
            tunnel: w91 -> [w126]
            i -> [w124]
            n54 = Index Array(array=w127, index=4) -> (element=w121:dbl)
            n55 = Index Array(array=w126, index (row)=w124) -> (element=w131:dbl[])  [unwired: 1 in]
            n56 = Equal?(x=w121, y=1.0) -> (x = y?=w117:bool)
            n57 = Equal?(x=w121, y=4.0) -> (x = y?=w118:bool)
            n58 = Equal?(x=w121, y=-1.0) -> (x = y?=w119:bool)
            n59 = Compound Arithmetic op=OR(w117, w118, w119) -> (w116:bool)
            n60 = case shown="True" w116 {
              tunnel: w131 -> [_ w137]
              tunnel: w125 -> [w134 w139]
              tunnel: [w134 w138] -> w130
              tunnel: [w133 w136] -> w129
              tunnel: w128 -> [w133 w135]
              frame False {
              }
              frame True {
                n61 = Increment(x=w135) -> (x+1=w136:i32)
                n62 = Replace Array Subset(array=w139, new element=w137, index (row)=w135) -> (w138:dbl[][])  [unwired: 1 in]
              }
            }
          }
        }
        n63 = call-poly <vilib>:"Ramp Pattern.vi"("start"=0.0, "end"=w67, "samples"=w63) -> ("Ramp Pattern"=→"time s":dbl[])  [unwired: 7 in, 1 out]
        n64 = Multiply(x=w53, y=w47) -> (x*y=w48:dbl[])
        n65 = Multiply(x=w52, y=w47) -> (x*y=w50:dbl[])
        n66 = Multiply(x=w51, y=w47) -> (x*y=w49:dbl[])
        n67 = Array Max & Min(array=w58) -> (max value=→"# total vectors":i32)  [unwired: 3 out]
        n68 = Build Array(w48) -> (w46:dbl[][])
        n69 = Build Array(w49) -> (w45:dbl[][])
        n70 = Build Array(w50) -> (w43:dbl[][])
        n71 = Transpose 2D Array(2D array=w46) -> (transposed array=w41:dbl[][])
        "good vectors %" <- w41
        n72 = Transpose 2D Array(2D array=w45) -> (transposed array=→"bad vectors %":dbl[][])
        n73 = Transpose 2D Array(2D array=w43) -> (transposed array=→"interpolated vetors %":dbl[][])
        n74 = Array To Spreadsheet String(array=w41, 3:"%.6f" ("format string")) -> (spreadsheet string=w40:string)  [unwired: 1 in]
        n75 = Build Path(base path=w38, name or relative path="good_vect_list.xls" ("search string/char (-)")) -> (appended path=w37:path)
        n76 = call "Write_File_Simple.vi"("append to file? (new file:F)"=FALSE, "character string"=w40, "file path"=w37) -> ()  [unwired: 2 out]
        "Status" <- "Getting file information from the data folder..." ("Status")
      }
      frame "Get Position" {
        n77 = local read "# total vectors"() -> (w173:i32)
        n78 = Initialize Array(T1 {"Record Length"=0.0, "CHC"=[], "u m/s"=[], "v m/s"=[], "time s"=[], "Vel mag m/s"=[], "XYZ Position"=[], " Turb Stats"=[], "Turb Stats Error"=[], "u (good)"=[], "v (good)"=[]} ("Spot Data Cluster"), w173) -> (w171:T2)
        n79 = for {
          N -> [w190]
          shift-right: [w195] -> w169
          shift-left: w171 -> [w196]
          tunnel: w168 -> [w188] mode=indexing
          tunnel: w175 -> [w197]
          tunnel: w174 -> [w189]
          tunnel: "Getting PIV spot positions for all vecotrs" ("Status") -> [w186]
          tunnel: w167 -> [w185]
          tunnel: w166 -> [w184]
          i -> [w191]
          n80 = Transpose 2D Array(2D array=w188) -> (transposed array=w187:dbl[][])
          n81 = Divide(x=w191, y=w190) -> (x/y=w193:dbl)
          n82 = Index Array(array=w187) -> (element #1=w180:dbl[], element #2=w178:dbl[])  [unwired: 4 in]
          n83 = Multiply(x=w193, y=100) -> (x*y=w194:dbl)
          n84 = Negate(x=w180) -> (-x=w181:dbl[])
          n85 = local write "Progress Bar"(w194) -> ()
          n86 = Negate(x=w178) -> (-x=w179:dbl[])
          n87 = Select(t=w181, s=w184, f=w180) -> (s? t:f=w182:dbl[])
          n88 = Select(t=w179, s=w185, f=w178) -> (s? t:f=w183:dbl[])
          n89 = for {
            tunnel: w182 -> [w204] mode=indexing
            tunnel: w183 -> [w203] mode=indexing
            tunnel: w197 -> [w202]
            shift-right: [w199] -> w195
            shift-left: w196 -> [w201]
            tunnel: w189 -> [w198]
            i -> [w200]
            n90 = in-place {
              in-place-border: w204 -> [w211]
              in-place-border: w203 -> [w210]
              in-place-border: w202 -> [w209]
              in-place-border: w198 -> [w205]
              n91 = in-place-array #1(w201, w200) -> (w208:T1)
              n92 = case shown="\"XY\"" w205 {
                tunnel: w211 -> [w215 w221 w225]
                tunnel: w210 -> [w216 w220 w224]
                tunnel: 0.0 ("element") -> [w217 w219 w223]
                tunnel: [w214 w218 w222] -> w213
                frame "XY" {
                  n93 = Build Array(w215, w216, w217) -> (w214:dbl[])
                }
                frame "YZ" {
                  n94 = Build Array(w219, w221, w220) -> (w218:dbl[])
                }
                frame "XZ" {
                  n95 = Build Array(w225, w223, w224) -> (w222:dbl[])
                }
              }
              n96 = Add(x=w209, y=w213) -> (x+y=w207:dbl[])
              n97 = Bundle By Name(cluster=w208, "XYZ Position"=w207) -> (w206:T1)
              n98 = in-place-array #1(w206) -> (w199:T2)  [unwired: 1 out]
            }
          }
          n99 = local write "Status"(w186) -> ()
        }
      }
      frame "Do Quality Check" {
        n100 = local read "# total vectors"() -> (w226:i32)
        n101 = for {
          N: w226 -> [w254]
          tunnel: w235 -> [w253]
          tunnel: w234 -> [w252]
          tunnel: w229 -> [w246]
          tunnel: w232 -> [w245]
          tunnel: [w239] -> w228 mode=indexing
          tunnel: [w238] -> w230 mode=indexing
          i -> [w247]
          n102 = Index Array(array=w246, index (dim 1) #1=w247, index (dim 2) #1=2 ("disabled index (col)"), index (dim 1) #2=w247, index (dim 2) #2=3 ("disabled index (col)")) -> (element #1=w249:dbl[], element #2=w248:dbl[])  [unwired: 2 in]
          n103 = Divide(x=w247, y=w254) -> (x/y=w256:dbl)
          n104 = Multiply(x=w256, y=100) -> (x*y=w257:dbl)
          n105 = Negate(x=w249) -> (-x=w261:dbl[])
          n106 = Negate(x=w248) -> (-x=w260:dbl[])
          n107 = local write "Progress Bar"(w257) -> ()
          n108 = Select(t=w261, s=w252, f=w249) -> (s? t:f=w259:dbl[])
          n109 = Select(t=w260, s=w253, f=w248) -> (s? t:f=w258:dbl[])
          n110 = Array Size(array=w259) -> (size(s)=w244:i32)
          n111 = call "Generic_Weighted_Stats.vi"("v"=w258, "u"=w259) -> ("Turbulence Statistics"=w243:T3)  [unwired: 9 in]
          n112 = Unbundle By Name(w243) -> ("Kurt_u"=w241:dbl, "Kurt_v"=w242:dbl)
          n113 = for {
            N: w244 -> [_]
            tunnel: w259 -> [w279]
            tunnel: w258 -> [w278]
            tunnel: w242 -> [w263]
            tunnel: w241 -> [w265]
            tunnel: w245 -> [w273]
            shift-right: [w269] -> w238
            shift-left: i32[] [] -> [w268]
            i -> [w267]
            w277 = 1 ("length")
            n114 = Delete From Array(array=w278, length=w277, index=w267) -> (array with subset deleted=w281:dbl[])  [unwired: 1 out]
            n115 = Delete From Array(array=w279, length=w277, index=w267) -> (array with subset deleted=w282:dbl[])  [unwired: 1 out]
            n116 = call "Generic_Weighted_Stats.vi"("v"=w281, "u"=w282) -> ("Turbulence Statistics"=w266:T3)  [unwired: 9 in]
            n117 = Unbundle By Name(w266) -> ("Kurt_u"=w264:dbl, "Kurt_v"=w262:dbl)
            n118 = Subtract(x=w265, y=w264) -> (x-y=w280:dbl)
            n119 = Subtract(x=w263, y=w262) -> (x-y=w276:dbl)
            n120 = Absolute Value(x=w280) -> (abs(x)=w275:dbl)
            n121 = Absolute Value(x=w276) -> (abs(x)=w274:dbl)
            n122 = Greater?(x=w275, y=w273) -> (0:w271:bool)
            n123 = Greater?(x=w274, y=w273) -> (0:w272:bool)
            n124 = Or(x=w271, y=w272) -> (x .or. y?=w270:bool)
            n125 = case shown="False" w270 {
              tunnel: [w283 w286] -> w269
              tunnel: w268 -> [w283 w285]
              tunnel: w267 -> [_ w284]
              frame False {
              }
              frame True {
                n126 = Build Array (concatenate)(w285, w284) -> (w286:i32[])
              }
            }
          }
          n127 = Array Size(array=w238) -> (size(s)=w239:i32)
        }
        "Bad vect index (spot)" <- w230
        n128 = local write "Status"("Doing vector quality checks..." ("Status")) -> ()
        n129 = Array Max & Min(array=w228) -> (max value=→"max bad vectors":i32)  [unwired: 3 out]
      }
      frame "Process Data" {
        n130 = local read "Bad vect index (spot)"() -> (w287:i32[][])
        n131 = local read "# total vectors"() -> (w297:i32)
        n132 = for {
          N: w297 -> [w301]
          tunnel: w293 -> [w314]
          tunnel: w294 -> [w313]
          tunnel: w295 -> [w308]
          shift-right: [w305] -> w292
          shift-left: w296 -> [w304]
          tunnel: w287 -> [w306] mode=indexing
          i -> [w303]
          n133 = Index Array(array=w308, index (dim 1) #1=w303, index (dim 2) #1=2 ("disabled index (col)"), index (dim 1) #2=w303, index (dim 2) #2=3 ("disabled index (col)")) -> (element #1=w310:dbl[], element #2=w309:dbl[])  [unwired: 2 in]
          n134 = Divide(x=w303, y=w301) -> (x/y=w316:dbl)
          n135 = Multiply(x=w316, y=100) -> (x*y=w317:dbl)
          n136 = Negate(x=w310) -> (-x=w319:dbl[])
          n137 = Negate(x=w309) -> (-x=w318:dbl[])
          n138 = local write "Progress Bar"(w317) -> ()
          n139 = Select(t=w319, s=w313, f=w310) -> (s? t:f=w300:dbl[])
          n140 = Select(t=w318, s=w314, f=w309) -> (s? t:f=w307:dbl[])
          n141 = for {
            shift-right: [w355] -> w299
            shift-left: w300 -> [w358]
            shift-right: [w354] -> w302
            shift-left: w307 -> [w357]
            tunnel: w306 -> [w353] mode=indexing
            w356 = 1 ("length")
            n142 = Delete From Array(array=w358, length=w356, index=w353) -> (array with subset deleted=w355:dbl[])  [unwired: 1 out]
            n143 = Delete From Array(array=w357, length=w356, index=w353) -> (array with subset deleted=w354:dbl[])  [unwired: 1 out]
          }
          n144 = Array Size(array=w299) -> (size(s)=w298:i32)
          n145 = in-place {
            in-place-border: w299 -> [w334]
            in-place-border: w302 -> [w335]
            in-place-border: w298 -> [w320]
            w336 = 4 ("y")
            n146 = in-place-array #2(w304, w303) -> (w340:T1)
            n147 = Quotient & Remainder(x=w320, y=w336) -> (floor(x/y)=w332:i32)  [unwired: 1 out]
            n148 = Increment(x=w336) -> (x+1=w337:i32)
            n149 = call "Generic_Weighted_Stats.vi"("v"=w335, "u"=w334) -> ("Turbulence Statistics"=w331:T3)  [unwired: 9 in]
            n150 = for {
              N: w337 -> [_]
              tunnel: w331 -> [w342]
              tunnel: w332 -> [w349]
              tunnel: w334 -> [w346]
              tunnel: w335 -> [w345]
              tunnel: [w343] -> w330 mode=indexing
              i -> [w348]
              w347 = 1 ("y")
              n151 = Multiply(x=w349, y=w348) -> (x*y=w344:i32)
              n152 = Delete From Array(array=w346, length=w347, index=w344) -> (array with subset deleted=w352:dbl[])  [unwired: 1 out]
              n153 = Delete From Array(array=w345, length=w347, index=w344) -> (array with subset deleted=w351:dbl[])  [unwired: 1 out]
              n154 = call "Generic_Weighted_Stats.vi"("v"=w351, "u"=w352) -> ("Turbulence Statistics"=w341:T3)  [unwired: 9 in]
              n155 = Subtract(x=w342, y=w341) -> (x-y=w350:T3)
              n156 = Absolute Value(x=w350) -> (abs(x)=w343:T3)
            }
            n157 = To Double Precision Float(number=w320) -> (double precision float=w338:dbl)
            n158 = Index Array(array=w330) -> (element #1=w329:T3, element #2=w328:T3, element #3=w327:T3, element #4=w326:T3, element #5=w325:T3)  [unwired: 5 in]
            n159 = Compound Arithmetic op=ADD(w329, w328, w327, w326, w325) -> (w324:T3)
            n160 = Divide(x=w324, y=5.0 ("Record Length")) -> (x/y=w322:T3)
            n161 = Build Array(w331) -> (w333:T4)
            n162 = Build Array(w322) -> (w321:T4)
            n163 = Bundle By Name(cluster=w340, "Record Length"=w338, "Turb Stats"=w333, "Turb Stats Error"=w321) -> (w339:T1)
            n164 = in-place-array #2(w339) -> (w305:T2)  [unwired: 1 out]
          }
        }
        n165 = local write "Status"("Processing data..." ("Status")) -> ()
      }
      frame "Create Files" {
        n166 = Index Array(array=w382) -> (element=w394:T1)  [unwired: 1 in]
        n167 = Equal?(x=w378, y=1) -> (x = y?=w373:bool)
        n168 = Build Path(base path=w396, name or relative path=w397) -> (appended path=w376:path)
        n169 = call "Get Cluster Element Names.vi"("Cluster"=w394) -> ("Element Names"=w393:string[])  [unwired: 9 in, 1 out]
        n170 = Unbundle By Name(w394) -> ("Turb Stats"=w384:T4)
        n171 = call <vilib>:"Check if File or Folder Exists.vi"("path"=w376) -> ("file or folder exists?"=w374:bool, "dup path"=w375:path)  [unwired: 8 in, 1 out]
        n172 = And(x=w373, y=w374) -> (x .and. y?=w370:bool)
        n173 = case shown="True" w370 {
          tunnel: [w405 path "" ("dup path")] -> w362
          tunnel: w375 -> [w405 _]
          frame False {
          }
          frame True {
            w408 = T5 1 items=["no dialog", "OK message", "continue or stop message", "OK message + warnings", "continue/stop + warnings"] ("type of dialog (OK msg:1)")
            n174 = call <vilib>:"Simple Error Handler.vi"("type of dialog (OK msg:1)"=w408, "error in (no error)"=errorcluster {"status"=TRUE, "code"=0, "source"="Folder already exists, please select a new case name or results folder"}) -> ()  [unwired: 3 in, 5 out]
          }
        }
        n175 = Delete From Array(array=w393, length=10, index=1) -> (deleted portion=w381:string[], array with subset deleted=w389:string[])
        n176 = Index Array(array=w384) -> (element=w383:T3)  [unwired: 1 in]
        n177 = call "Get Cluster Element Names.vi"("Cluster"=w383) -> ("Element Names"=w390:string[])  [unwired: 9 in, 1 out]
        n178 = Delete From Array(array=w381, length=2, index=6) -> (deleted portion=w359:string[])  [unwired: 1 out]
        n179 = for {
          tunnel: w359 -> [w411] mode=indexing
          tunnel: w390 -> [w410]
          tunnel: [w409] -> w388 mode=indexing
          n180 = for {
            tunnel: w411 -> [w415]
            tunnel: w410 -> [w413] mode=indexing
            tunnel: [w412] -> w409 mode=indexing
            n181 = Concatenate Strings(w415, "_" ("string"), w413) -> (w412:string)
          }
        }
        n182 = Index Array(array=w388) -> (element #1=w387:string[], element #2=w386:string[])  [unwired: 4 in]
        n183 = Build Array (concatenate)(w389, w387, w386) -> (w385:string[])
        n184 = for {
          tunnel: w385 -> [w418] mode=indexing
          tunnel: [w420] -> w363 mode=indexing
          w424 = "_" ("Replace with")
          n185 = call <vilib>:"Trim Whitespace.vi"("string"=w418) -> ("trimmed string"=w416:string)  [unwired: 1 in]
          n186 = call "Replace_Character.vi"("Replace with"="_", "Input String"=w416, "Search For"=" ") -> ("Output string"=w419:string)  [unwired: 1 out]
          n187 = call "Replace_Character.vi"("Replace with"=w424, "Input String"=w419, "Search For"="(") -> ("Output string"=w426:string)  [unwired: 1 out]
          n188 = call "Replace_Character.vi"("Replace with"=w424, "Input String"=w426, "Search For"=")") -> ("Output string"=w423:string)  [unwired: 1 out]
          n189 = call "Replace_Character.vi"("Replace with"="", "Input String"=w423, "Search For"="/") -> ("Output string"=w420:string)  [unwired: 1 out]
        }
        "Variable Names" <- w363
        n190 = for {
          tunnel: w362 -> [w404]
          tunnel: [w398] -> w368 mode=indexing
          tunnel: w363 -> [_] mode=indexing
          i -> [w403]
          n191 = Increment(x=w403) -> (x+1=w402:i32)
          n192 = Number To Decimal String(number=w402) -> (decimal integer string=w400:string)  [unwired: 1 in]
          n193 = Concatenate Strings("ENSI.var" ("name or relative path"), w400) -> (w399:string)
          n194 = Build Path(base path=w404, name or relative path=w399) -> (appended path=w398:path)
        }
        n195 = Build Path(base path=w362, name or relative path="ENSI.case") -> (appended path=w366:path)
        n196 = Build Path(base path=w362, name or relative path="ENSI.geo") -> (appended path=w367:path)
        n197 = Build Array (concatenate)(w366, w367, w368) -> (→"File Paths":path[])
        n198 = Select(t="End Time", s=w370, f="Setup Files" ("t")) -> (s? t:f=w372:string)
      }
      frame "Setup Files" {
        n199 = local read "File Paths"() -> (w434:path[])
        n200 = local write "Status"("Setting up case files ready to write to..." ("Status")) -> ()
        n201 = for {
          N -> [w437]
          tunnel: w434 -> [w440] mode=indexing
          i -> [w435]
          n202 = Divide(x=w435, y=w437) -> (x/y=w436:dbl)
          n203 = Multiply(x=w436, y=100) -> (x*y=w439:dbl)
          n204 = local write "Progress Bar"(w439) -> ()
          n205 = case shown="0" w435 {
            tunnel: w440 -> [w445 w466 w485]
            tunnel: w435 -> [_ _ w480]
            frame 0 {
              n206 = local read "Variable Names"() -> (w442:string[])
              n207 = for {
                tunnel: w442 -> [w451] mode=indexing
                tunnel: [w449] -> w441 mode=indexing
                i -> [w454]
                n208 = Increment(x=w454) -> (x+1=w455:i32)
                n209 = Number To Decimal String(number=w455) -> (decimal integer string=w452:string)  [unwired: 1 in]
                n210 = Concatenate Strings(" ENSI.var", w452) -> (w450:string)
                n211 = Concatenate Strings("scalar per node: ", w451, w450) -> (w449:string)
              }
              n212 = Build Array (concatenate)(string[] ["FORMAT", "type: ensight gold", "GEOMETRY", "model: ENSI.geo", "VARIABLE"], w441) -> (w444:string[])
              n213 = for {
                tunnel: w444 -> [w461] mode=indexing
                shift-right: [w459] -> w447
                shift-left: "" -> [w457]
                n214 = Concatenate Strings(w461, "\n") -> (w458:string)
                n215 = Concatenate Strings(w457, w458) -> (w459:string)
              }
              n216 = call "Write_File_Simple.vi"("append to file? (new file:F)"=FALSE, "character string"=w447, "file path"=w445) -> ()  [unwired: 2 out]
            }
            frame 1 {
              n217 = local read "# total vectors"() -> (w464:i32)
              n218 = Number To Decimal String(number=w464) -> (decimal integer string=w463:string)  [unwired: 1 in]
              n219 = Build Array (concatenate)(string[] ["EnSight Model Geometry File", "EnSight 9.2 ", "node id assign", "element id assign", "part", "         1", "Point field", "coordinates"], w463) -> (w462:string[])
              n220 = for {
                tunnel: w462 -> [w474] mode=indexing
                shift-right: [w472] -> w468
                shift-left: "" -> [w470]
                n221 = Concatenate Strings(w474, "\n") -> (w471:string)
                n222 = Concatenate Strings(w470, w471) -> (w472:string)
              }
              n223 = call "Write_File_Simple.vi"("append to file? (new file:F)"=FALSE, "character string"=w468, "file path"=w466) -> ()  [unwired: 2 out]
            }
            frame 2, Default {
              n224 = local read "Variable Names"() -> (w481:string[])
              n225 = Subtract(x=w480, y=2) -> (x-y=w478:i32)
              n226 = Index Array(array=w481, index=w478) -> (element=w477:string)
              n227 = Build Array (concatenate)(w477, string[] ["part", "         1", "coordinates"]) -> (w475:string[])
              n228 = for {
                tunnel: w475 -> [w490] mode=indexing
                shift-right: [w488] -> w483
                shift-left: "" -> [w486]
                n229 = Concatenate Strings(w490, "\n") -> (w487:string)
                n230 = Concatenate Strings(w486, w487) -> (w488:string)
              }
              n231 = call "Write_File_Simple.vi"("append to file? (new file:F)"=FALSE, "character string"=w483, "file path"=w485) -> ()  [unwired: 2 out]
            }
          }
        }
      }
      frame "Collect Data" {
        w495 = T2 []  # Array
        n232 = for {
          N -> [w506]
          tunnel: w497 -> [w514] mode=indexing
          tunnel: [w512] -> w491 mode=indexing
          tunnel: [w511] -> w493 mode=indexing
          i -> [w507]
          n233 = Unbundle By Name(w514) -> ("Record Length"=w513:dbl, "Turb Stats"=w505:T4, "Turb Stats Error"=w502:T4, "XYZ Position"=w511:dbl[])
          n234 = Divide(x=w507, y=w506) -> (x/y=w509:dbl)
          n235 = Multiply(x=w509, y=100) -> (x*y=w510:dbl)
          n236 = local write "Progress Bar"(w510) -> ()
          n237 = Index Array(array=w505) -> (element=w504:T3)  [unwired: 1 in]
          n238 = Index Array(array=w502) -> (element=w501:T3)  [unwired: 1 in]
          n239 = Cluster To Array(cluster=w504) -> (array=w503:dbl[])
          n240 = Cluster To Array(cluster=w501) -> (array=w500:dbl[])
          n241 = Build Array (concatenate)(w513, w503, w500) -> (w512:dbl[])
        }
        "Data Array (spot,Var)" <- w491
        n242 = local write "Status"("Gathering all the data ready to write to file..." ("Status")) -> ()
        n243 = Transpose 2D Array(2D array=w493) -> (transposed array=→"Position Array (XYZ,spot)":dbl[][])
      }
      frame "Save Data" {
        n244 = local read "Data Array (spot,Var)"() -> (w519:dbl[][])
        n245 = local read "Position Array (XYZ,spot)"() -> (w518:dbl[][])
        n246 = local read "File Paths"() -> (w520:path[])
        n247 = Transpose 2D Array(2D array=w519) -> (transposed array=w515:dbl[][])
        n248 = local write "Status"("Wrting the data to file..." ("Status")) -> ()
        n249 = for {
          N -> [w524]
          tunnel: w520 -> [w531] mode=indexing
          tunnel: w515 -> [w530]
          tunnel: w518 -> [w529]
          i -> [w525]
          # "Loop Variable"
          n250 = Divide(x=w525, y=w524) -> (x/y=w527:dbl)
          n251 = Multiply(x=w527, y=100) -> (x*y=w528:dbl)
          n252 = local write "Progress Bar"(w528) -> ()
          n253 = case shown="2, Default" w525 {
            tunnel: w531 -> [_ w537 w549]
            tunnel: w525 -> [_ _ w556]
            tunnel: w530 -> [_ _ w553]
            tunnel: w529 -> [_ w536 _]
            frame 0 {
            }
            frame 1 {
              n254 = Index Array(array=w536) -> (element #1=w535:dbl[], element #2=w534:dbl[], element #3=w533:dbl[])  [unwired: 6 in]
              n255 = Build Array (concatenate)(w535, w534, w533) -> (w532:dbl[])
              n256 = for {
                tunnel: w532 -> [w541] mode=indexing
                shift-right: [w547] -> w538
                shift-left: "" -> [w546]
                w542 = T5 4 items=["no dialog", "OK message", "continue or stop message", "OK message + warnings", "continue/stop + warnings"] ("type of dialog (OK msg:1)")
                n257 = call "Ensight_Format_Check.vi"("Input Number"=w541) -> ("error"=w544:errorcluster, "Output string"=w545:string)  [unwired: 8 in, 1 out]
                n258 = Concatenate Strings(w546, w545) -> (w547:string)
                n259 = call <vilib>:"Simple Error Handler.vi"("error source (\" \")"="GEOM" ("error source (\" \")"), "type of dialog (OK msg:1)"=w542, "error in (no error)"=w544) -> ()  [unwired: 2 in, 5 out]
              }
              n260 = call "Write_File_Simple.vi"("append to file? (new file:F)"=TRUE, "character string"=w538, "file path"=w537) -> ()  [unwired: 2 out]
            }
            frame 2, Default {
              n261 = Subtract(x=w556, y=2) -> (x-y=w548:i32)
              n262 = Index Array(array=w553, index (row)=w548) -> (element=w552:dbl[])  [unwired: 1 in]
              n263 = for {
                tunnel: w552 -> [w557] mode=indexing
                shift-right: [w566] -> w550
                shift-left: "" -> [w565]
                tunnel: w549 -> [w562]
                w558 = T5 4 items=["no dialog", "OK message", "continue or stop message", "OK message + warnings", "continue/stop + warnings"] ("type of dialog (OK msg:1)")
                n264 = Path To String(path=w562) -> (string=w561:string)
                n265 = call "Ensight_Format_Check.vi"("Input Number"=w557) -> ("error"=w563:errorcluster, "Output string"=w564:string)  [unwired: 8 in, 1 out]
                n266 = Concatenate Strings("VAR file: " ("error source (\" \")"), w561) -> (w559:string)
                n267 = call <vilib>:"Simple Error Handler.vi"("error source (\" \")"=w559, "type of dialog (OK msg:1)"=w558, "error in (no error)"=w563) -> ()  [unwired: 2 in, 5 out]
                n268 = Concatenate Strings(w565, w564) -> (w566:string)
              }
              n269 = call "Write_File_Simple.vi"("append to file? (new file:F)"=TRUE, "character string"=w550, "file path"=w549) -> ()  [unwired: 2 out]
            }
          }
        }
      }
      frame "End Time" {
        n270 = local write "Position Array (XYZ,spot)"(dbl[][] [] ("Position Array")) -> ()
        n271 = local write "Data Array (spot,Var)"(dbl[][] [] ("Data Array")) -> ()
      }
    }
  }
  "Progress Bar" <- u8 0 ("Progress Bar")
